vi "DetectorTest_MainV11.vi"() -> ()   [LabVIEW 2012]
uses:
  Detector IV/SMU Settings.ctl
  <vilib>/Utility/file.llb/Write To Spreadsheet File (string).vi
  <vilib>/Utility/file.llb/Read From Spreadsheet File (string).vi
  <vilib>/Utility/file.llb/Read From Spreadsheet File (DBL).vi
  <vilib>/Analysis/NI_AALBase.lvlib
panel:
  in  "make common recipe":bool
  in  "select preset recipe":bool
  in  "Detector Measurement Recipe":T1={"Start Voltage"=0.0, "End Voltage"=0.0, "Number of Points"=0.0, "I compliance ma"=0.0, "Sweep Delay s"=0.0, "Direction"="", "Comments"="testing", "Common Recipe"=0.0, "Test Setup"=0.0, "Measurement Recipe ID"=0.0}
  in  "Current Session":timestamp=timestamp(3388091786.578125 s since 1904-01-01)
  in  "new sesh":bool
  out "RecipeID":string="58"
  in  "Sweep Direction (Keysight)":i32(ring) items=["Up", "Down"]
  in  "Auto Adjust Compliance?":bool
  out "Auto Temp Counter":i32
  out "iteration":i32
  in  "Temp Data":T2={"Ambient Temperature"=20.38176242851337, "Chuck Set Temperature"=35.0} {"Chuck Set Temperature" format="%#.1g"; "Ambient Temperature" format="%#.1g"}
  in  "Wafer Info 3":T3={"Cell Name (Automatic)"="Open_Diode_1000", "Package"="", "Coating"="FOR_AIR", "Comment"="IV test for lot 371", "Flash Setup"="5500_99_03p5", "Hrs under test"=0.0}
  out "TempCounter":i32
  out "WaferCounter":i32
  in  "Profile Z":bool
  in  "Load Wafer":bool
  out "Raw Test Skipped":bool=TRUE
  out "device name w skip":string="Open_Diode_1000(skip)"
  in  "4-wire":bool
  out "Laser Counter":i32
  out "Output Power (mW)":dbl
  out "Counter":i32
  out "NameList":string[](array[string])
  in  "Wafer Info Flash 2":T4={"Cell Name"="5500_130_05", "Package"="", "Coating"="", "LRC?"=enum."J2", "Comment"="", "Hours Under Test"=0.0}
  in  "Parameters Flash 2":T5 {"Voc" format="%#_4g"; "Isc" format="%#_4g"; "FF" format="%#_4g"; "Imax" format="%#_4g"; "Vmax" format="%#_4g"; "Pmax" format="%#_4g"; "Itest" format="%#_4g"}
  in  "Wafer Info Flash":T4={"Cell Name"="Open_Diode_1000", "Package"="", "Coating"="", "LRC?"=enum."J2", "Comment"="", "Hours Under Test"=0.0}
  in  "Parameters Flash":T5={"Voc"=0.0, "Isc"=0.0, "FF"=0.0, "Vtest"=0.0, "Imax"=0.0, "Vmax"=0.0, "Pmax"=0.0, "Itest"=0.0, "Efficiency"=0.0, "Incident Power"=5.674, "Power Density (W/cm^2)"=0.6679328011361159, "Cell Area (cm²)"=849486.6535, "Number of AM1.5D Suns"=0.0, "Input Current (mA)"=40.0, "Equivalent 1 sun Jsc"=0.0} {"Voc" format="%#_4g"; "Isc" format="%#_4g"; "FF" format="%#_4g"; "Imax" format="%#_4g"; "Vmax" format="%#_4g"; "Pmax" format="%#_4g"; "Itest" format="%#_4g"}
  out "RawData file":path=path "C:/Users/Flash/Desktop/Data/Detector test data/SJC_ENG_371_4-GaAs/A-3719-2-A/Raw Data/A-3719-2-A_Open_Diode_1000_20180913075240.csv"
  out "Fine Cell Clusters":T6(array[cluster])=[{"Cell Name"="Open_Diode_1000", "X-coord"=46800.0, "Y-coord"=22950.0, "Area"=849486.6535, "Grid Shadowing"=0.0, "Xdim"=500.0, "Ydim"=500.0, "Mesa Area"=785398.1634}]
  out "Selected Data":cluster{dbl[], dbl[]}={[nan, nan, nan, nan, nan, nan, nan, nan, nan, nan, nan, nan, nan, nan, nan, nan, nan, nan, nan, nan, nan, nan, nan, nan, nan, nan, nan, nan, nan, nan, nan, nan, nan, nan, nan, nan, nan, nan, nan, nan, nan, nan, nan, nan, nan, nan, nan, nan, nan, nan, nan, nan, nan, nan, nan, nan, nan, nan, nan, nan, nan, nan, nan, nan, nan, nan, nan, nan, nan, nan, nan, nan, nan, nan, nan, nan, nan, nan, nan, nan, nan, nan, nan, nan], [nan, nan, nan, nan, nan, nan, nan, nan, nan, nan, nan, nan, nan, nan, nan, nan, nan, nan, nan, nan, nan, nan, nan, nan, nan, nan, nan, nan, nan, nan, nan, nan, nan, nan, nan, nan, nan, nan, nan, nan, nan, nan, nan, nan, nan, nan, nan, nan, nan, nan, nan, nan, nan, nan, nan, nan, nan, nan, nan, nan, nan, nan, nan, nan, nan, nan, nan, nan, nan, nan, nan, nan, nan, nan, nan, nan, nan, nan, nan, nan, nan, nan, nan, nan]}
  in  "Test Results 2":T7
  in  "Session Info 2":T8={"V set"=-1.0, "I compliance"=0.001, "J set"=0.01, "I set"=0.0, "V compliance"=1.0, "Laser Power (mW)"=0.0, "TestID"=0, "Session Time"=timestamp(0 s since 1904-01-01), "Operator"="Radek"} {"V compliance" format="%#_6f"; "I compliance" format="%#_6e"}
  in  "Die Info 2":T9={"Device Name"="", "ActiveArea_um2"=3848.451, "MesaArea_um2"=3848.451, "x"=0.0, "y"=0.0}
  in  "Wafer Info 2":T10
  in  "Test Results":T7={"I meas"=-1.83245e-12, "V meas"=6.01176, "Time"=timestamp(3619695820.3512325 s since 1904-01-01)}
  in  "Session Info":T8={"V set"=-6.0, "I compliance"=0.001, "J set"=0.01, "I set"=1.9634954079999997e-05, "V compliance"=6.0, "Laser Power (mW)"=0.0, "TestID"=1794, "Session Time"=timestamp(3619695160.866512 s since 1904-01-01), "Operator"="sswifter"} {"V compliance" format="%#_6f"; "I compliance" format="%#_6e"}
  in  "Die Info":T9={"Device Name"="Open_Diode_1000", "ActiveArea_um2"=849486.6535, "MesaArea_um2"=785398.1634, "x"=26800.0, "y"=72950.0}
  in  "Wafer Info":T10={"Wafer Name"="A-3719-2-A", "Scribe"="BJ325-089", "Mask"="PH001", "Lot"="SJC_ENG_371_4-GaAs"}
  in  "Name Array":string[](array[string])=["Wafer name", "Scribe", "Mask", "Lot", "Device name", "Active Area", "Mesa Area", "x", "y", "Imeas", "Vmeas", "Time", "Vset", "Icomp", "Jset", "Iset", "Vcomp", "Laser Power", "TestID", "SessionTime", "Operator", "Selected"]
  in  "TestID file":path=path "C:/Users/Flash/Documents/GitHub/labview/Detector IV/rawtest_log.csv"
  in  "update wafer":bool
  in  "Lot":string="SJC_ENG_382_4-GaAs"
  in  "Laser Current (mA)":dbl
  in  "Device Name":string="Open_Diode_3000"
  in  "Scribe":string="BP769-030XT"
  in  "MesaArea_um2":dbl=7068583.471
  out "Status":string="idle"
  out "error out":errorcluster
  in  "error in (no error)":errorcluster
  out "Manaul Plot 1":cluster{"V manual":dbl[], dbl[]}[](array[cluster])=[{"V manual"=[-0.1, -0.089741, -0.07949, -0.06923, -0.05897, -0.04872, -0.03846, -0.02821, -0.017951, -0.00769, 0.00256, 0.012819, 0.02308, 0.03333, 0.043589, 0.05385, 0.0641, 0.074359, 0.084619, 0.09487, 0.10513, 0.115379, 0.125639, 0.135899, 0.14615, 0.156409, 0.16667, 0.176919, 0.187179, 0.19744, 0.207691, 0.217949, 0.22821, 0.23846, 0.248719], [2.22891e-05, 1.84968e-05, 1.52529e-05, 1.24377e-05, 1.00378e-05, 7.9393e-06, 6.043e-06, 4.31347e-06, 2.71019e-06, 1.17492e-06, 3.32763e-07, 1.84722e-06, 3.41691e-06, 5.05009e-06, 6.8287e-06, 8.72018e-06, 1.07805e-05, 1.3036e-05, 1.55303e-05, 1.81749e-05, 2.11963e-05, 2.4467e-05, 2.80104e-05, 3.19022e-05, 3.6041e-05, 4.04887e-05, 4.53187e-05, 5.05479e-05, 5.60681e-05, 6.20483e-05, 6.8299e-05, 7.49314e-05, 8.20298e-05, 8.95166e-05, 9.72544e-05]}, {"V manual"=[-0.1, nan, nan, nan, nan, nan, nan, nan, nan, nan, nan, nan, nan, nan, nan, nan, nan, nan, nan, nan, nan, nan, nan, nan, nan, nan, nan, nan, nan, nan, nan, nan, nan, nan, nan, nan, nan, nan, nan, nan], [2.2117733333333333e-05, nan, nan, nan, nan, nan, nan, nan, nan, nan, nan, nan, nan, nan, nan, nan, nan, nan, nan, nan, nan, nan, nan, nan, nan, nan, nan, nan, nan, nan, nan, nan, nan, nan, nan, nan, nan, nan, nan, nan]}, {"V manual"=[0.23860433333333333, nan, nan, nan, nan, nan, nan, nan, nan, nan, nan, nan, nan, nan, nan, nan, nan, nan, nan, nan, nan, nan, nan, nan, nan, nan, nan, nan, nan, nan, nan, nan, nan, nan, nan, nan, nan, nan, nan, nan], [7.068583470999999e-05, nan, nan, nan, nan, nan, nan, nan, nan, nan, nan, nan, nan, nan, nan, nan, nan, nan, nan, nan, nan, nan, nan, nan, nan, nan, nan, nan, nan, nan, nan, nan, nan, nan, nan, nan, nan, nan, nan, nan]}]
  out "Manual Plot 0":cluster{"V manual":dbl[], "I manual":dbl[]}[](array[cluster])=[{"V manual"=[-0.1, -0.089741, -0.07949, -0.06923, -0.05897, -0.04872, -0.03846, -0.02821, -0.017951, -0.00769, 0.00256, 0.012819, 0.02308, 0.03333, 0.043589, 0.05385, 0.0641, 0.074359, 0.084619, 0.09487, 0.10513, 0.115379, 0.125639, 0.135899, 0.14615, 0.156409, 0.16667, 0.176919, 0.187179, 0.19744, 0.207691, 0.217949, 0.22821, 0.23846, 0.248719], "I manual"=[-2.22891e-05, -1.84968e-05, -1.52529e-05, -1.24377e-05, -1.00378e-05, -7.9393e-06, -6.043e-06, -4.31347e-06, -2.71019e-06, -1.17492e-06, 3.32763e-07, 1.84722e-06, 3.41691e-06, 5.05009e-06, 6.8287e-06, 8.72018e-06, 1.07805e-05, 1.3036e-05, 1.55303e-05, 1.81749e-05, 2.11963e-05, 2.4467e-05, 2.80104e-05, 3.19022e-05, 3.6041e-05, 4.04887e-05, 4.53187e-05, 5.05479e-05, 5.60681e-05, 6.20483e-05, 6.8299e-05, 7.49314e-05, 8.20298e-05, 8.95166e-05, 9.72544e-05]}, {"V manual"=[-0.1, nan, nan, nan, nan, nan, nan, nan, nan, nan, nan, nan, nan, nan, nan, nan, nan, nan, nan, nan, nan, nan, nan, nan, nan, nan, nan, nan, nan, nan, nan, nan, nan, nan, nan, nan, nan, nan, nan, nan], "I manual"=[-2.2117733333333333e-05, nan, nan, nan, nan, nan, nan, nan, nan, nan, nan, nan, nan, nan, nan, nan, nan, nan, nan, nan, nan, nan, nan, nan, nan, nan, nan, nan, nan, nan, nan, nan, nan, nan, nan, nan, nan, nan, nan, nan]}, {"V manual"=[0.23860433333333333, nan, nan, nan, nan, nan, nan, nan, nan, nan, nan, nan, nan, nan, nan, nan, nan, nan, nan, nan, nan, nan, nan, nan, nan, nan, nan, nan, nan, nan, nan, nan, nan, nan, nan, nan, nan, nan, nan, nan], "I manual"=[7.068583470999999e-05, nan, nan, nan, nan, nan, nan, nan, nan, nan, nan, nan, nan, nan, nan, nan, nan, nan, nan, nan, nan, nan, nan, nan, nan, nan, nan, nan, nan, nan, nan, nan, nan, nan, nan, nan, nan, nan, nan, nan]}]
  in  "Reset 1st die":bool
  in  "Sweep Settings":T11={"Channel"=enum."Channel A", "Vstart"=-0.1, "Vend"=0.3, "# of points"=40, "NPLC"=1.0, "I compliance"=0.0001, "Delay ms"=100.0}
  in  "Reset xy":bool
  out "current y":i32
  out "current x":i32=10000
  in  "sweep delay ms":dbl=100.0
  in  "I compliance sweep":dbl=0.0001
  in  "points":u16=80
  in  "V end":dbl=1.0
  in  "V start":dbl=-5.0
  in  "Repeat Vf":u32=3
  out "I set":dbl=7.068583470999999e-05
  in  "V compliance":dbl=0.5 format="%#_6f"
  in  "Vf delay ms":dbl=100.0
  in  "J set A/cm2":dbl=0.001
  in  "Repeat Id":u32=5
  in  "I compliance":dbl=0.001 format="%#_6e"
  in  "Id delay ms":dbl=500.0
  in  "V set":dbl=-0.1
  out "Vmeas Settings":T12={"Channel"=enum."Channel A", "Vset"=7.068583470999999e-05, "NPLC"=1.0, "I compliance"=0.3, "Repeat time"=1, "Delay ms"=100.0, "4-wire"=FALSE}
  out "Imeas Settings":T12={"Channel"=enum."Channel A", "Vset"=-0.1, "NPLC"=1.0, "I compliance"=0.001, "Repeat time"=5, "Delay ms"=500.0, "4-wire"=FALSE}
  out "Array of Cell Data Clusters":T13(array[cluster])=[{"Cell Name"="Open_Diode_3000", "X-coord"=0.0, "Y-coord"=0.0, "Area"=7258335.667, "Grid Shadowing"=0.0, "Ydim"=1500.0, "Xdim"=1500.0, "Meas Area"=7068583.471}, {"Cell Name"="Open_Diode_3000", "X-coord"=10000.0, "Y-coord"=0.0, "Area"=7258335.667, "Grid Shadowing"=0.0, "Ydim"=1500.0, "Xdim"=1500.0, "Meas Area"=7068583.471}, {"Cell Name"="Open_Diode_3000", "X-coord"=20000.0, "Y-coord"=0.0, "Area"=7258335.667, "Grid Shadowing"=0.0, "Ydim"=1500.0, "Xdim"=1500.0, "Meas Area"=7068583.471}, {"Cell Name"="Open_Diode_3000", "X-coord"=30000.0, "Y-coord"=0.0, "Area"=7258335.667, "Grid Shadowing"=0.0, "Ydim"=1500.0, "Xdim"=1500.0, "Meas Area"=7068583.471}, {"Cell Name"="Open_Diode_3000", "X-coord"=-10000.0, "Y-coord"=10000.0, "Area"=7258335.667, "Grid Shadowing"=0.0, "Ydim"=1500.0, "Xdim"=1500.0, "Meas Area"=7068583.471}, {"Cell Name"="Open_Diode_3000", "X-coord"=0.0, "Y-coord"=10000.0, "Area"=7258335.667, "Grid Shadowing"=0.0, "Ydim"=1500.0, "Xdim"=1500.0, "Meas Area"=7068583.471}, {"Cell Name"="Open_Diode_3000", "X-coord"=10000.0, "Y-coord"=10000.0, "Area"=7258335.667, "Grid Shadowing"=0.0, "Ydim"=1500.0, "Xdim"=1500.0, "Meas Area"=7068583.471}, {"Cell Name"="Open_Diode_3000", "X-coord"=40000.0, "Y-coord"=10000.0, "Area"=7258335.667, "Grid Shadowing"=0.0, "Ydim"=1500.0, "Xdim"=1500.0, "Meas Area"=7068583.471}, {"Cell Name"="Open_Diode_3000", "X-coord"=-20000.0, "Y-coord"=20000.0, "Area"=7258335.667, "Grid Shadowing"=0.0, "Ydim"=1500.0, "Xdim"=1500.0, "Meas Area"=7068583.471}, {"Cell Name"="Open_Diode_3000", "X-coord"=-10000.0, "Y-coord"=20000.0, "Area"=7258335.667, "Grid Shadowing"=0.0, "Ydim"=1500.0, "Xdim"=1500.0, "Meas Area"=7068583.471}, {"Cell Name"="Open_Diode_3000", "X-coord"=10000.0, "Y-coord"=20000.0, "Area"=7258335.667, "Grid Shadowing"=0.0, "Ydim"=1500.0, "Xdim"=1500.0, "Meas Area"=7068583.471}, {"Cell Name"="Open_Diode_3000", "X-coord"=20000.0, "Y-coord"=20000.0, "Area"=7258335.667, "Grid Shadowing"=0.0, "Ydim"=1500.0, "Xdim"=1500.0, "Meas Area"=7068583.471}, {"Cell Name"="Open_Diode_3000", "X-coord"=40000.0, "Y-coord"=20000.0, "Area"=7258335.667, "Grid Shadowing"=0.0, "Ydim"=1500.0, "Xdim"=1500.0, "Meas Area"=7068583.471}, {"Cell Name"="Open_Diode_3000", "X-coord"=50000.0, "Y-coord"=20000.0, "Area"=7258335.667, "Grid Shadowing"=0.0, "Ydim"=1500.0, "Xdim"=1500.0, "Meas Area"=7068583.471}, {"Cell Name"="Open_Diode_3000", "X-coord"=-20000.0, "Y-coord"=30000.0, "Area"=7258335.667, "Grid Shadowing"=0.0, "Ydim"=1500.0, "Xdim"=1500.0, "Meas Area"=7068583.471}, {"Cell Name"="Open_Diode_3000", "X-coord"=-10000.0, "Y-coord"=30000.0, "Area"=7258335.667, "Grid Shadowing"=0.0, "Ydim"=1500.0, "Xdim"=1500.0, "Meas Area"=7068583.471}, {"Cell Name"="Open_Diode_3000", "X-coord"=20000.0, "Y-coord"=30000.0, "Area"=7258335.667, "Grid Shadowing"=0.0, "Ydim"=1500.0, "Xdim"=1500.0, "Meas Area"=7068583.471}, {"Cell Name"="Open_Diode_3000", "X-coord"=30000.0, "Y-coord"=30000.0, "Area"=7258335.667, "Grid Shadowing"=0.0, "Ydim"=1500.0, "Xdim"=1500.0, "Meas Area"=7068583.471}, {"Cell Name"="Open_Diode_3000", "X-coord"=40000.0, "Y-coord"=30000.0, "Area"=7258335.667, "Grid Shadowing"=0.0, "Ydim"=1500.0, "Xdim"=1500.0, "Meas Area"=7068583.471}, {"Cell Name"="Open_Diode_3000", "X-coord"=50000.0, "Y-coord"=30000.0, "Area"=7258335.667, "Grid Shadowing"=0.0, "Ydim"=1500.0, "Xdim"=1500.0, "Meas Area"=7068583.471}, {"Cell Name"="Open_Diode_3000", "X-coord"=-20000.0, "Y-coord"=40000.0, "Area"=7258335.667, "Grid Shadowing"=0.0, "Ydim"=1500.0, "Xdim"=1500.0, "Meas Area"=7068583.471}, {"Cell Name"="Open_Diode_3000", "X-coord"=-10000.0, "Y-coord"=40000.0, "Area"=7258335.667, "Grid Shadowing"=0.0, "Ydim"=1500.0, "Xdim"=1500.0, "Meas Area"=7068583.471}, {"Cell Name"="Open_Diode_3000", "X-coord"=0.0, "Y-coord"=40000.0, "Area"=7258335.667, "Grid Shadowing"=0.0, "Ydim"=1500.0, "Xdim"=1500.0, "Meas Area"=7068583.471}, {"Cell Name"="Open_Diode_3000", "X-coord"=10000.0, "Y-coord"=40000.0, "Area"=7258335.667, "Grid Shadowing"=0.0, "Ydim"=1500.0, "Xdim"=1500.0, "Meas Area"=7068583.471}, {"Cell Name"="Open_Diode_3000", "X-coord"=40000.0, "Y-coord"=40000.0, "Area"=7258335.667, "Grid Shadowing"=0.0, "Ydim"=1500.0, "Xdim"=1500.0, "Meas Area"=7068583.471}, {"Cell Name"="Open_Diode_3000", "X-coord"=50000.0, "Y-coord"=40000.0, "Area"=7258335.667, "Grid Shadowing"=0.0, "Ydim"=1500.0, "Xdim"=1500.0, "Meas Area"=7068583.471}, {"Cell Name"="Open_Diode_3000", "X-coord"=-20000.0, "Y-coord"=50000.0, "Area"=7258335.667, "Grid Shadowing"=0.0, "Ydim"=1500.0, "Xdim"=1500.0, "Meas Area"=7068583.471}, {"Cell Name"="Open_Diode_3000", "X-coord"=-10000.0, "Y-coord"=50000.0, "Area"=7258335.667, "Grid Shadowing"=0.0, "Ydim"=1500.0, "Xdim"=1500.0, "Meas Area"=7068583.471}, {"Cell Name"="Open_Diode_3000", "X-coord"=10000.0, "Y-coord"=50000.0, "Area"=7258335.667, "Grid Shadowing"=0.0, "Ydim"=1500.0, "Xdim"=1500.0, "Meas Area"=7068583.471}, {"Cell Name"="Open_Diode_3000", "X-coord"=20000.0, "Y-coord"=50000.0, "Area"=7258335.667, "Grid Shadowing"=0.0, "Ydim"=1500.0, "Xdim"=1500.0, "Meas Area"=7068583.471}, {"Cell Name"="Open_Diode_3000", "X-coord"=40000.0, "Y-coord"=50000.0, "Area"=7258335.667, "Grid Shadowing"=0.0, "Ydim"=1500.0, "Xdim"=1500.0, "Meas Area"=7068583.471}, {"Cell Name"="Open_Diode_3000", "X-coord"=50000.0, "Y-coord"=50000.0, "Area"=7258335.667, "Grid Shadowing"=0.0, "Ydim"=1500.0, "Xdim"=1500.0, "Meas Area"=7068583.471}, {"Cell Name"="Open_Diode_3000", "X-coord"=-10000.0, "Y-coord"=60000.0, "Area"=7258335.667, "Grid Shadowing"=0.0, "Ydim"=1500.0, "Xdim"=1500.0, "Meas Area"=7068583.471}, {"Cell Name"="Open_Diode_3000", "X-coord"=20000.0, "Y-coord"=60000.0, "Area"=7258335.667, "Grid Shadowing"=0.0, "Ydim"=1500.0, "Xdim"=1500.0, "Meas Area"=7068583.471}, {"Cell Name"="Open_Diode_3000", "X-coord"=30000.0, "Y-coord"=60000.0, "Area"=7258335.667, "Grid Shadowing"=0.0, "Ydim"=1500.0, "Xdim"=1500.0, "Meas Area"=7068583.471}, {"Cell Name"="Open_Diode_3000", "X-coord"=40000.0, "Y-coord"=60000.0, "Area"=7258335.667, "Grid Shadowing"=0.0, "Ydim"=1500.0, "Xdim"=1500.0, "Meas Area"=7068583.471}, {"Cell Name"="Open_Diode_3000", "X-coord"=0.0, "Y-coord"=70000.0, "Area"=7258335.667, "Grid Shadowing"=0.0, "Ydim"=1500.0, "Xdim"=1500.0, "Meas Area"=7068583.471}, {"Cell Name"="Open_Diode_3000", "X-coord"=10000.0, "Y-coord"=70000.0, "Area"=7258335.667, "Grid Shadowing"=0.0, "Ydim"=1500.0, "Xdim"=1500.0, "Meas Area"=7068583.471}, {"Cell Name"="Open_Diode_3000", "X-coord"=20000.0, "Y-coord"=70000.0, "Area"=7258335.667, "Grid Shadowing"=0.0, "Ydim"=1500.0, "Xdim"=1500.0, "Meas Area"=7068583.471}, {"Cell Name"="Open_Diode_3000", "X-coord"=30000.0, "Y-coord"=70000.0, "Area"=7258335.667, "Grid Shadowing"=0.0, "Ydim"=1500.0, "Xdim"=1500.0, "Meas Area"=7068583.471}]
  in  "stop":bool
  in  "ActiveArea_um2":dbl=7258335.667
  in  "NPLC":dbl=1.0
  in  "Operator":string(combo)="tbilir"
  in  "Mask":string="PH001"
  in  "Wafer Name":string="A-3820-3-A"
  in  "Tab Control":T14(tab)
  in  "First Wafer Loaded?":bool
  in  "begin lot test":bool
  in  "Desired Wafer Name":string
  in  "Wafer List":i32(listbox)=-1
  in  "Add to wafer list":bool
  in  "Remove from wafer list":bool
  in  "Clear wafer list":bool
  in  "Generate Report":bool
  in  "Only Raw Test":bool
  in  "Clear Laser List":bool
  in  "Remove from Laser List":bool
  in  "Add to Laser":bool
  in  "Desired Current (mA)":dbl=40.0
  in  "Laser List":i32(listbox)=-1
  in  "Start auto":bool
  in  "Clear List":bool
  in  "Refresh Device":bool
  in  "Mask Name":string
  in  "Remove from List":bool
  in  "Add to list":bool
  in  "Available Device Name":string(combo)="Open_Diode_1000"
  in  "Test List":i32(listbox)=-1
  in  "Mask File all":path=path "C:/Users/Flash/Desktop/Mask Files/PH001 Detector GSG/PH001_Detector Aligner mask map file _ full top_open top 10_open top 5 diodes.csv"
  in  "Skip Raw Test?":bool
  in  "Test description":string="IV test for lot 371"
  in  "Clear temp list Auto":bool
  in  "Remove from Temp Auto":bool
  in  "Add to Temp Auto":bool
  in  "Auto Temp Set":dbl=25.0
  in  "Auto Temperature List":i32(listbox)=-1
  in  "Manual_Test":bool
  in  "Manual IV Plot settting":enum32{"Linear plot", "Log plot"}(radio)
  out "Vmeas manual":dbl=0.23860433333333333
  out "Imeas manual":dbl=-2.2117733333333333e-05
  out "Iarray manual":dbl[](array[numeric])=[-2.22891e-05, -1.84968e-05, -1.52529e-05, -1.24377e-05, -1.00378e-05, -7.9393e-06, -6.043e-06, -4.31347e-06, -2.71019e-06, -1.17492e-06, 3.32763e-07, 1.84722e-06, 3.41691e-06, 5.05009e-06, 6.8287e-06, 8.72018e-06, 1.07805e-05, 1.3036e-05, 1.55303e-05, 1.81749e-05, 2.11963e-05, 2.4467e-05, 2.80104e-05, 3.19022e-05, 3.6041e-05, 4.04887e-05, 4.53187e-05, 5.05479e-05, 5.60681e-05, 6.20483e-05, 6.8299e-05, 7.49314e-05, 8.20298e-05, 8.95166e-05, 9.72544e-05]
  out "Varray manual":dbl[](array[numeric])=[-0.1, -0.089741, -0.07949, -0.06923, -0.05897, -0.04872, -0.03846, -0.02821, -0.017951, -0.00769, 0.00256, 0.012819, 0.02308, 0.03333, 0.043589, 0.05385, 0.0641, 0.074359, 0.084619, 0.09487, 0.10513, 0.115379, 0.125639, 0.135899, 0.14615, 0.156409, 0.16667, 0.176919, 0.187179, 0.19744, 0.207691, 0.217949, 0.22821, 0.23846, 0.248719]
  out "y target":i32
  out "x target":i32=10000
  in  "Die Number":u16(ring)=1 items=["0", "1", "2", "3", "4", "5", "6", "7", "8", "9", "10", "11", "12", "13", "14", "15", "16", "17", "18", "19", "20", "21", "22", "23", "24", "25", "26", "27", "28", "29", "30", "31", "32", "33", "34", "35", "36", "37", "38", "39", "40", "41", "42", "43", "44", "45", "46", "47", "48", "49", "50", "51", "52", "53", "54", "55", "56", "57", "58", "59", "60", "61", "62", "63", "64", "65", "66", "67", "68", "69", "70", "71", "72", "73", "74", "75", "76", "77", "78", "79", "80", "81", "82", "83", "84", "85"]
  in  "load file":bool
  in  "Move to":bool
  in  "Mask File Manual":path=path "C:/Users/Flash/Desktop/Mask Files/PH001 Detector GSG/PH001_Detector Aligner mask map file _ full top_open top 10_open top 5 diodes_Open_Diode_3000.csv"
  out "Manual IV":cluster{"V manual":dbl[], "I manual":dbl[]}[](graph)=[{"V manual"=[-0.1, -0.089741, -0.07949, -0.06923, -0.05897, -0.04872, -0.03846, -0.02821, -0.017951, -0.00769, 0.00256, 0.012819, 0.02308, 0.03333, 0.043589, 0.05385, 0.0641, 0.074359, 0.084619, 0.09487, 0.10513, 0.115379, 0.125639, 0.135899, 0.14615, 0.156409, 0.16667, 0.176919, 0.187179, 0.19744, 0.207691, 0.217949, 0.22821, 0.23846, 0.248719], "I manual"=[-2.22891e-05, -1.84968e-05, -1.52529e-05, -1.24377e-05, -1.00378e-05, -7.9393e-06, -6.043e-06, -4.31347e-06, -2.71019e-06, -1.17492e-06, 3.32763e-07, 1.84722e-06, 3.41691e-06, 5.05009e-06, 6.8287e-06, 8.72018e-06, 1.07805e-05, 1.3036e-05, 1.55303e-05, 1.81749e-05, 2.11963e-05, 2.4467e-05, 2.80104e-05, 3.19022e-05, 3.6041e-05, 4.04887e-05, 4.53187e-05, 5.05479e-05, 5.60681e-05, 6.20483e-05, 6.8299e-05, 7.49314e-05, 8.20298e-05, 8.95166e-05, 9.72544e-05]}, {"V manual"=[-0.1, nan, nan, nan, nan, nan, nan, nan, nan, nan, nan, nan, nan, nan, nan, nan, nan, nan, nan, nan, nan, nan, nan, nan, nan, nan, nan, nan, nan, nan, nan, nan, nan, nan, nan, nan, nan, nan, nan, nan], "I manual"=[-2.2117733333333333e-05, nan, nan, nan, nan, nan, nan, nan, nan, nan, nan, nan, nan, nan, nan, nan, nan, nan, nan, nan, nan, nan, nan, nan, nan, nan, nan, nan, nan, nan, nan, nan, nan, nan, nan, nan, nan, nan, nan, nan]}, {"V manual"=[0.23860433333333333, nan, nan, nan, nan, nan, nan, nan, nan, nan, nan, nan, nan, nan, nan, nan, nan, nan, nan, nan, nan, nan, nan, nan, nan, nan, nan, nan, nan, nan, nan, nan, nan, nan, nan, nan, nan, nan, nan, nan], "I manual"=[7.068583470999999e-05, nan, nan, nan, nan, nan, nan, nan, nan, nan, nan, nan, nan, nan, nan, nan, nan, nan, nan, nan, nan, nan, nan, nan, nan, nan, nan, nan, nan, nan, nan, nan, nan, nan, nan, nan, nan, nan, nan, nan]}]
  in  "Measure 2 Point?":bool=TRUE
  in  "Manual Test Comments":string="IV test for lot 371"
  in  "Load raw":bool
  in  "Select":bool
  in  "Number Select":u16=10
  in  "Vmax":dbl=0.285
  in  "Vmin":dbl=0.05
  out "Test FileName":string="A-3719-2-A_Open_Diode_1000_20180913075240.csv"
  out "RawTest ID":u32=2029
  out "Progress":u8(slide)=99 scale=0.0..100.0
  out "Current Device":u32=84
  out "Total Device":u32=84
  out "V meas":dbl[](array[numeric])=[6.01142, 6.01054, 6.01089, 0.000137925, 6.01222, 6.01216, 6.01145, 6.01193, 6.0103, 6.01103, 6.01162, 6.01132, 6.01127, 6.01137, 6.01132, 6.01125, 6.01108, 6.01134, 6.01154, 6.01135, 6.01146, 6.01204, 6.01111, 6.01101, 6.01053, 6.01143, 6.01152, 6.01128, 6.00993, 6.00994, 6.01042, 3.58707, 6.01175, 6.01164, 6.01056, 6.01166, 6.01073, 6.01098, 6.01142, 6.01026, 6.01071, 6.01116, 6.01174, 6.01214, 6.01026, 6.01093, 5.99486, 6.01138, 6.01091, 6.01133, 6.01086, 6.01094, 6.01192, 6.01232, 6.01069, 6.01162, 6.01233, 6.01184, 6.0022, 5.17964, 6.01156, 6.01223, 6.01107, 6.0102, 6.0108, 6.01164, 5.75188, 5.06441, 6.01144, 6.01129, 6.01161, 6.01159, 6.01096, 5.61419, 5.16536, 6.01197, 6.01142, 6.01186, 6.01133, 6.01132, 6.01119, 6.01113, 5.83632, 6.01176]
  out "I meas":dbl[](array[numeric])=[-3.868033999999999e-11, -1.2052780000000002e-09, -6.028065999999999e-11, -0.0009999796, -3.0170019999999996e-11, -4.752688e-11, -4.8625459999999994e-11, -3.7159980000000005e-11, -1.7203160000000002e-07, -2.00883e-08, -7.974548e-11, -3.897576e-11, -3.555112e-11, -2.188194e-08, -5.2771619999999994e-11, -2.9935519999999994e-11, -3.295828e-11, -5.707007999999999e-08, -4.796104e-07, -2.002028e-08, -7.080146e-08, -4.18e-11, -2.108774e-11, -4.09959e-11, -4.424556e-11, -3.3264100000000003e-09, -2.0351338000000002e-10, -6.144901999999999e-09, -4.3002719999999993e-11, -3.898936e-09, -2.0389360000000002e-11, -2.049748e-08, -6.527374000000001e-10, -1.0336196000000001e-10, -2.697004e-11, -3.376518e-08, -6.171924e-11, -2.02069e-10, -1.200538e-09, -2.8179300000000003e-11, -6.537938e-10, -5.153115999999999e-11, -2.8508420000000003e-09, -7.534774e-07, -2.636916e-07, -1.446754e-09, -9.464432000000001e-11, -1.0602588000000001e-10, -4.217728e-11, -7.227086e-08, -3.990094e-11, -2.7389038000000002e-11, -1.90881e-07, -2.2892700000000004e-12, -4.745506e-08, -4.579318e-11, -4.5842860000000003e-11, -5.953868e-11, -3.758154e-11, -4.4363539999999995e-09, -7.143562e-11, -1.397812e-10, -7.11463e-11, -5.56664e-11, -2.6296820000000003e-08, -1.1582659999999999e-07, -2.317642e-11, -5.807276000000001e-11, -2.17813e-12, -5.7970201999999995e-11, -6.71486e-11, -8.667722000000001e-12, 3.2483739999999993e-12, -6.306573999999999e-11, -8.307524e-11, -2.4324079999999998e-12, -2.795726e-12, -2.185576e-12, -2.0225460000000002e-12, -2.122472e-12, -1.6340760000000001e-06, -2.5727129999999997e-06, -3.269066e-11, -1.83245e-12]
  in  "RawData Save Path":path=path "C:/Users/Flash/Desktop/Data/Detector test data"
  in  "StartRaw":bool
  out "Vforward hist":T15(graph)={"X Values"=[0.30074752875, 0.90196673625, 1.5031859437500001, 2.10440515125, 2.70562435875, 3.3068435662500004, 3.90806277375, 4.50928198125, 5.110501188750001, 5.7117203962500005], "Histogram: h(x)"=[1, 0, 0, 0, 0, 1, 0, 0, 3, 79]}
  out "Idark hist":T15(graph)={"X Values"=[-0.0009499806198375813, -0.0008499826595127439, -0.0007499846991879066, -0.0006499867388630691, -0.0005499887785382317, -0.0004499908182133943, -0.0003499928578885569, -0.0002499948975637195, -0.0001499969372388821, -4.99989769140447e-05], "Histogram: h(x)"=[1, 0, 0, 0, 0, 0, 0, 0, 0, 83]}
  in  "Mask File Raw":path=path "C:/Users/Flash/Desktop/Mask Files/PH001 Detector GSG/PH001_Detector Aligner mask map file _ full top_open top 10_open top 5 diodes_Open_Diode_3000.csv"
  out "Spec Plot":cluster{"V meas":dbl[], "I meas":dbl[]}[](graph)=[{"V meas"=[6.01142, 6.01054, 6.01089, 0.000137925, 6.01222, 6.01216, 6.01145, 6.01193, 6.0103, 6.01103, 6.01162, 6.01132, 6.01127, 6.01137, 6.01132, 6.01125, 6.01108, 6.01134, 6.01154, 6.01135, 6.01146, 6.01204, 6.01111, 6.01101, 6.01053, 6.01143, 6.01152, 6.01128, 6.00993, 6.00994, 6.01042, 3.58707, 6.01175, 6.01164, 6.01056, 6.01166, 6.01073, 6.01098, 6.01142, 6.01026, 6.01071, 6.01116, 6.01174, 6.01214, 6.01026, 6.01093, 5.99486, 6.01138, 6.01091, 6.01133, 6.01086, 6.01094, 6.01192, 6.01232, 6.01069, 6.01162, 6.01233, 6.01184, 6.0022, 5.17964, 6.01156, 6.01223, 6.01107, 6.0102, 6.0108, 6.01164, 5.75188, 5.06441, 6.01144, 6.01129, 6.01161, 6.01159, 6.01096, 5.61419, 5.16536, 6.01197, 6.01142, 6.01186, 6.01133, 6.01132, 6.01119, 6.01113, 5.83632, 6.01176], "I meas"=[-3.868033999999999e-11, -1.2052780000000002e-09, -6.028065999999999e-11, -0.0009999796, -3.0170019999999996e-11, -4.752688e-11, -4.8625459999999994e-11, -3.7159980000000005e-11, -1.7203160000000002e-07, -2.00883e-08, -7.974548e-11, -3.897576e-11, -3.555112e-11, -2.188194e-08, -5.2771619999999994e-11, -2.9935519999999994e-11, -3.295828e-11, -5.707007999999999e-08, -4.796104e-07, -2.002028e-08, -7.080146e-08, -4.18e-11, -2.108774e-11, -4.09959e-11, -4.424556e-11, -3.3264100000000003e-09, -2.0351338000000002e-10, -6.144901999999999e-09, -4.3002719999999993e-11, -3.898936e-09, -2.0389360000000002e-11, -2.049748e-08, -6.527374000000001e-10, -1.0336196000000001e-10, -2.697004e-11, -3.376518e-08, -6.171924e-11, -2.02069e-10, -1.200538e-09, -2.8179300000000003e-11, -6.537938e-10, -5.153115999999999e-11, -2.8508420000000003e-09, -7.534774e-07, -2.636916e-07, -1.446754e-09, -9.464432000000001e-11, -1.0602588000000001e-10, -4.217728e-11, -7.227086e-08, -3.990094e-11, -2.7389038000000002e-11, -1.90881e-07, -2.2892700000000004e-12, -4.745506e-08, -4.579318e-11, -4.5842860000000003e-11, -5.953868e-11, -3.758154e-11, -4.4363539999999995e-09, -7.143562e-11, -1.397812e-10, -7.11463e-11, -5.56664e-11, -2.6296820000000003e-08, -1.1582659999999999e-07, -2.317642e-11, -5.807276000000001e-11, -2.17813e-12, -5.7970201999999995e-11, -6.71486e-11, -8.667722000000001e-12, 3.2483739999999993e-12, -6.306573999999999e-11, -8.307524e-11, -2.4324079999999998e-12, -2.795726e-12, -2.185576e-12, -2.0225460000000002e-12, -2.122472e-12, -1.6340760000000001e-06, -2.5727129999999997e-06, -3.269066e-11, -1.83245e-12]}, {"V meas"=[3.58707, nan, nan, nan, nan, nan, nan, nan, nan, nan, nan, nan, nan, nan, nan, nan, nan, nan, nan, nan, nan, nan, nan, nan, nan, nan, nan, nan, nan, nan, nan, nan, nan, nan, nan, nan, nan, nan, nan, nan, nan, nan, nan, nan, nan, nan, nan, nan, nan, nan, nan, nan, nan, nan, nan, nan, nan, nan, nan, nan, nan, nan, nan, nan, nan, nan, nan, nan, nan, nan, nan, nan, nan, nan, nan, nan, nan, nan, nan, nan, nan, nan, nan, nan], "I meas"=[-2.049748e-08, nan, nan, nan, nan, nan, nan, nan, nan, nan, nan, nan, nan, nan, nan, nan, nan, nan, nan, nan, nan, nan, nan, nan, nan, nan, nan, nan, nan, nan, nan, nan, nan, nan, nan, nan, nan, nan, nan, nan, nan, nan, nan, nan, nan, nan, nan, nan, nan, nan, nan, nan, nan, nan, nan, nan, nan, nan, nan, nan, nan, nan, nan, nan, nan, nan, nan, nan, nan, nan, nan, nan, nan, nan, nan, nan, nan, nan, nan, nan, nan, nan, nan, nan]}]
  in  "Explore Data":bool
  out "no file":bool
  in  "Comments":string="IV test for lot 371"
  in  "FineTest save path":path=path "C:/Users/Flash/Desktop/Data/Detector test data"
  out "I fine":dbl[](array[numeric])=[-2.70504e-08, -2.32087e-08, -1.94015e-08, -1.62001e-08, -1.3396e-08, -1.06144e-08, -8.14274e-09, -5.83125e-09, -3.66964e-09, -2.05099e-09, -1.05505e-09, -6.56038e-10, -4.43558e-10, -3.24538e-10, -2.3071e-10, -1.84326e-10, -1.50747e-10, -1.31042e-10, -1.1589e-10, -1.0217e-10, -9.29752e-11, -8.22993e-11, -7.74358e-11, -6.84813e-11, -6.19634e-11, -5.51294e-11, -4.86827e-11, -4.15262e-11, -3.40749e-11, -2.82174e-11, -2.14966e-11, -1.33787e-11, -7.37435e-12, -5.50663e-12, 4.69868e-12, 1.38179e-11, 4.52471e-11, 2.99241e-10, 1.96981e-09, 2.81104e-08]
  out "V fine":dbl[](array[numeric])=[-6.0, -5.82051, -5.64103, -5.46154, -5.28205, -5.10256, -4.92308, -4.74359, -4.5641, -4.38461, -4.20513, -4.02564, -3.84615, -3.66667, -3.48718, -3.30769, -3.1282, -2.94872, -2.76923, -2.58974, -2.41026, -2.23077, -2.05128, -1.87179, -1.69231, -1.51282, -1.33333, -1.15384, -0.974358, -0.79487, -0.615383, -0.435896, -0.256409, -0.0769218, 0.102565, 0.282053, 0.46154, 0.641027, 0.820514, 1.0]
  out "Current Device":u32=1
  out "Total Device":u32=1
  out "IV fine log":cluster{dbl[], dbl[]}[](graph)=[{[-6.0, -5.82051, -5.64103, -5.46154, -5.28205, -5.10256, -4.92308, -4.74359, -4.5641, -4.38461, -4.20513, -4.02564, -3.84615, -3.66667, -3.48718, -3.30769, -3.1282, -2.94872, -2.76923, -2.58974, -2.41026, -2.23077, -2.05128, -1.87179, -1.69231, -1.51282, -1.33333, -1.15384, -0.974358, -0.79487, -0.615383, -0.435896, -0.256409, -0.0769218, 0.102565, 0.282053, 0.46154, 0.641027, 0.820514, 1.0], [2.70504e-08, 2.32087e-08, 1.94015e-08, 1.62001e-08, 1.3396e-08, 1.06144e-08, 8.14274e-09, 5.83125e-09, 3.66964e-09, 2.05099e-09, 1.05505e-09, 6.56038e-10, 4.43558e-10, 3.24538e-10, 2.3071e-10, 1.84326e-10, 1.50747e-10, 1.31042e-10, 1.1589e-10, 1.0217e-10, 9.29752e-11, 8.22993e-11, 7.74358e-11, 6.84813e-11, 6.19634e-11, 5.51294e-11, 4.86827e-11, 4.15262e-11, 3.40749e-11, 2.82174e-11, 2.14966e-11, 1.33787e-11, 7.37435e-12, 5.50663e-12, 4.69868e-12, 1.38179e-11, 4.52471e-11, 2.99241e-10, 1.96981e-09, 2.81104e-08]}]
  out "Progress 2":u8(slide)=100 scale=0.0..100.0
  in  "StartFine":bool
  out "IV fine linear":cluster{dbl[], dbl[]}[](graph)=[{[-6.0, -5.82051, -5.64103, -5.46154, -5.28205, -5.10256, -4.92308, -4.74359, -4.5641, -4.38461, -4.20513, -4.02564, -3.84615, -3.66667, -3.48718, -3.30769, -3.1282, -2.94872, -2.76923, -2.58974, -2.41026, -2.23077, -2.05128, -1.87179, -1.69231, -1.51282, -1.33333, -1.15384, -0.974358, -0.79487, -0.615383, -0.435896, -0.256409, -0.0769218, 0.102565, 0.282053, 0.46154, 0.641027, 0.820514, 1.0], [-2.70504e-08, -2.32087e-08, -1.94015e-08, -1.62001e-08, -1.3396e-08, -1.06144e-08, -8.14274e-09, -5.83125e-09, -3.66964e-09, -2.05099e-09, -1.05505e-09, -6.56038e-10, -4.43558e-10, -3.24538e-10, -2.3071e-10, -1.84326e-10, -1.50747e-10, -1.31042e-10, -1.1589e-10, -1.0217e-10, -9.29752e-11, -8.22993e-11, -7.74358e-11, -6.84813e-11, -6.19634e-11, -5.51294e-11, -4.86827e-11, -4.15262e-11, -3.40749e-11, -2.82174e-11, -2.14966e-11, -1.33787e-11, -7.37435e-12, -5.50663e-12, 4.69868e-12, 1.38179e-11, 4.52471e-11, 2.99241e-10, 1.96981e-09, 2.81104e-08]}]
  in  "Mask File Fine":path=path "C:/Users/Flash/Desktop/Data/Detector test data/SJC_ENG_371_4-GaAs/A-3719-2-A/Raw Data/PH001_Detector Aligner mask map file _ full top_open top 10_open top 5 diodes_Open_Diode_1000_A-3719-2-A_091318_080341.5AM.csv"
  out "Y":dbl
  out "X":dbl
  in  "move prober 2":bool
  in  "load file for temp series":bool
  in  "Mask File Temperature":path=path "C:/Users/Flash/Desktop/Data/Detector test data/PH001 Detector Aligner mask map file _ full top_open top 10_open top 5 diodes_Open_Diode_5_300_A-3605-1-A_052518_113739.0AM.csv"
  out "IV temp linear":cluster{dbl[], dbl[]}[](graph)
  in  "Start temp":bool
  out "IV temp log":cluster{dbl[], dbl[]}[](graph)
  out "V fine temp":dbl[](array[numeric])=[-1.5, -1.45128, -1.40256, -1.35385, -1.30513, -1.25641, -1.20769, -1.15897, -1.11026, -1.06154, -1.01282, -0.964102, -0.915384, -0.866666, -0.817948, -0.76923, -0.720512, -0.671794, -0.623076, -0.574358, -0.52564, -0.476923, -0.428205, -0.379487, -0.330769, -0.282051, -0.233333, -0.184615, -0.135897, -0.087179, -0.038461, 0.0102569, 0.0589749, 0.107693, 0.156411, 0.205129, 0.253847, 0.302565, 0.351283, 0.400001]
  out "I fine temp":dbl[](array[numeric])=[-1.28772e-07, -1.20805e-07, -1.15592e-07, -1.10987e-07, -1.06412e-07, -1.02022e-07, -4.62038e-08, -9.34188e-08, -8.97462e-08, -8.60003e-08, -8.23237e-08, -7.87101e-08, -7.52945e-08, -7.18306e-08, -6.85145e-08, -6.5287e-08, -6.2088e-08, -5.90038e-08, -5.59938e-08, -5.29941e-08, -5.00661e-08, -4.71812e-08, -4.43421e-08, -4.15389e-08, -3.87298e-08, -3.5945e-08, -3.31511e-08, -3.027e-08, -2.71168e-08, -2.30654e-08, -1.54139e-08, 7.82768e-09, 2.30625e-07, 5.07951e-07, 2.21662e-06, 9.15235e-06, 3.37902e-05, 9.47719e-05, 0.000202989, 0.000357986]
  in  "Temperature Series save path":path=path "C:/Users/Flash/Desktop/Data/Detector test data"
  in  "Comments Temp":string
  in  "Single Device Temperature List":i32(listbox)=-1
  in  "Desired Temperature":dbl=25.0
  in  "Add to Temp":bool
  in  "Remove from Temp":bool
  in  "Clear temp list":bool
  in  "Desired Device":u16(ring)=50 items=["0", "1", "2", "3", "4", "5", "6", "7", "8", "9"]
  in  "Channel Keysight":dbl
  in  "Keysight SMU":refnum<visa-resource-name>="GPIB0::23::INSTR"
  in  "update temp":bool
  out "Current Temp":string="0\r"
  in  "Temp Setpoint":string="25"
  in  "Temptronics VISA":refnum<visa-resource-name>="GPIB0::9::INSTR"
  in  "Prober GPIB":string="0:1"
  in  "Keithley SMU":refnum<visa-resource-name>="GPIB0::26::INSTR"
  in  "Channel":enum32{"Channel A", "Channel B"}(ring)
  out "Calibration":cluster{"Y":dbl[], "Y":dbl[]}[](graph)=[{"Y"=[0.1, 0.2, 0.3, 0.4, 0.5, 0.6, 0.7, 0.8, 0.9, 1.0, 1.1, 1.2, 1.3, 1.4, 1.5, 1.6, 1.7, 1.8, 1.9, 2.0, 2.1, 2.2, 2.3, 2.4, 2.5, 2.6, 2.7, 2.8, 2.9, 3.0, 3.1, 3.2, 3.3, 3.4, 3.5, 3.6, 3.7, 3.8, 3.9, 4.0, 4.1, 4.2, 4.3, 4.4, 4.5, 4.6, 4.7, 4.8, 4.9, 5.0, 5.1, 5.2, 5.3, 5.4, 5.5, 5.6, 5.7, 5.8, 5.9, 6.0, 6.1, 6.2, 6.3, 6.4, 6.5, 6.6, 6.7, 6.8, 6.9, 7.0, 7.1, 7.2, 7.3, 7.4, 7.5, 7.6, 7.7, 7.8, 7.9, 8.0, 8.1, 8.2, 8.3, 8.4, 8.5, 8.6, 8.7, 8.8, 8.9, 9.0, 9.1, 9.2, 9.3, 9.4, 9.5, 9.6, 9.7, 9.8, 9.9, 10.0, 10.1, 10.2, 10.3, 10.4, 10.5, 10.6, 10.7, 10.8, 10.9, 11.0, 11.1, 11.2, 11.3, 11.4, 11.5, 11.6, 11.7, 11.8, 11.9, 12.0, 12.1, 12.2, 12.3, 12.4, 12.5, 12.6, 12.7, 12.8, 12.9, 13.0, 13.1, 13.2, 13.3, 13.4, 13.5, 13.6, 13.7, 13.8, 13.9, 14.0, 14.1, 14.2, 14.3, 14.4, 14.5, 14.6, 14.7, 14.8, 14.9, 15.0, 15.1, 15.2, 15.3, 15.4, 15.5, 15.6, 15.7, 15.8, 15.9, 16.0, 16.1, 16.2, 16.3, 16.4, 16.5, 16.6, 16.7, 16.8, 16.9, 17.0, 17.1, 17.2, 17.3, 17.4, 17.5, 17.6, 17.7, 17.8, 17.9, 18.0, 18.1, 18.2, 18.3, 18.4, 18.5, 18.6, 18.7, 18.8, 18.9, 19.0, 19.1, 19.2, 19.3, 19.4, 19.5, 19.6, 19.7, 19.8, 19.9, 20.0, 20.1, 20.2, 20.3, 20.4, 20.5, 20.6, 20.7, 20.8, 20.9, 21.0, 21.1, 21.2, 21.3, 21.4, 21.5, 21.6, 21.7, 21.8, 21.9, 22.0, 22.1, 22.2, 22.3, 22.4, 22.5, 22.6, 22.7, 22.8, 22.9, 23.0, 23.1, 23.2, 23.3, 23.4, 23.5, 23.6, 23.7, 23.8, 23.9, 24.0, 24.1, 24.2, 24.3, 24.4, 24.5, 24.6, 24.7, 24.8, 24.9, 25.0, 25.1, 25.2, 25.3, 25.4, 25.5, 25.6, 25.7, 25.8, 25.9, 26.0, 26.1, 26.2, 26.3, 26.4, 26.5, 26.6, 26.7, 26.8, 26.9, 27.0, 27.1, 27.2, 27.3, 27.4, 27.5, 27.6, 27.7, 27.8, 27.9, 28.0, 28.1, 28.2, 28.3, 28.4, 28.5, 28.6, 28.7, 28.8, 28.9, 29.0, 29.1, 29.2, 29.3, 29.4, 29.5, 29.6, 29.7, 29.8, 29.9, 30.0, 30.1, 30.2, 30.3, 30.4, 30.5, 30.6, 30.7, 30.8, 30.9, 31.0, 31.1, 31.2, 31.3, 31.4, 31.5, 31.6, 31.7, 31.8, 31.9, 32.0, 32.1, 32.2, 32.3, 32.4, 32.5, 32.6, 32.7, 32.8, 32.9, 33.0, 33.1, 33.2, 33.3, 33.4, 33.5, 33.6, 33.7, 33.8, 33.9, 34.0, 34.1, 34.2, 34.3, 34.4, 34.5, 34.6, 34.7, 34.8, 34.9, 35.0, 35.1, 35.2, 35.3, 35.4, 35.5, 35.6, 35.7, 35.8, 35.9, 36.0, 36.1, 36.2, 36.3, 36.4, 36.5, 36.6, 36.7, 36.8, 36.9, 37.0, 37.1, 37.2, 37.3, 37.4, 37.5, 37.6, 37.7, 37.8, 37.9, 38.0, 38.1, 38.2, 38.3, 38.4, 38.5, 38.6, 38.7, 38.8, 38.9, 39.0, 39.1, 39.2, 39.3, 39.4, 39.5, 39.6, 39.7, 39.8, 39.9, 40.0], "Y"=[0.0, 0.0, 0.0, 0.0, 0.0, 0.0, 0.0, 0.0, 0.0, 0.0, 0.0, 0.0, 0.0, 0.0, 0.0, 0.0, 0.0, 0.001, 0.001, 0.001, 0.001, 0.001, 0.001, 0.001, 0.001, 0.001, 0.001, 0.001, 0.001, 0.001, 0.001, 0.001, 0.001, 0.002, 0.002, 0.002, 0.002, 0.002, 0.002, 0.002, 0.002, 0.002, 0.002, 0.003, 0.003, 0.003, 0.003, 0.003, 0.003, 0.004, 0.004, 0.004, 0.004, 0.004, 0.005, 0.005, 0.005, 0.005, 0.006, 0.006, 0.006, 0.007, 0.007, 0.007, 0.008, 0.008, 0.008, 0.009, 0.009, 0.01, 0.01, 0.011, 0.011, 0.012, 0.012, 0.013, 0.013, 0.014, 0.015, 0.016, 0.017, 0.019, 0.023, 0.037, 0.058, 0.075, 0.091, 0.109, 0.127, 0.149, 0.168, 0.185, 0.202, 0.22, 0.243, 0.261, 0.279, 0.297, 0.314, 0.332, 0.354, 0.372, 0.391, 0.409, 0.427, 0.449, 0.466, 0.485, 0.503, 0.522, 0.544, 0.561, 0.579, 0.597, 0.615, 0.633, 0.658, 0.674, 0.692, 0.71, 0.728, 0.751, 0.768, 0.787, 0.807, 0.824, 0.845, 0.862, 0.88, 0.899, 0.918, 0.933, 0.957, 0.976, 0.993, 1.012, 1.029, 1.051, 1.07, 1.089, 1.103, 1.124, 1.145, 1.165, 1.183, 1.202, 1.217, 1.239, 1.256, 1.276, 1.294, 1.315, 1.333, 1.356, 1.376, 1.389, 1.405, 1.43, 1.45, 1.467, 1.485, 1.508, 1.524, 1.546, 1.56, 1.579, 1.598, 1.614, 1.631, 1.656, 1.679, 1.695, 1.715, 1.731, 1.75, 1.769, 1.791, 1.801, 1.824, 1.84, 1.865, 1.881, 1.897, 1.912, 1.93, 1.953, 1.974, 1.993, 2.006, 2.028, 2.052, 2.073, 2.087, 2.105, 2.125, 2.146, 2.164, 2.186, 2.203, 2.213, 2.243, 2.258, 2.276, 2.296, 2.311, 2.328, 2.35, 2.366, 2.389, 2.412, 2.426, 2.45, 2.459, 2.476, 2.502, 2.522, 2.53, 2.561, 2.571, 2.593, 2.609, 2.626, 2.652, 2.666, 2.691, 2.704, 2.729, 2.74, 2.764, 2.782, 2.807, 2.817, 2.837, 2.854, 2.869, 2.886, 2.908, 2.937, 2.947, 2.979, 2.988, 3.002, 3.033, 3.043, 3.064, 3.075, 3.1, 3.111, 3.145, 3.156, 3.181, 3.196, 3.212, 3.232, 3.246, 3.273, 3.289, 3.299, 3.327, 3.35, 3.371, 3.374, 3.4, 3.418, 3.45, 3.462, 3.483, 3.499, 3.516, 3.531, 3.55, 3.564, 3.592, 3.608, 3.629, 3.662, 3.674, 3.693, 3.717, 3.727, 3.752, 3.772, 3.78, 3.804, 3.82, 3.838, 3.87, 3.871, 3.889, 3.91, 3.938, 3.945, 3.97, 3.981, 4.008, 4.023, 4.048, 4.058, 4.076, 4.113, 4.131, 4.144, 4.172, 4.183, 4.199, 4.227, 4.24, 4.258, 4.285, 4.301, 4.32, 4.316, 4.347, 4.38, 4.395, 4.4, 4.426, 4.449, 4.458, 4.471, 4.488, 4.507, 4.529, 4.555, 4.571, 4.584, 4.624, 4.629, 4.654, 4.684, 4.686, 4.715, 4.731, 4.733, 4.756, 4.781, 4.791, 4.815, 4.82, 4.847, 4.864, 4.89, 4.907, 4.923, 4.935, 4.976, 4.983, 5.002, 5.022, 5.05, 5.065, 5.074, 5.082, 5.1, 5.123, 5.154, 5.154, 5.187, 5.22, 5.239, 5.253, 5.261, 5.278, 5.285, 5.316, 5.333, 5.363, 5.375, 5.388, 5.405, 5.426, 5.432, 5.455, 5.493, 5.508, 5.516, 5.539, 5.54, 5.569, 5.584, 5.594, 5.623, 5.639, 5.678, 5.667, 5.689, 5.724, 5.742, 5.738, 5.771, 5.806, 5.814, 5.826, 5.847, 5.852, 5.877, 5.906, 5.912, 5.934, 5.958]}]
  out "Laser Error":errorcluster caption="error out" {"code" format="%.0x"}
  in  "Load Calibration File":path=path "C:/Users/Flash/Desktop/Laser Calibration Files/Calib7_23_18.csv"
  in  "TL4000 In":refnum<visa-resource-name>="USB0::0x1313::0x804F::M00445403::INSTR" caption="resource name"
  in  "Enable Laser":bool=TRUE
  out "Raw Test Filename":path=path "C:/Users/Flash/Desktop/Data/Detector test data/SJC_ENG_371_4-GaAs/A-3719-2-A/Raw Data/A-3719-2-A_Open_Diode_1000_20180913075240.csv"
  out "new raw data save path":path=path "C:/Users/Flash/Desktop/Data/Detector test data/SJC_ENG_371_4-GaAs/A-3719-2-A/Raw Data"
  out "Error Out":errorcluster
  in  "Wait after load":u32
  in  "Keysight":bool
  out "Temp Controller Found":bool
  out "Keithley SMU Found":bool
  out "Keysight SMU Found":bool=TRUE
  out "Thorlabs Laser Found":bool=TRUE
  out "EG Prober Found":bool=TRUE
  out "Test Type":string="Auto Test"
  in  "Update viewer":bool
  in  "Logview":i32(listbox)=-1
  in  "Add Comments":string
  in  "Save Comment":bool
  out "Last Measurement":T16={"result string"="9_13_2018", "time string"="11:39 AM", "Wafer Name"="A-3719-2-A", "Operator"="sswifter", "Test description"="IV test for lot 371", "Test Type"="Auto Test"}
  in  "Measurement Log Path":path=path "C:/Users/Flash/Desktop/Data/Detector test data/MeasurementLog.csv"
  # "0 is for dark IV!"
  # "Sweep Settings"
  # "Forward Voltage"
  # "Dark/Light Current"
  # "Check settings before click start!"
  # "Make sure current x and y are same as prober before click Start!"
  # "TEC Control"
  # "TL4000 Settings"
  # "Keithley"
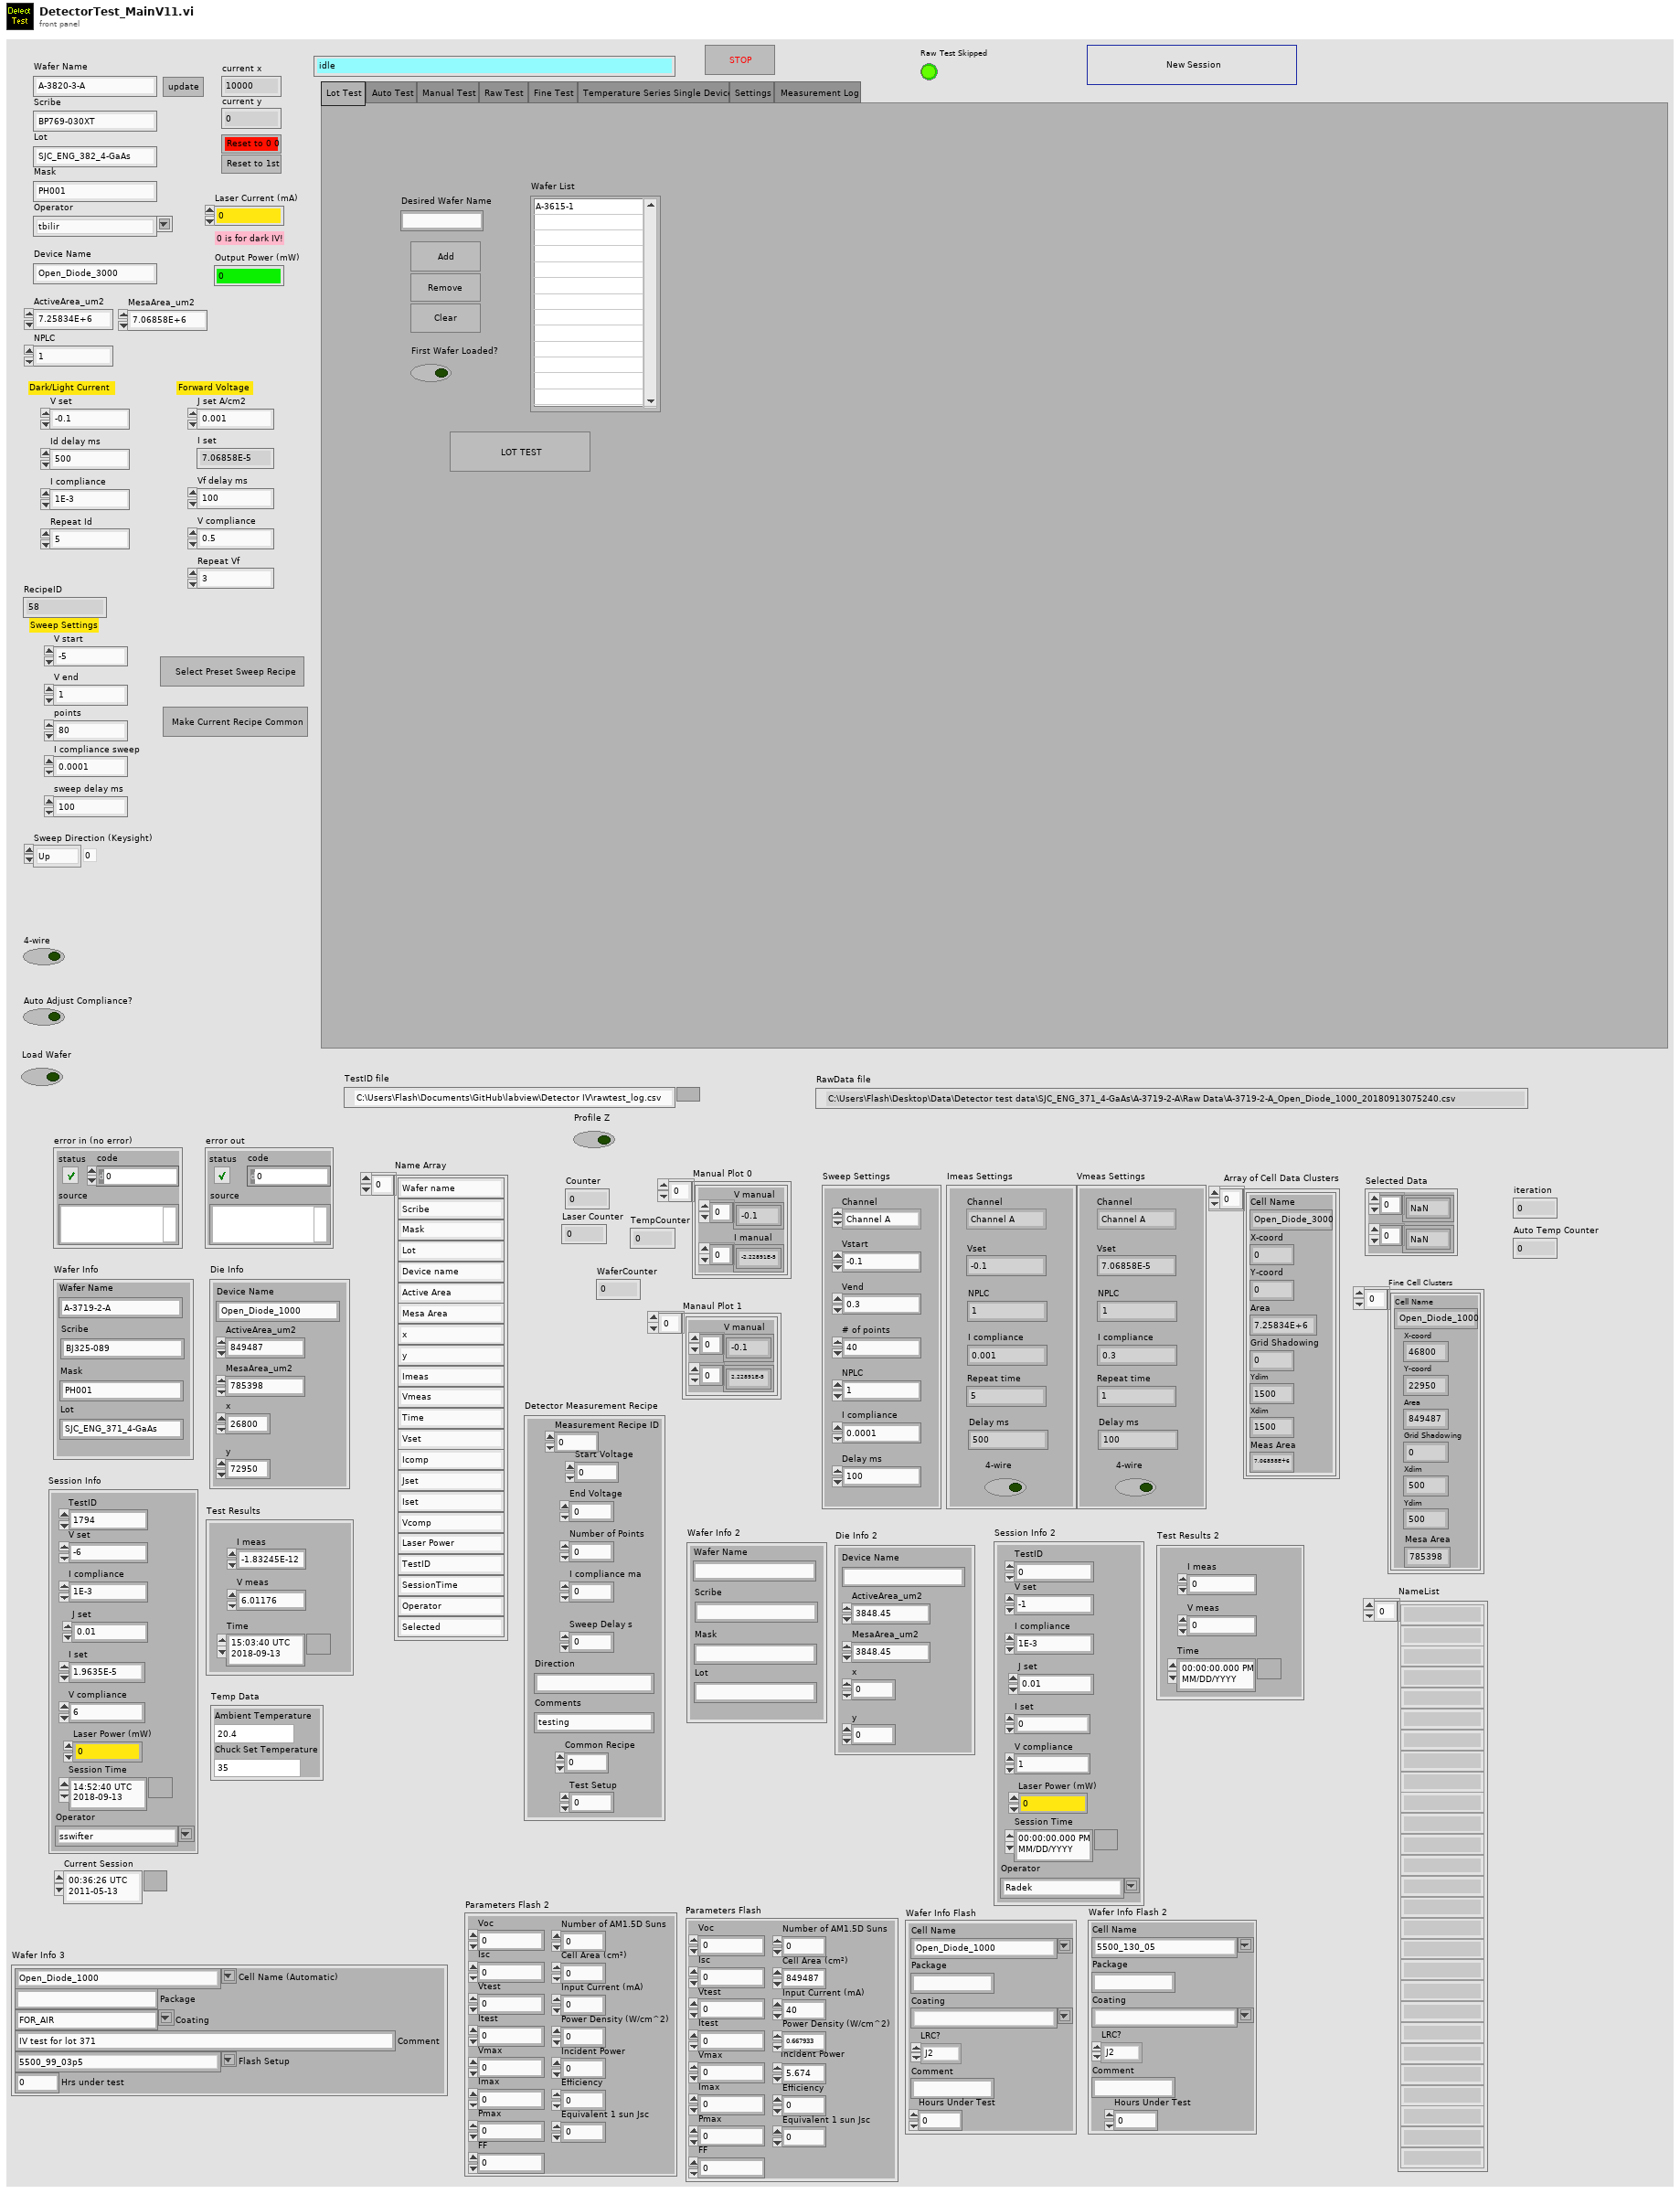
[diagram p1: front panel]
types:
  T1 = cluster{"Start Voltage":dbl, "End Voltage":dbl, "Number of Points":dbl, "I compliance ma":dbl, "Sweep Delay s":dbl, "Direction":string, "Comments":string, "Common Recipe":dbl, "Test Setup":dbl, "Measurement Recipe ID":dbl}
  T2 = cluster{"Ambient Temperature":dbl, "Chuck Set Temperature":dbl}
  T3 = cluster{"Cell Name (Automatic)":string, "Package":string, "Coating":string, "Comment":string, "Flash Setup":string, "Hrs under test":dbl}
  T4 = cluster{"Cell Name":string, "Package":string, "Coating":string, "LRC?":enum16{"J1", "J2", "LRC"}, "Comment":string, "Hours Under Test":dbl}
  T5 = cluster{"Voc":dbl, "Isc":dbl, "FF":dbl, "Vtest":dbl, "Imax":dbl, "Vmax":dbl, "Pmax":dbl, "Itest":dbl, "Efficiency":dbl, "Incident Power":dbl, "Power Density (W/cm^2)":dbl, "Cell Area (cm²)":dbl, "Number of AM1.5D Suns":dbl, "Input Current (mA)":dbl, "Equivalent 1 sun Jsc":dbl}
  T6 = cluster{"Cell Name":string, "X-coord":dbl, "Y-coord":dbl, "Area":dbl, "Grid Shadowing":dbl, "Xdim":dbl, "Ydim":dbl, "Mesa Area":dbl}[]
  T7 = cluster{"I meas":dbl, "V meas":dbl, "Time":timestamp}
  T8 = cluster{"V set":dbl, "I compliance":dbl, "J set":dbl, "I set":dbl, "V compliance":dbl, "Laser Power (mW)":dbl, "TestID":u32, "Session Time":timestamp, "Operator":string}
  T9 = cluster{"Device Name":string, "ActiveArea_um2":dbl, "MesaArea_um2":dbl, "x":dbl, "y":dbl}
  T10 = cluster{"Wafer Name":string, "Scribe":string, "Mask":string, "Lot":string}
  T11 = cluster{"Channel":enum32{"Channel A", "Channel B"}, "Vstart":dbl, "Vend":dbl, "# of points":u16, "NPLC":dbl, "I compliance":dbl, "Delay ms":dbl}
  T12 = typedef "SMU Settings.ctl" = cluster{"Channel":enum32{"Channel A", "Channel B"}, "Vset":dbl, "NPLC":dbl, "I compliance":dbl, "Repeat time":u16, "Delay ms":dbl, "4-wire":bool}
  T13 = cluster{"Cell Name":string, "X-coord":dbl, "Y-coord":dbl, "Area":dbl, "Grid Shadowing":dbl, "Ydim":dbl, "Xdim":dbl, "Meas Area":dbl}[]
  T14 = enum32{"Lot Test", "Auto Test", "Manual Test", "Raw Test", "Fine Test", "Temperature Series Single Device", "Settings", "Measurement Log"}
  T15 = cluster{"X Values":dbl[], "Histogram: h(x)":i32[]}
  T16 = cluster{"result string":string, "time string":string, "Wafer Name":string, "Operator":string, "Test description":string, "Test Type":string}
  T17 = enum32{"Lot Test", "Auto Test", "Manual Test", "Raw Test", "Fine Test", "Temperature Series Single Device", "Settings"}
  T18 = cluster{"Cell Name":string, "X-coord":dbl, "Y-coord":dbl, "Area":dbl, "Grid Shadowing":dbl, "Ydim":dbl, "Xdim":dbl, "Meas Area":dbl}
  T19 = cluster{"Varray manual":dbl[], "Iarray manual":dbl[]}[]
  T20 = cluster{"Start Voltage":dbl, "End Voltage":dbl, "# Data Points":dbl, "I compliance":dbl, "Sweep Delay":dbl, "Direction":string, "Comments":string, "Recipe ID":dbl, "Common Recipe":dbl, "Setup ID":dbl}
  T21 = cluster{"Start Voltage":dbl, "End Voltage":dbl, "Number of Points":dbl, "I compliance ma":dbl, "Sweep Delay s":dbl, "Direction":string}
  T22 = cluster{"Start Voltage":dbl, "End Voltage":dbl, "Number of Points":dbl, "I compliance ma":dbl, "Sweep Delay s":dbl, "Direction":string, "Comments":string, "Common Recipe":dbl, "Test Setup":dbl}
  T23 = cluster{"WaferName":string, "Scribe":string, "Structure":string, "Lot":string, "Mask":string}
  T24 = cluster{"V set":dbl, "I compliance":dbl, "J set":dbl, "I set":dbl, "V compliance":dbl, "Laser Power (mW)":dbl, "TestID":u32, "Operator":string}
  T25 = cluster{"Device Name":string, "ActiveArea_um2":dbl, "MesaArea_um2":dbl}
  T26 = cluster{"Cell Name":string, "X-coord":dbl, "Y-coord":dbl, "Area":dbl, "Grid Shadowing":dbl, "Xdim":dbl, "Ydim":dbl, "Mesa Area":dbl}
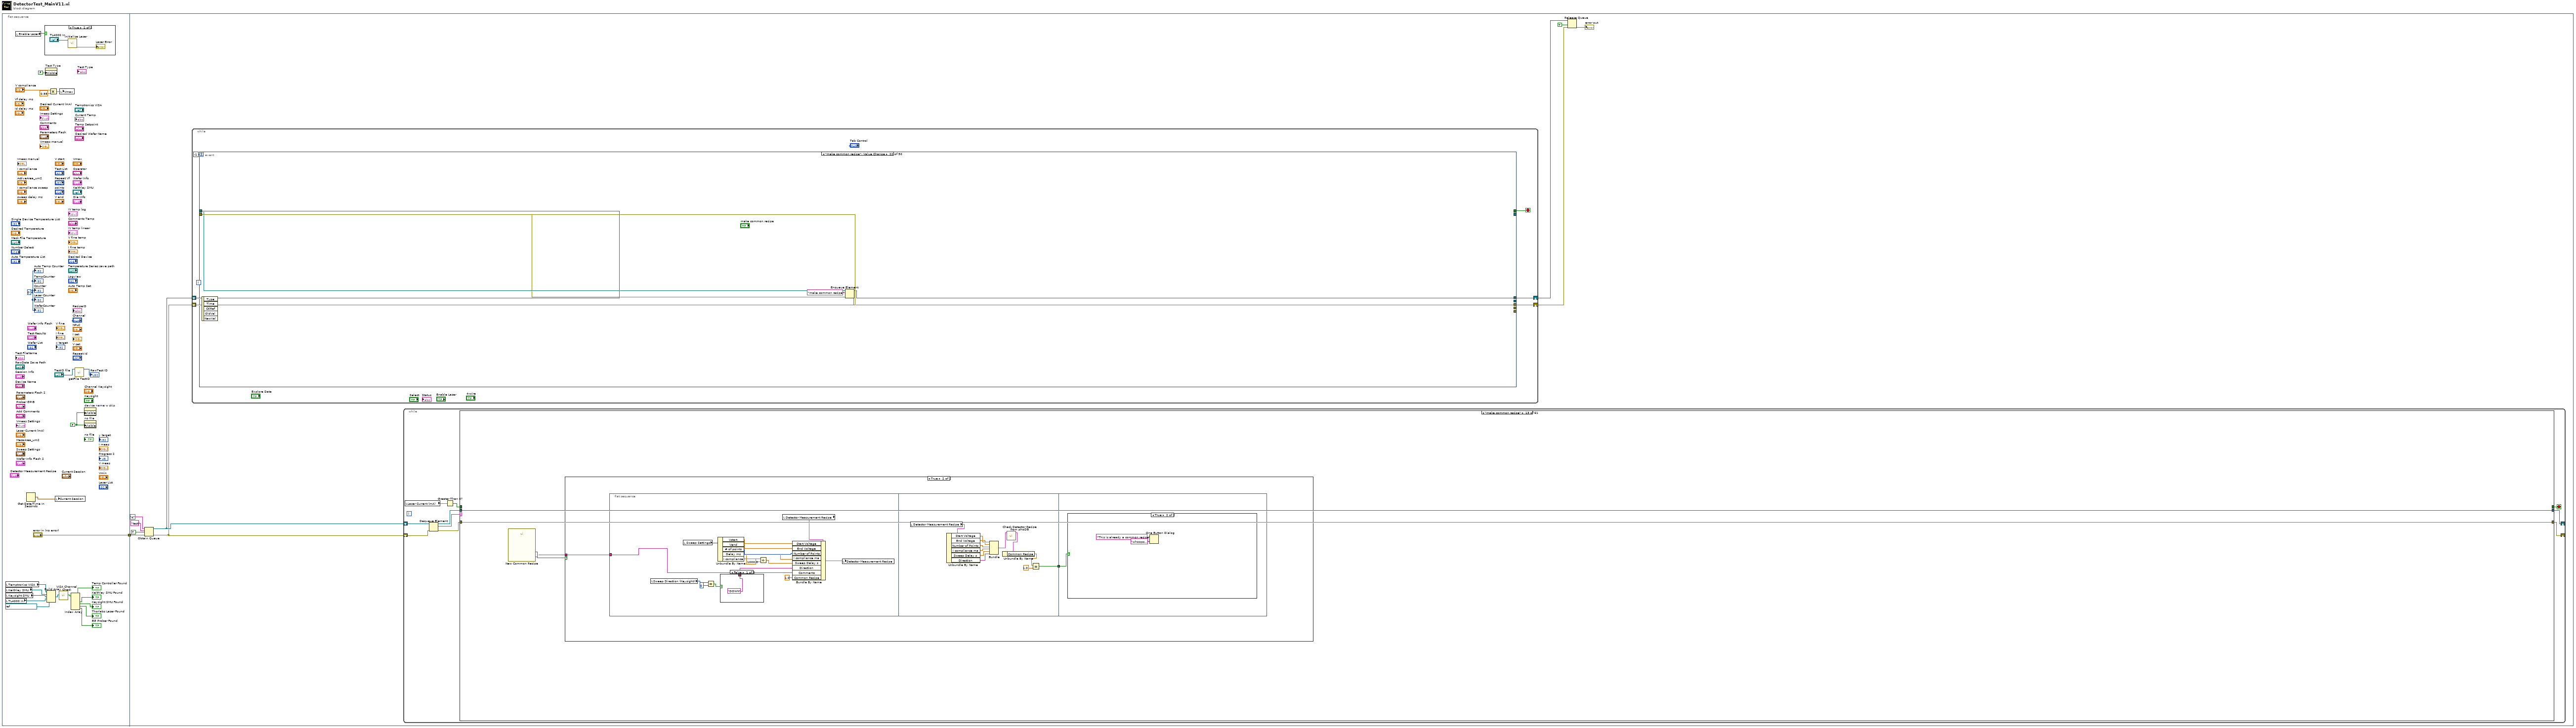
[diagram p0: block diagram]
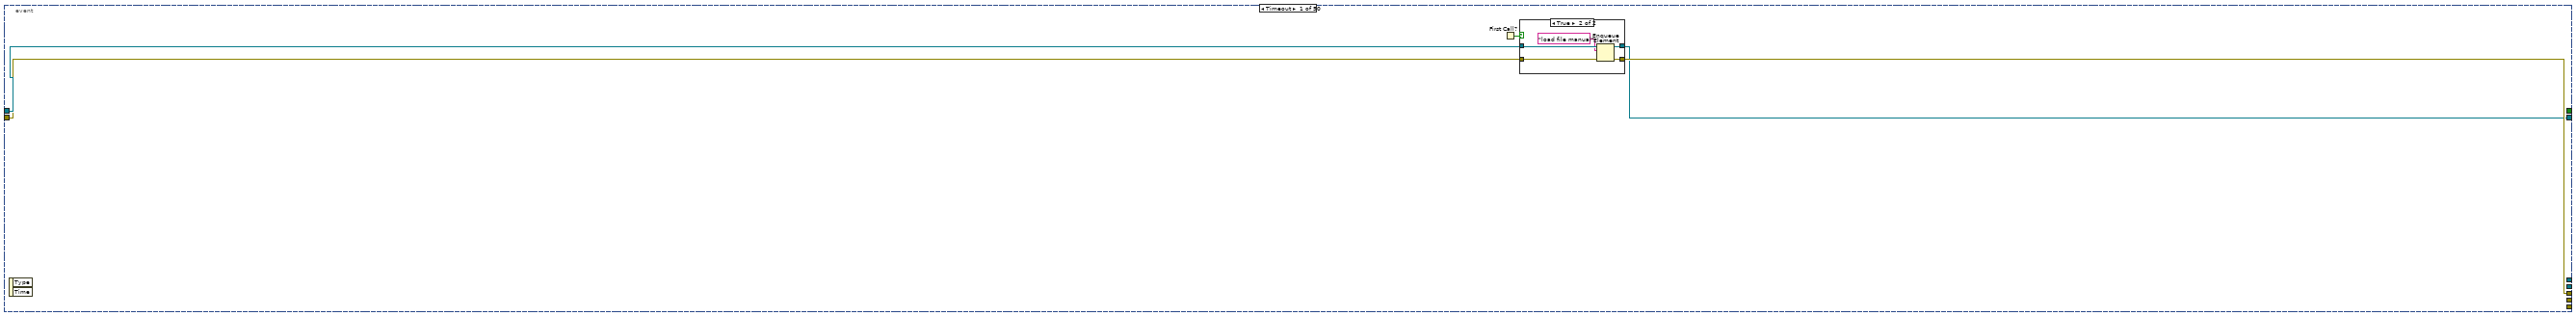
[diagram p3: hidden frame]
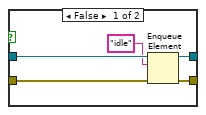
[diagram p4: hidden frame]
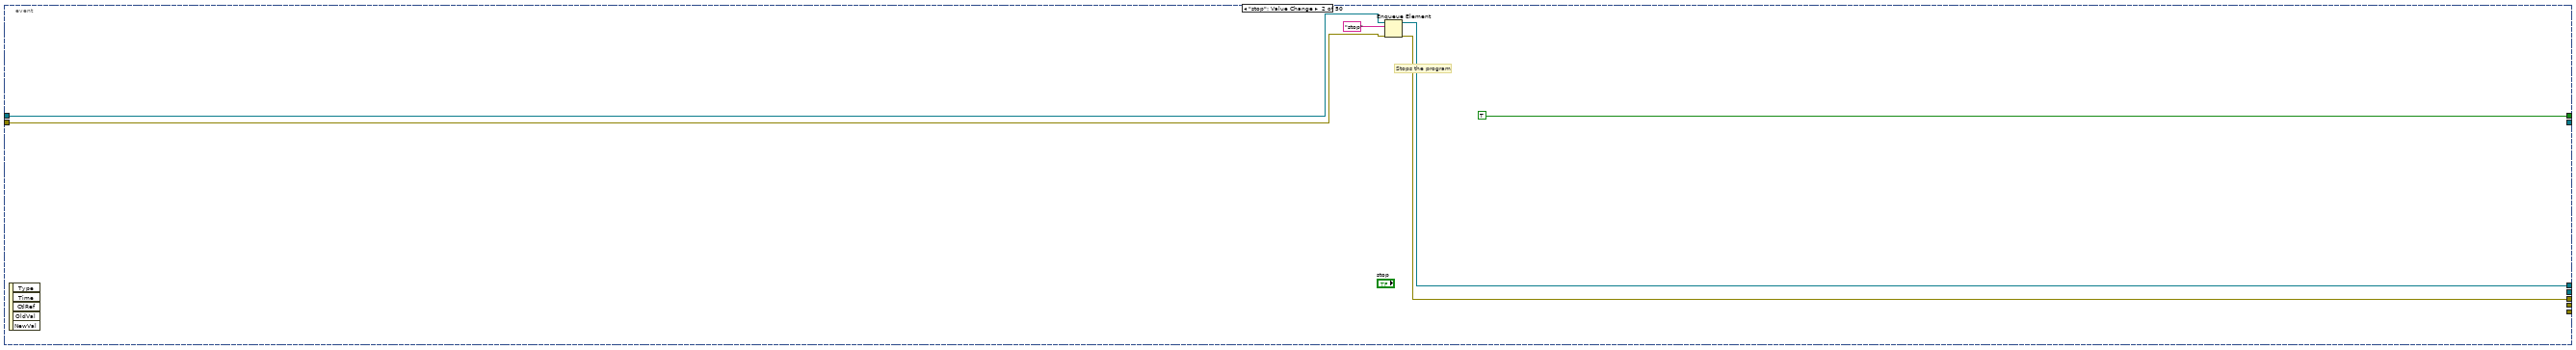
[diagram p5: hidden frame]
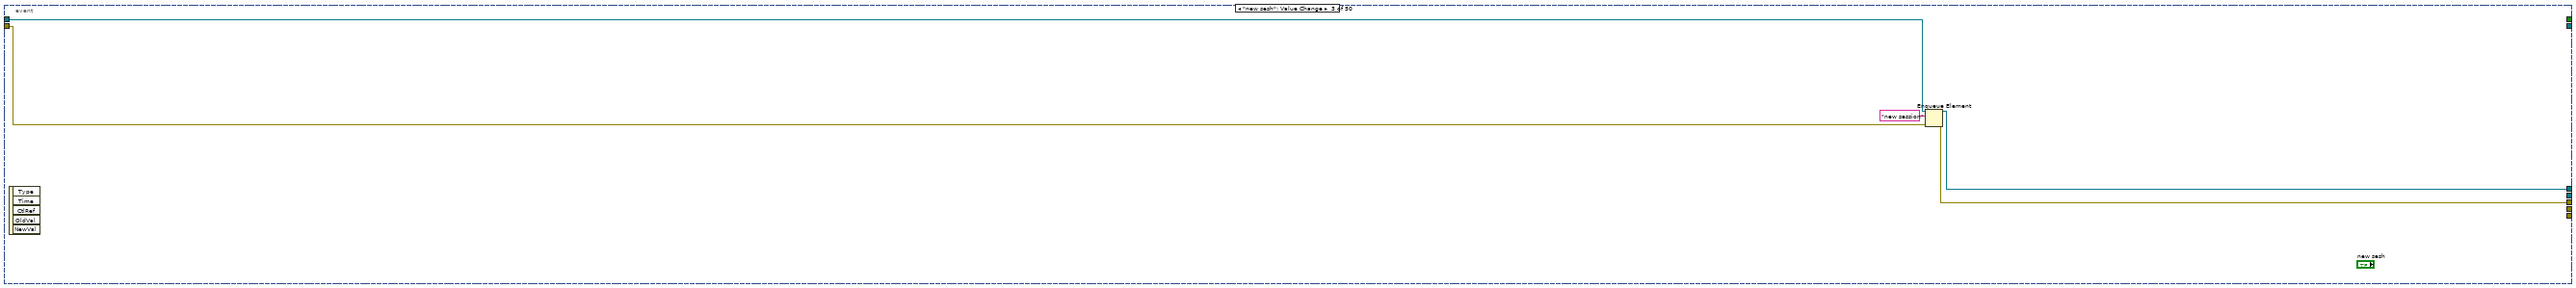
[diagram p6: hidden frame]
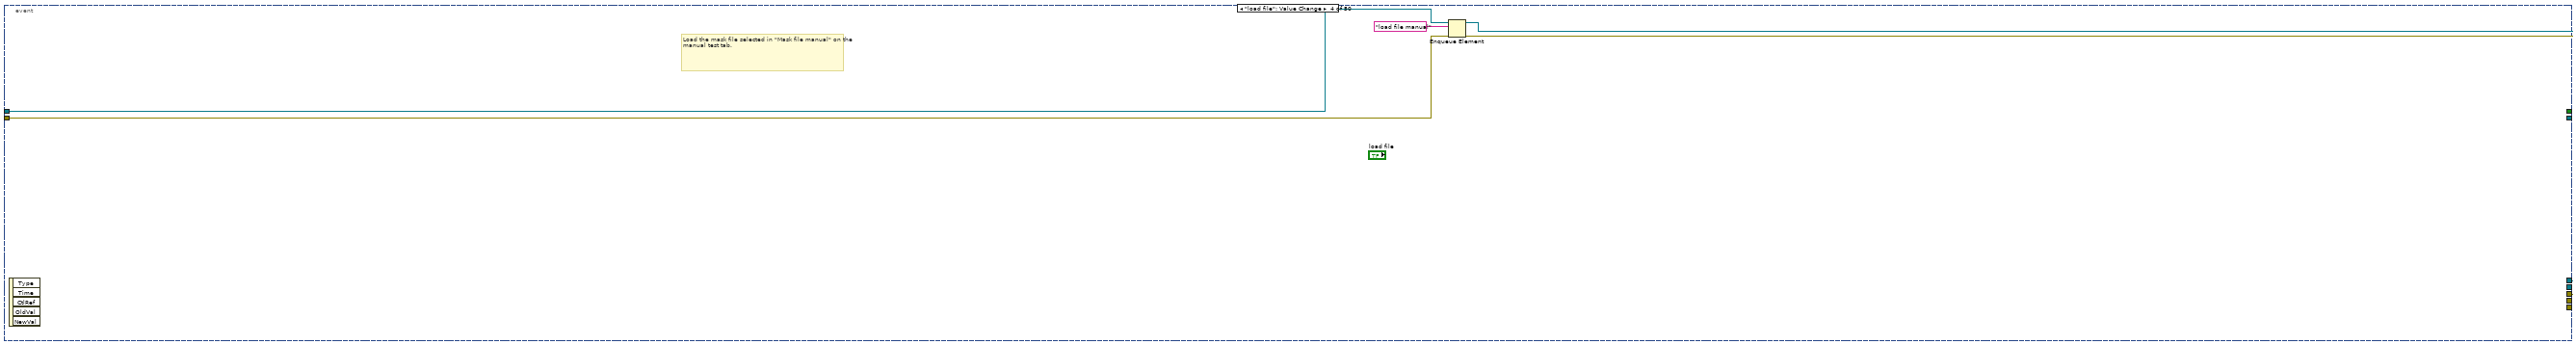
[diagram p7: hidden frame]
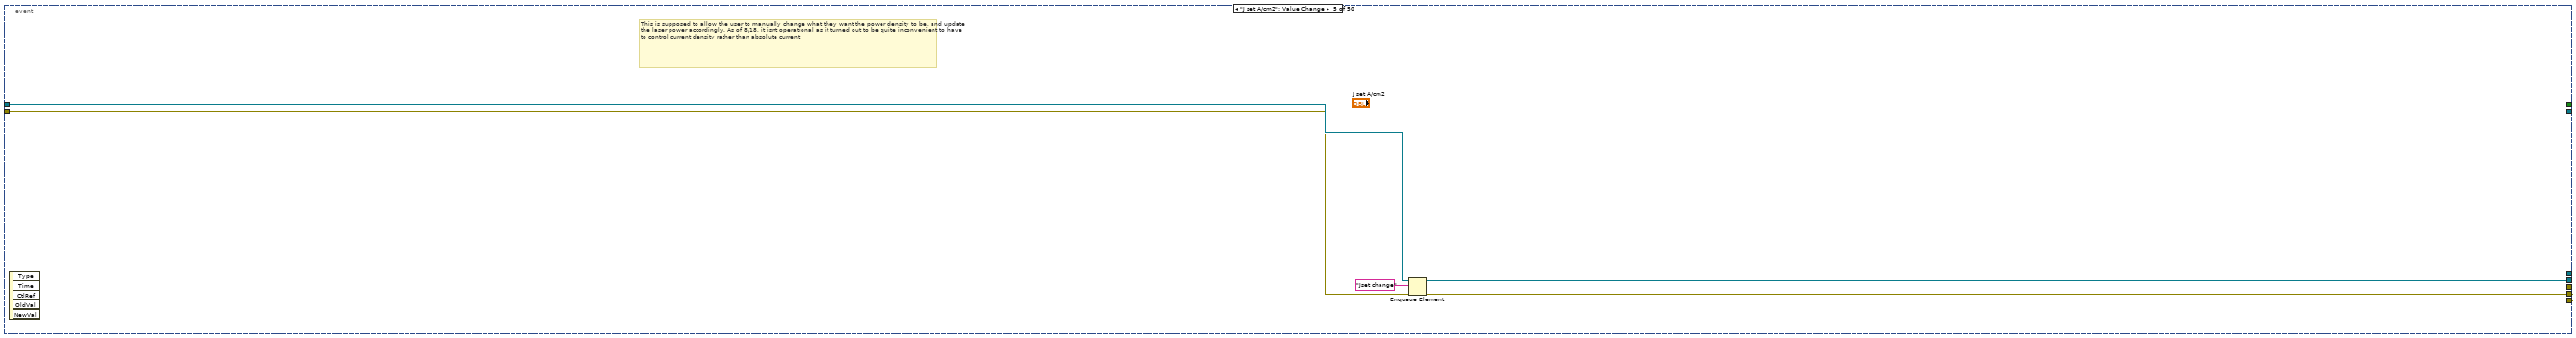
[diagram p8: hidden frame]
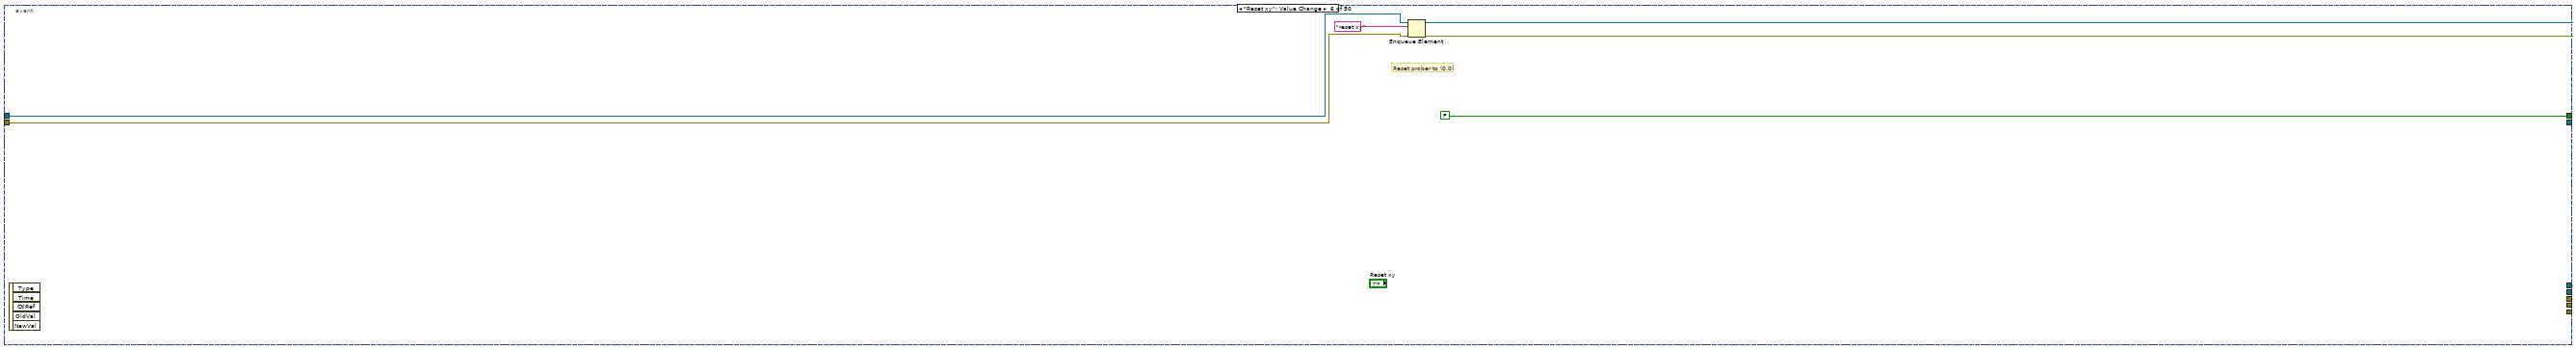
[diagram p9: hidden frame]
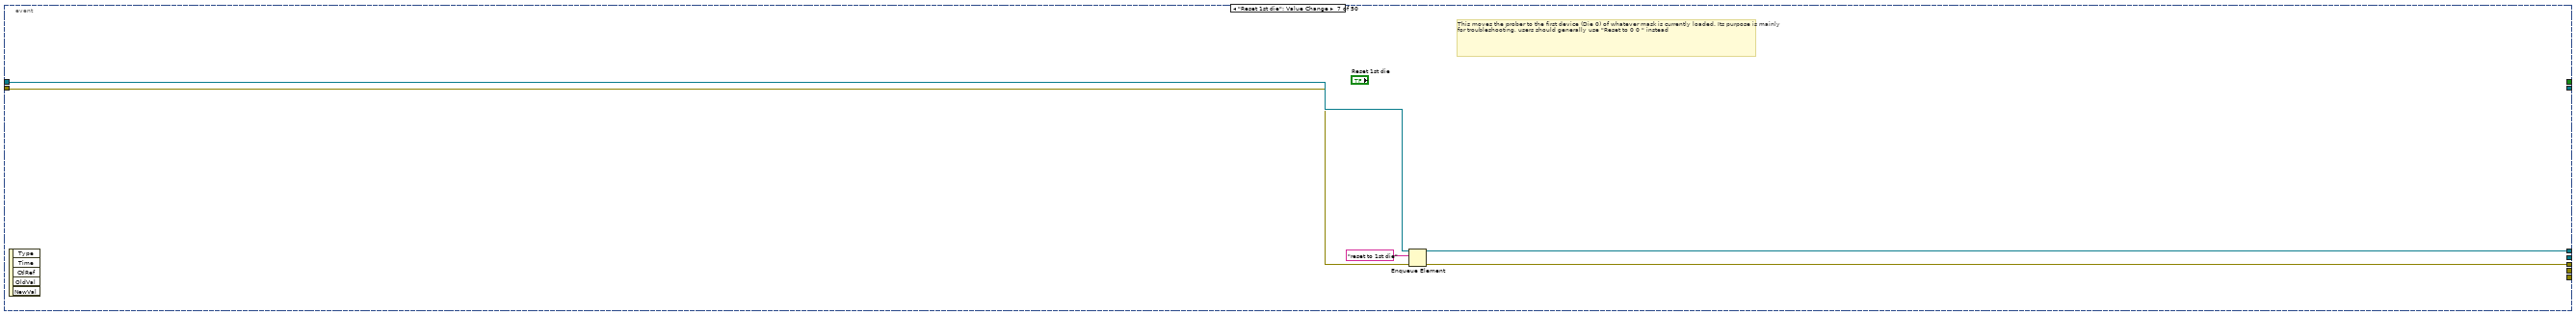
[diagram p10: hidden frame]
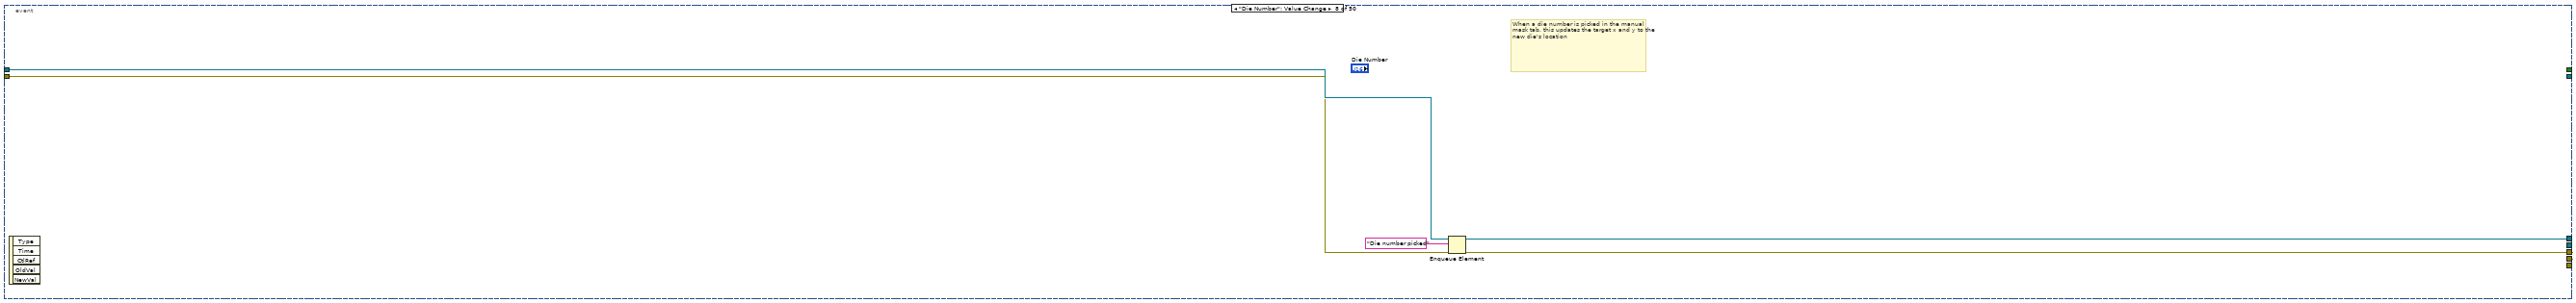
[diagram p11: hidden frame]
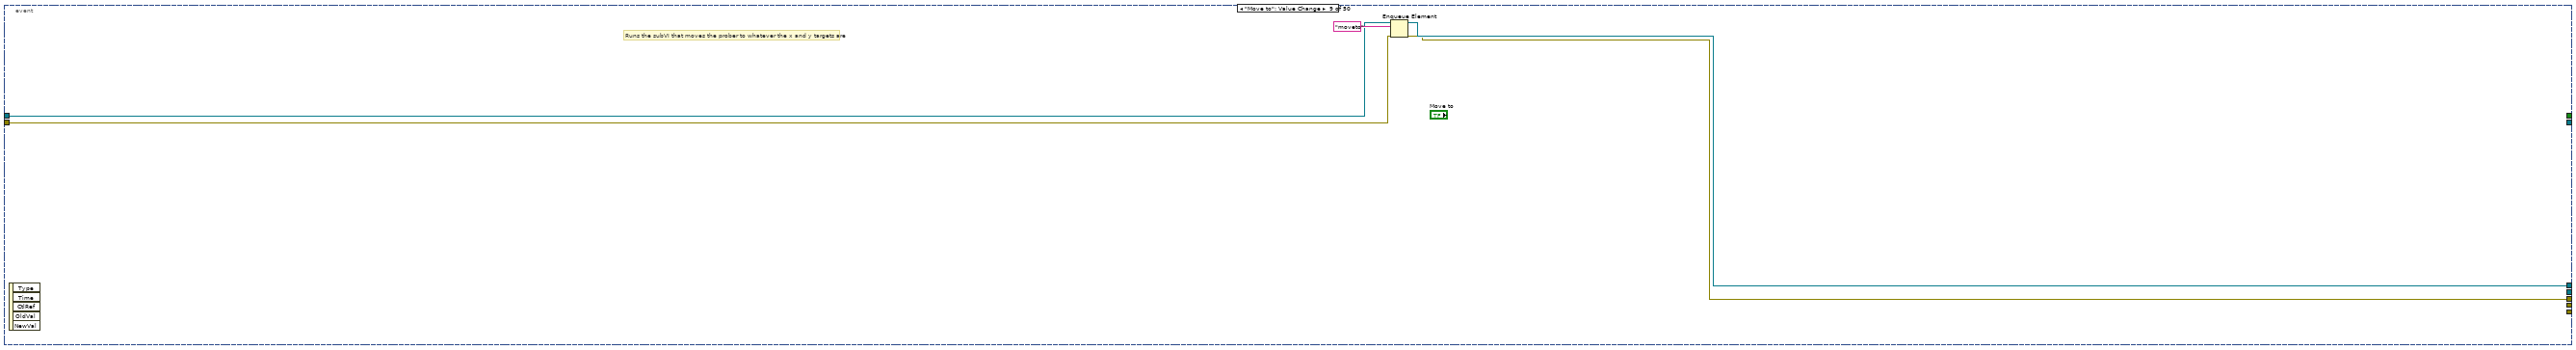
[diagram p12: hidden frame]
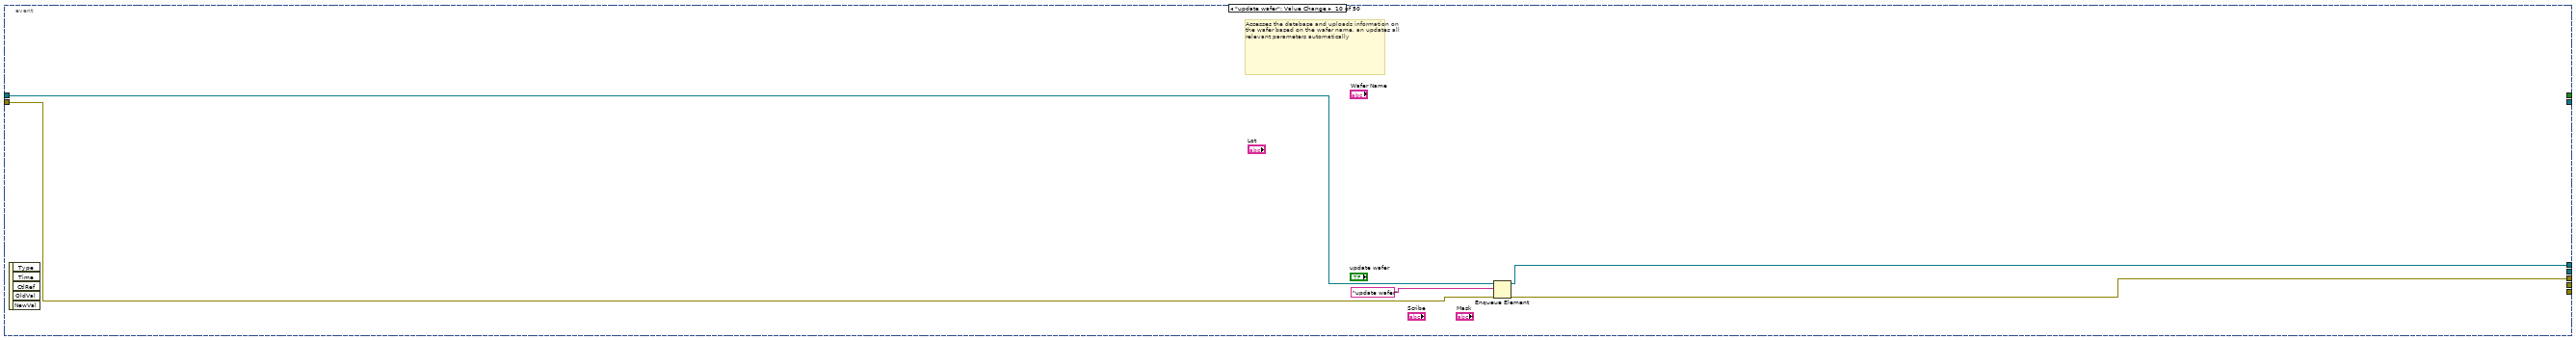
[diagram p13: hidden frame]
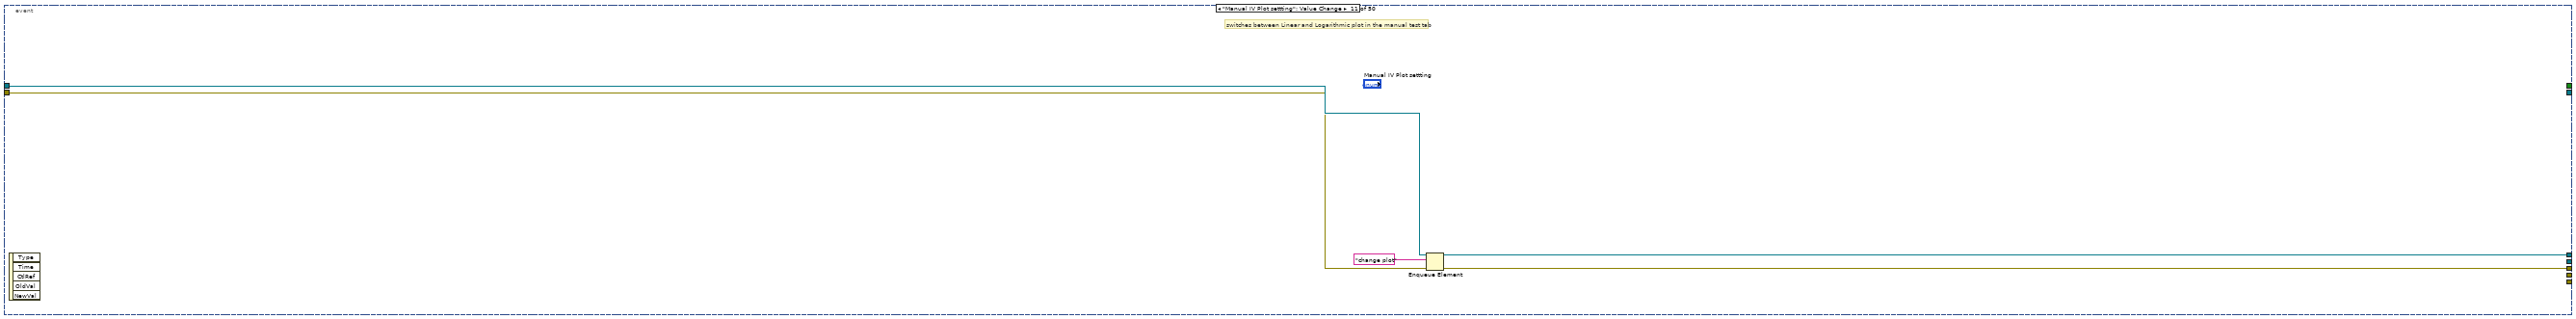
[diagram p14: hidden frame]
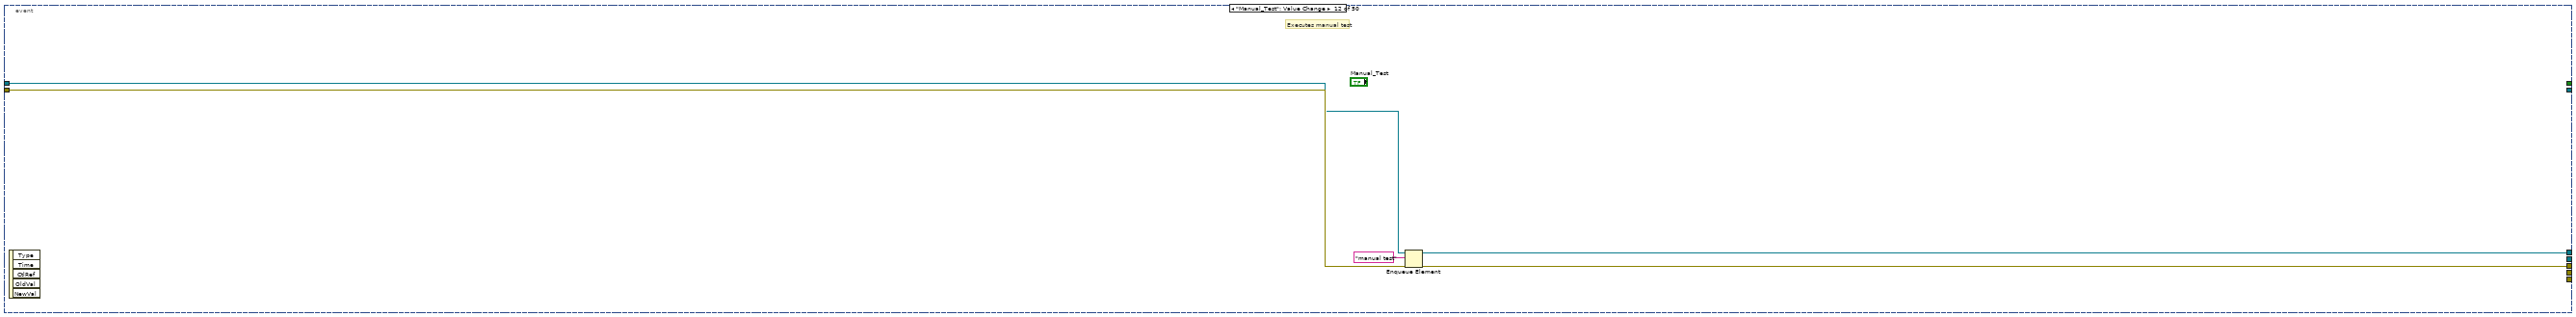
[diagram p15: hidden frame]
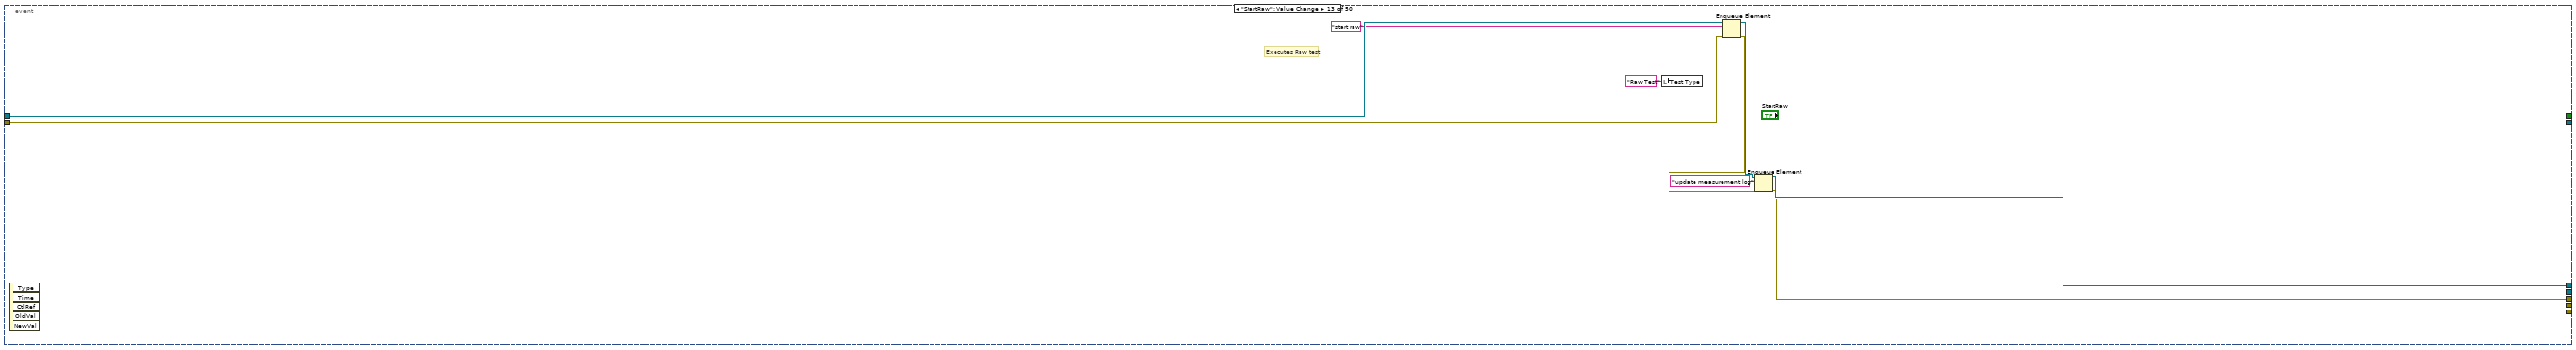
[diagram p16: hidden frame]
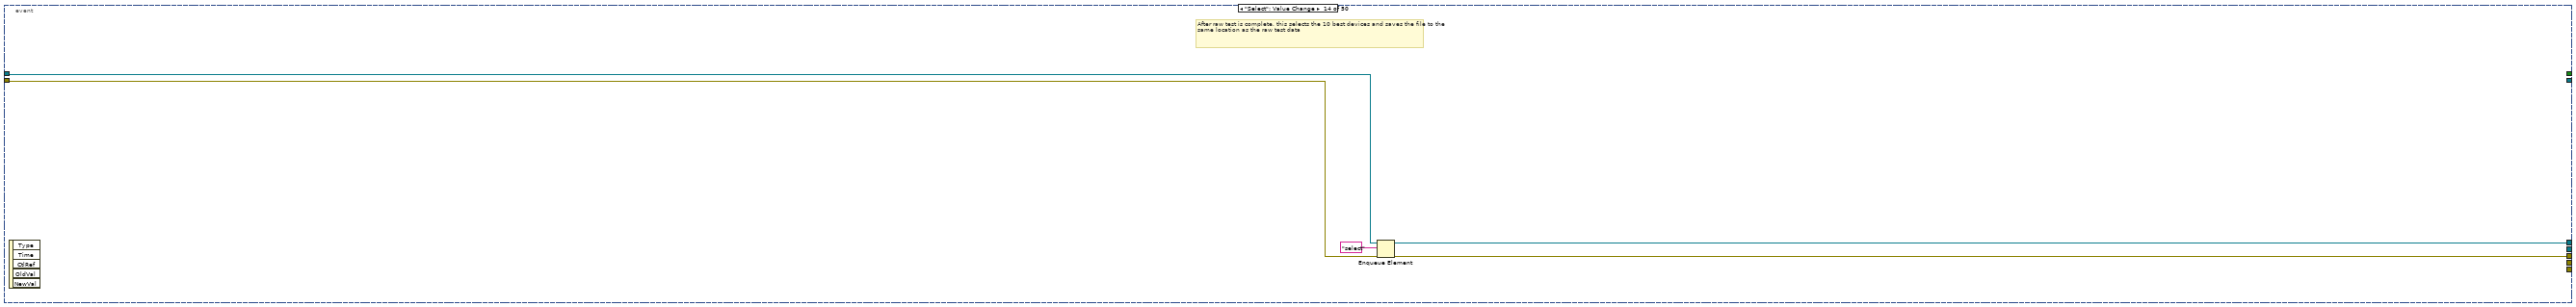
[diagram p17: hidden frame]
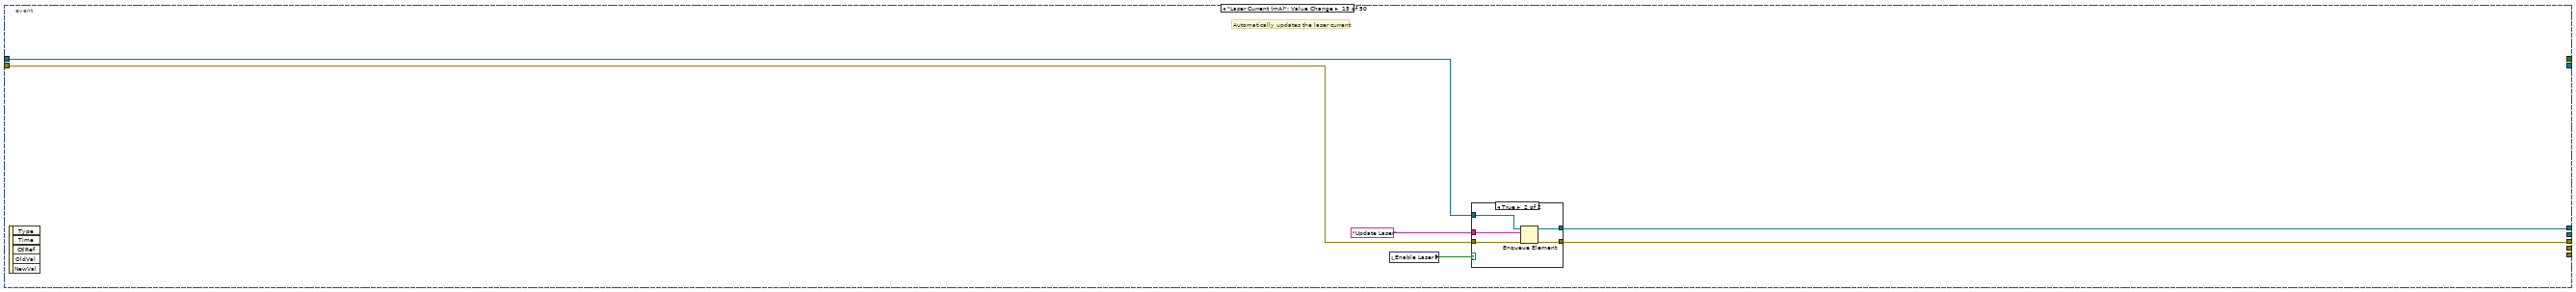
[diagram p18: hidden frame]
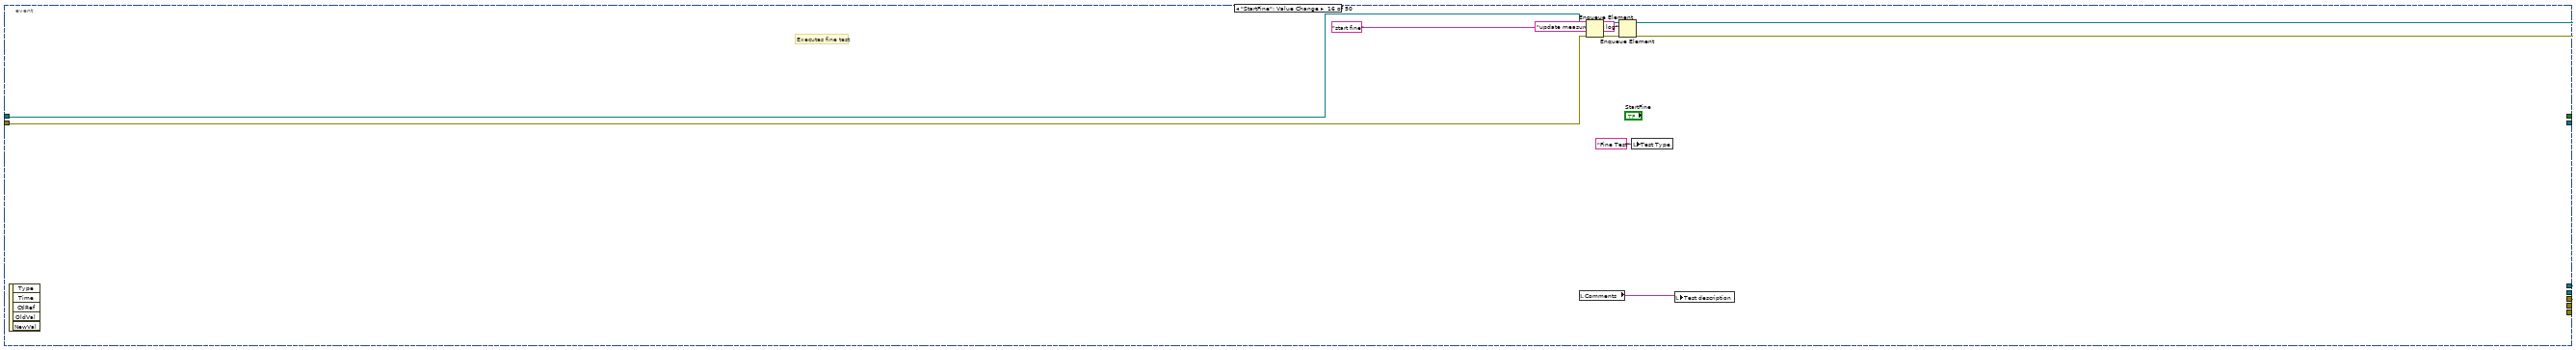
[diagram p20: hidden frame]
diagram:
  n1 = flat-sequence {
    tunnel: ["error in (no error)"] -> w1
    tunnel: w1 -> [w33]
    frame #0 {
      w18 = FALSE ("Visible")
      w16 = u32 0 ("Counter")
      n2 = local read "Temptronics VISA"() -> (w14:refnum<visa-resource-name>)
      n3 = local read "Keithley SMU"() -> (w13:refnum<visa-resource-name>)
      n4 = local read "Keysight SMU"() -> (w12:refnum<visa-resource-name>)
      n5 = local read "TL4000 In"() -> (w11:refnum<visa-resource-name>)
      n6 = local read "Enable Laser"() -> (w17:bool)
      n7 = Get Date/Time In Seconds() -> (seconds since 1Jan1904=w2:timestamp)
      n8 = case shown="True" w17 {
        frame False {
        }
        frame True {
          n9 = call "Initialize Laser.vi"("VISA Refnum in"="TL4000 In") -> ("error out"=→"Laser Error":errorcluster)  [unwired: 10 in]
        }
      }
      n10 = property on="Test Type" class="Str"("Visible"=FALSE) -> ()  [unwired: 2 in, 2 out]
      n11 = Build Array(w14, w13, w12, w11, refnum<visa-resource-name> "GPIB0::1::INSTR" ("Temptronics VISA")) -> (w9:refnum<visa-resource-name>[])
      n12 = Multiply(x="V compliance", y=0.95) -> (x*y=w20:dbl)
      n13 = local write "Current Session"(w2) -> ()
      n14 = call "VISA Channel Check.vi"("VISA Channel Array"=w9) -> ("Array"=w8:bool[])  [unwired: 10 in]
      n15 = local write "Vmax"(w20) -> ()
      n16 = Index Array(array=w8) -> (element #1=→"Temp Controller Found":bool, element #2=→"Keithley SMU Found":bool, element #3=→"Keysight SMU Found":bool, element #4=→"Thorlabs Laser Found":bool, element #5=→"EG Prober Found":bool)  [unwired: 5 in]
      n17 = call "getFile TestID.vi"("Path"="TestID file") -> ("TestID"=→"RawTest ID":u32)  [unwired: 9 in, 1 out]
      n18 = property on="device name w skip" class="Str"("Visible"=w18) -> ()  [unwired: 2 in, 2 out]
      n19 = property on="no file" class="Bool (strict)"("Visible"=w18) -> ()  [unwired: 2 in, 2 out]
      "Counter" <- w16
      "Laser Counter" <- w16
      "WaferCounter" <- w16
      "TempCounter" <- w16
      "Auto Temp Counter" <- w16
    }
    frame #1 {
      n20 = Obtain Queue(name (unnamed)="q", element data type="test" ("name (unnamed)"), create if not found? (T)=TRUE, error in (no error)=w33) -> (queue out=w35:refnum<queue>, error out=w34:errorcluster)  [unwired: 1 in, 1 out]
      n21 = while {
        shift-right: [w40] -> w36
        shift-left: w35 -> [w41]
        shift-right: [w38] -> w27
        shift-left: w34 -> [w39]
        stop <- w42 stop-if-true
        n22 = event shown="[21] \"make common recipe\": Value Change" {
          selector: _ -> [_ _ _ _ _ _ _ _ _ _ _ _ _ _ _ _ _ _ _ _ _ _ _ _ _ _ _ _ _ _ _ _ _ _ _ _ _ _ _ _ _ _ _ _ _ _ _ _ _ _]
          dyn-events: _ -> [_ _ _ _ _ _ _ _ _ _ _ _ _ _ _ _ _ _ _ _ _ _ _ _ _ _ _ _ _ _ _ _ _ _ _ _ _ _ _ _ _ _ _ _ _ _ _ _ _ _]
          timeout: -1 -> [_ _ _ _ _ _ _ _ _ _ _ _ _ _ _ _ _ _ _ _ _ _ _ _ _ _ _ _ _ _ _ _ _ _ _ _ _ _ _ _ _ _ _ _ _ _ _ _ _ _]
          tunnel: [_ TRUE _ _ _ FALSE _ _ _ _ _ _ _ _ _ _ _ _ _ _ _ _ _ _ _ _ _ _ _ _ _ _ _ _ _ _ _ _ _ _ _ _ _ _ _ _ _ _ _ _] -> w42
          tunnel: w41 -> [w46 w58 w67 w73 w78 w84 w89 w94 w98 w104 w109 w112 w123 w128 w133 w151 w156 w161 w166 w179 w301 w309 w312 w318 w323 w329 w332 w486 w491 w496 w501 w505 w510 w516 w525 w531 w536 w541 w546 w560 w565 w569 w574 w579 w585 w589 w594 w600 w608 w612]
          tunnel: [_ w62 w65 w72 _ w83 w88 w93 w96 w102 w108 w111 w118 w126 w132 w145 w154 w159 w164 w177 w304 w306 w311 w316 w321 w327 w335 w484 w489 w494 w499 w503 w508 w514 w520 w529 w534 w540 w544 w555 w564 w566 w571 w578 w582 w587 w592 w598 w604 w610] -> w40
          tunnel: w39 -> [w45 w61 w66 w71 w77 w81 w87 w92 w97 w103 w107 w113 w122 w127 w131 w150 w155 w160 w165 w178 w300 w308 w314 w317 w322 w328 w331 w485 w490 w495 w500 w504 w511 w515 w524 w530 w535 w539 w545 w559 w563 w568 w573 w577 w584 w588 w593 w599 w607 w611]
          tunnel: [w44 w60 w64 w70 _ w82 w86 _ w95 w101 w106 w110 w117 w125 w130 w144 w153 w158 w163 w176 w303 w305 w313 w315 w320 w326 w334 w483 w488 w493 w498 w502 w509 w513 w519 w528 w533 w538 w543 w553 w562 w567 w572 w576 w581 w586 w591 w597 w602 w609] -> w38
          tunnel: [_ _ _ _ w76 _ _ _ _ _ _ _ _ _ _ _ _ _ _ _ _ _ _ _ _ _ _ _ _ _ _ _ _ _ _ _ _ _ _ _ _ _ _ _ _ _ _ _ _ _] -> _
          tunnel: [_ _ _ _ w75 _ _ _ _ _ _ _ _ _ _ _ _ _ _ _ _ _ _ _ _ _ _ _ _ _ _ _ _ _ _ _ _ _ _ _ _ _ _ _ _ _ _ _ _ _] -> _
          tunnel: [w43 _ _ _ _ _ _ _ _ _ _ _ _ _ _ _ _ _ _ _ _ _ _ _ _ _ _ _ _ _ _ _ _ _ _ _ _ _ _ _ _ _ _ _ _ _ _ _ _ _] -> _
          tunnel: [_ _ _ _ _ _ _ w91 _ _ _ _ _ _ _ _ _ _ _ _ _ _ _ _ _ _ _ _ _ _ _ _ _ _ _ _ _ _ _ _ _ _ _ _ _ _ _ _ _ _] -> _
          event Timeout {
            n23 = event-data() -> ()  [unwired: 1 in, 2 out]
            n24 = First Call?() -> (First Call?: T/F=w47:bool)
            n25 = case shown="True" w47 {
              tunnel: w45 -> [w50 w56]
              tunnel: w46 -> [w52 w57]
              tunnel: [w49 w55] -> w44
              tunnel: [w51 w54] -> w43
              frame False {
                n26 = Enqueue Element(queue=w52, element="idle", error in (no error)=w50) -> (queue out=w51:refnum<queue>, error out=w49:errorcluster)  [unwired: 1 in, 1 out]
              }
              frame True {
                n27 = Enqueue Element(queue=w57, element="load file manual", error in (no error)=w56) -> (queue out=w54:refnum<queue>, error out=w55:errorcluster)  [unwired: 1 in, 1 out]
              }
            }
          }
          event "stop": Value Change {
            # "Stops the program"
            n28 = event-data() -> ()  [unwired: 1 in, 5 out]
            n29 = Enqueue Element(queue=w58, element="stop", error in (no error)=w61) -> (queue out=w62:refnum<queue>, error out=w60:errorcluster)  [unwired: 1 in, 1 out]
          }
          event "new sesh": Value Change {
            n30 = event-data() -> ()  [unwired: 1 in, 5 out]
            n31 = Enqueue Element(queue=w67, element="new session", error in (no error)=w66) -> (queue out=w65:refnum<queue>, error out=w64:errorcluster)  [unwired: 1 in, 1 out]
          }
          event "load file": Value Change {
            # "Load the mask file selected in \"Mask file manual\" on the manual test tab."
            n32 = event-data() -> ()  [unwired: 1 in, 5 out]
            n33 = Enqueue Element(queue=w73, element="load file manual", error in (no error)=w71) -> (queue out=w72:refnum<queue>, error out=w70:errorcluster)  [unwired: 1 in, 1 out]
          }
          event "J set A/cm2": Value Change {
            # "This is supposed to allow the user to manually change what they want the power density to be, and update the laser power accordingly. As of 8/18, it isnt operational as it turned out to be quite inconvenient to have to control current density rather than absolute current"
            n34 = event-data() -> ()  [unwired: 1 in, 5 out]
            n35 = Enqueue Element(queue=w78, element="Jset change", error in (no error)=w77) -> (queue out=w76:refnum<queue>, error out=w75:errorcluster)  [unwired: 1 in, 1 out]
          }
          event "Reset xy": Value Change {
            # "Reset prober to (0,0)"
            n36 = event-data() -> ()  [unwired: 1 in, 5 out]
            n37 = Enqueue Element(queue=w84, element="reset xy", error in (no error)=w81) -> (queue out=w83:refnum<queue>, error out=w82:errorcluster)  [unwired: 1 in, 1 out]
          }
          event "Reset 1st die": Value Change {
            # "This moves the prober to the first device (Die 0) of whatever mask is currently loaded. Its purpose is mainly for troubleshooting, users should generally use \"Reset to 0 0 \" instead"
            n38 = event-data() -> ()  [unwired: 1 in, 5 out]
            n39 = Enqueue Element(queue=w89, element="reset to 1st die", error in (no error)=w87) -> (queue out=w88:refnum<queue>, error out=w86:errorcluster)  [unwired: 1 in, 1 out]
          }
          event "Die Number": Value Change {
            # "When a die number is picked in the manual mask tab, this updates the target x and y to the new die's location"
            n40 = event-data() -> ()  [unwired: 1 in, 5 out]
            n41 = Enqueue Element(queue=w94, element="Die number picked", error in (no error)=w92) -> (queue out=w93:refnum<queue>, error out=w91:errorcluster)  [unwired: 1 in, 1 out]
          }
          event "Move to": Value Change {
            # "Runs the subVI that moves the prober to whatever the x and y targets are"
            n42 = event-data() -> ()  [unwired: 1 in, 5 out]
            n43 = Enqueue Element(queue=w98, element="moveto", error in (no error)=w97) -> (queue out=w96:refnum<queue>, error out=w95:errorcluster)  [unwired: 1 in, 1 out]
          }
          event "update wafer": Value Change {
            # "Accesses the database and uploads information on the wafer based on the wafer name, an updates all relevant parameters automatically"
            n44 = event-data() -> ()  [unwired: 1 in, 5 out]
            n45 = Enqueue Element(queue=w104, element="update wafer", error in (no error)=w103) -> (queue out=w102:refnum<queue>, error out=w101:errorcluster)  [unwired: 1 in, 1 out]
          }
          event "Manual IV Plot settting": Value Change {
            # "switches between Linear and Logarithmic plot in the manual test tab"
            n46 = event-data() -> ()  [unwired: 1 in, 5 out]
            n47 = Enqueue Element(queue=w109, element="change plot", error in (no error)=w107) -> (queue out=w108:refnum<queue>, error out=w106:errorcluster)  [unwired: 1 in, 1 out]
          }
          event "Manual_Test": Value Change {
            # "Executes manual test"
            n48 = event-data() -> ()  [unwired: 1 in, 5 out]
            n49 = Enqueue Element(queue=w112, element="manual test", error in (no error)=w113) -> (queue out=w111:refnum<queue>, error out=w110:errorcluster)  [unwired: 1 in, 1 out]
          }
          event "StartRaw": Value Change {
            # "Executes Raw test"
            n50 = event-data() -> ()  [unwired: 1 in, 5 out]
            n51 = local write "Test Type"("Raw Test" ("Test Type")) -> ()
            n52 = Enqueue Element(queue=w123, element="start raw", error in (no error)=w122) -> (queue out=w119:refnum<queue>, error out=w116:errorcluster)  [unwired: 1 in, 1 out]
            n53 = Enqueue Element(queue=w119, element="update measurement log", error in (no error)=w116) -> (queue out=w118:refnum<queue>, error out=w117:errorcluster)  [unwired: 1 in, 1 out]
          }
          event "Select": Value Change {
            # "After raw test is complete, this selects the 10 best devices and saves the file to the same location as the raw test data"
            n54 = event-data() -> ()  [unwired: 1 in, 5 out]
            n55 = Enqueue Element(queue=w128, element="select", error in (no error)=w127) -> (queue out=w126:refnum<queue>, error out=w125:errorcluster)  [unwired: 1 in, 1 out]
          }
          event "Laser Current (mA)": Value Change {
            # "Automatically updates the laser current"
            n56 = event-data() -> ()  [unwired: 1 in, 5 out]
            n57 = local read "Enable Laser"() -> (w129:bool)
            n58 = case shown="True" w129 {
              tunnel: "Update Laser" ("element") -> [_ w141]
              tunnel: w133 -> [w136 w140]
              tunnel: [w136 w139] -> w132
              tunnel: w131 -> [w135 w138]
              tunnel: [w135 w137] -> w130
              frame False {
              }
              frame True {
                n59 = Enqueue Element(queue=w140, element=w141, error in (no error)=w138) -> (queue out=w139:refnum<queue>, error out=w137:errorcluster)  [unwired: 1 in, 1 out]
              }
            }
          }
          event "StartFine": Value Change {
            # "Executes fine test"
            n60 = event-data() -> ()  [unwired: 1 in, 5 out]
            n61 = local read "Comments"() -> (w142:string)
            n62 = Enqueue Element(queue=w151, element="start fine", error in (no error)=w150) -> (queue out=w147:refnum<queue>, error out=w146:errorcluster)  [unwired: 1 in, 1 out]
            n63 = Enqueue Element(queue=w147, element="update measurement log", error in (no error)=w146) -> (queue out=w145:refnum<queue>, error out=w144:errorcluster)  [unwired: 1 in, 1 out]
            n64 = local write "Test Type"("Fine Test" ("Test Type")) -> ()
            n65 = local write "Test description"(w142) -> ()
          }
          event "Mask File Raw": Value Change {
            # "When raw mask is updated, it asks if you want to update the manual test mask as well"
            n66 = event-data() -> ()  [unwired: 1 in, 5 out]
            n67 = Enqueue Element(queue=w156, element="raw mask updated", error in (no error)=w155) -> (queue out=w154:refnum<queue>, error out=w153:errorcluster)  [unwired: 1 in, 1 out]
          }
          event "Mask File Manual": Value Change {
            # "When manual mask is updated, it asks if the user would want to update the raw test as well"
            n68 = event-data() -> ()  [unwired: 1 in, 5 out]
            n69 = Enqueue Element(queue=w161, element="mask manual update", error in (no error)=w160) -> (queue out=w159:refnum<queue>, error out=w158:errorcluster)  [unwired: 1 in, 1 out]
          }
          event "Load raw": Value Change {
            # "Gives the user the option to pick a raw data file, and then displays that on the graphical display on the raw test tab"
            n70 = event-data() -> ()  [unwired: 1 in, 5 out]
            n71 = Enqueue Element(queue=w166, element="load raw data", error in (no error)=w165) -> (queue out=w164:refnum<queue>, error out=w163:errorcluster)  [unwired: 1 in, 1 out]
          }
          event "Start auto": Value Change {
            # "Exectues Auto Test:\n1) For loop - repeats as many times as there are test names.\n2) Skip raw? - check to see if the user would like to skip raw test (see guide). If raw test is skipped, the variable \"Raw test skipped\" is set to TRUE\n3) Case Structure - If the laser is enabled, the program sets the laser current to zero prior to the raw test.; if the user has elected to disable the laser, then this step is skipped\n4) Start Raw - The raw test is executed. If the raw test is skipped, this element is still queued up, and the entire test is skipped within the event structure. This is because the timing didn't work when I tried to skip the raw test here.\n5)Select - This selects the best ten devices. Again, if raw test is skipped, this still is added to the queue, and is skipped in the event structure\n6) Double Case Structure - There are 4 options\n         a) Laser Disabled & Only Raw test TRUE -  The entire fine test portion is skipped\n         b)  Laser Disabled & Only Raw Test FALSE - The fine test is run ONLY dark. Find best devices mask still queues up, but only runs if the raw test has been skipped\n         c) Laser Enabled - Only Raw Test TRUE - the entire fine test is still skipped\n         d) Laser Enabled - Only Raw Test FALSE - fine test is run through a for loop that repeats the test for every laser power in the Laser List. Find best devices mask only runs if the raw test is skipped.\n7) Reset skip - replaces the (skip) on the device name if the raw test was skipped, as for the duration of the test it had to be removed. This is in case multiple tests are to be run - so the user doesn't have to keep specifying that they want to skip the raw test every time they run the auto test\n8) Zero/Update Laser - Turns the laser to zero after the test is complete\n9) Update Measurement log - automatically updates the measurement lof with the details of the test"
            n72 = event-data() -> ()  [unwired: 1 in, 1 out]
            n73 = local read "Test description"() -> (w174:string)
            n74 = property on="Auto Temperature List" class="LstBox (strict)"() -> ("Item Names"=w172:string[])  [unwired: 2 in, 2 out]
            n75 = local write "Test Type"("Auto Test" ("Test Type")) -> ()
            n76 = local write "Comments"(w174) -> ()
            n77 = for {
              tunnel: w179 -> [w194]
              tunnel: w178 -> [w193]
              tunnel: [w197] -> w171
              tunnel: [w196] -> w169
              tunnel: w172 -> [_] mode=indexing
              n78 = local read "Temp Controller Found"() -> (w190:bool)
              n79 = case shown="False" w190 {
                tunnel: w194 -> [w205 w216]
                tunnel: w193 -> [w204 w215]
                tunnel: [w205 w214] -> w192
                tunnel: [w204 w213] -> w191
                frame False {
                }
                frame True {
                  n80 = Enqueue Element(queue=w216, element="select temperature", error in (no error)=w215) -> (queue out=w210:refnum<queue>, error out=w208:errorcluster)  [unwired: 1 in, 1 out]
                  n81 = Enqueue Element(queue=w210, element="update temperature", error in (no error)=w208) -> (queue out=w209:refnum<queue>, error out=w207:errorcluster)  [unwired: 1 in, 1 out]
                  n82 = Enqueue Element(queue=w209, element="wait for temperature", error in (no error)=w207) -> (queue out=w214:refnum<queue>, error out=w213:errorcluster)  [unwired: 1 in, 1 out]
                }
              }
              n83 = property on="Test List" class="LstBox (strict)"() -> ("Item Names"=w203:string[])  [unwired: 2 in, 2 out]
              n84 = for {
                shift-right: [w217] -> w200
                shift-left: w191 -> [w225]
                shift-right: [w220] -> w201
                shift-left: w192 -> [w226]
                tunnel: w203 -> [_] mode=indexing
                n85 = Enqueue Element(queue=w226, element="skip raw?", error in (no error)=w225) -> (queue out=w224:refnum<queue>, error out=w223:errorcluster)  [unwired: 1 in, 1 out]
                n86 = Enqueue Element(queue=w224, element="pick device", error in (no error)=w223) -> (queue out=w232:refnum<queue>, error out=w231:errorcluster)  [unwired: 1 in, 1 out]
                n87 = case shown="False" FALSE {
                  tunnel: w232 -> [w285 w298]
                  tunnel: w231 -> [w284 w299]
                  tunnel: [w282 w298] -> w230
                  tunnel: [w281 w299] -> w229
                  frame False {
                    n88 = local read "Enable Laser"() -> (w283:bool)
                    n89 = case shown="True" w283 {
                      tunnel: [w289 w297] -> w287
                      tunnel: [w288 w296] -> w286
                      tunnel: w285 -> [w289 w294]
                      tunnel: w284 -> [w288 w292]
                      frame False {
                      }
                      frame True {
                        n90 = Enqueue Element(queue=w294, element="Zero Laser", error in (no error)=w292) -> (queue out=w293:refnum<queue>, error out=w291:errorcluster)  [unwired: 1 in, 1 out]
                        n91 = Enqueue Element(queue=w293, element="Update Laser", error in (no error)=w291) -> (queue out=w297:refnum<queue>, error out=w296:errorcluster)  [unwired: 1 in, 1 out]
                      }
                    }
                    n92 = Enqueue Element(queue=w287, element="start raw", error in (no error)=w286) -> (queue out=w278:refnum<queue>, error out=w277:errorcluster)  [unwired: 1 in, 1 out]
                    n93 = Enqueue Element(queue=w278, element="select", error in (no error)=w277) -> (queue out=w282:refnum<queue>, error out=w281:errorcluster)  [unwired: 1 in, 1 out]
                  }
                  frame True {
                  }
                }
                n94 = local read "Enable Laser"() -> (w227:bool)
                n95 = case shown="True" w227 {
                  tunnel: [w239 w255] -> w221
                  tunnel: [w238 w254] -> w218
                  tunnel: w230 -> [w237 w253]
                  tunnel: w229 -> [w236 w252]
                  frame False {
                    n96 = local read "Only Raw Test"() -> (w234:bool)
                    n97 = Not(x=w234) -> (.not. x?=w235:bool)
                    n98 = case shown="False" w235 {
                      tunnel: [w241 w249] -> w239
                      tunnel: [w240 w248] -> w238
                      tunnel: w237 -> [w241 w247]
                      tunnel: w236 -> [w240 w245]
                      frame False {
                      }
                      frame True {
                        n99 = Enqueue Element(queue=w247, element="find best devices mask", error in (no error)=w245) -> (queue out=w246:refnum<queue>, error out=w244:errorcluster)  [unwired: 1 in, 1 out]
                        n100 = Enqueue Element(queue=w246, element="start fine", error in (no error)=w244) -> (queue out=w249:refnum<queue>, error out=w248:errorcluster)  [unwired: 1 in, 1 out]
                      }
                    }
                  }
                  frame True {
                    n101 = Not(x="Only Raw Test") -> (.not. x?=w250:bool)
                    n102 = case shown="True" w250 {
                      tunnel: [w257 w262] -> w255
                      tunnel: [w256 w261] -> w254
                      tunnel: w253 -> [w257 w260]
                      tunnel: w252 -> [w256 w259]
                      frame False {
                      }
                      frame True {
                        n103 = property on="Laser List" class="LstBox (strict)"() -> ("Item Names"=w258:string[])  [unwired: 2 in, 2 out]
                        n104 = for {
                          tunnel: [w276] -> w262
                          tunnel: [w275] -> w261
                          tunnel: w260 -> [w271]
                          tunnel: w259 -> [w274]
                          tunnel: w258 -> [_] mode=indexing
                          n105 = Enqueue Element(queue=w271, element="pick laser", error in (no error)=w274) -> (queue out=w270:refnum<queue>, error out=w272:errorcluster)  [unwired: 1 in, 1 out]
                          n106 = Enqueue Element(queue=w270, element="Update Laser", error in (no error)=w272) -> (queue out=w265:refnum<queue>, error out=w268:errorcluster)  [unwired: 1 in, 1 out]
                          n107 = Enqueue Element(queue=w265, element="find best devices mask", error in (no error)=w268) -> (queue out=w266:refnum<queue>, error out=w267:errorcluster)  [unwired: 1 in, 1 out]
                          n108 = Enqueue Element(queue=w266, element="start fine", error in (no error)=w267) -> (queue out=w276:refnum<queue>, error out=w275:errorcluster)  [unwired: 1 in, 1 out]
                        }
                      }
                    }
                  }
                }
                n109 = Enqueue Element(queue=w221, element="reset skip", error in (no error)=w218) -> (queue out=w220:refnum<queue>, error out=w217:errorcluster)  [unwired: 1 in, 1 out]
              }
              n110 = Enqueue Element(queue=w201, element="Zero Laser", error in (no error)=w200) -> (queue out=w199:refnum<queue>, error out=w198:errorcluster)  [unwired: 1 in, 1 out]
              n111 = Enqueue Element(queue=w199, element="update laser", error in (no error)=w198) -> (queue out=w197:refnum<queue>, error out=w196:errorcluster)  [unwired: 1 in, 1 out]
            }
            n112 = local read "Temp Controller Found"() -> (w167:bool)
            n113 = case shown="False" w167 {
              tunnel: w171 -> [w181 w189]
              tunnel: [w181 w187] -> w170
              tunnel: w169 -> [w180 w186]
              tunnel: [w180 w184] -> w168
              frame False {
              }
              frame True {
                n114 = Enqueue Element(queue=w189, element="temp to 25", error in (no error)=w186) -> (queue out=w188:refnum<queue>, error out=w185:errorcluster)  [unwired: 1 in, 1 out]
                n115 = Enqueue Element(queue=w188, element="update temperature", error in (no error)=w185) -> (queue out=w187:refnum<queue>, error out=w184:errorcluster)  [unwired: 1 in, 1 out]
              }
            }
            n116 = Enqueue Element(queue=w170, element="update measurement log", error in (no error)=w168) -> (queue out=w177:refnum<queue>, error out=w176:errorcluster)  [unwired: 1 in, 1 out]
          }
          event "select preset recipe": Value Change {
            n117 = event-data() -> ()  [unwired: 1 in, 5 out]
            n118 = Enqueue Element(queue=w301, element="select preset sweep recipe", error in (no error)=w300) -> (queue out=w304:refnum<queue>, error out=w303:errorcluster)  [unwired: 1 in, 1 out]
          }
          event "make common recipe": Value Change {
            n119 = event-data() -> ()  [unwired: 1 in, 5 out]
            n120 = Enqueue Element(queue=w309, element="make common recipe", error in (no error)=w308) -> (queue out=w306:refnum<queue>, error out=w305:errorcluster)  [unwired: 1 in, 1 out]
          }
          event "Generate Report": Value Change {
            n121 = event-data() -> ()  [unwired: 1 in, 5 out]
            n122 = Enqueue Element(queue=w312, element="generate prelim report", error in (no error)=w314) -> (queue out=w311:refnum<queue>, error out=w313:errorcluster)  [unwired: 1 in, 1 out]
          }
          event "Add to Temp Auto": Value Change {
            n123 = event-data() -> ()  [unwired: 1 in, 5 out]
            n124 = Enqueue Element(queue=w318, element="add temp auto", error in (no error)=w317) -> (queue out=w316:refnum<queue>, error out=w315:errorcluster)  [unwired: 1 in, 1 out]
          }
          event "Remove from Temp Auto": Value Change {
            n125 = event-data() -> ()  [unwired: 1 in, 5 out]
            n126 = Enqueue Element(queue=w323, element="remove temp auto", error in (no error)=w322) -> (queue out=w321:refnum<queue>, error out=w320:errorcluster)  [unwired: 1 in, 1 out]
          }
          event "Clear temp list Auto": Value Change {
            n127 = event-data() -> ()  [unwired: 1 in, 5 out]
            n128 = Enqueue Element(queue=w329, element="clear temp auto", error in (no error)=w328) -> (queue out=w327:refnum<queue>, error out=w326:errorcluster)  [unwired: 1 in, 1 out]
          }
          event "begin lot test": Value Change {
            n129 = event-data() -> ()  [unwired: 1 in, 5 out]
            n130 = local write "Test Type"("Lot Test" ("Test Type")) -> ()
            n131 = property on="Wafer List" class="LstBox (strict)"() -> ("Item Names"=w333:string[])  [unwired: 2 in, 2 out]
            n132 = for {
              tunnel: w333 -> [_] mode=indexing
              shift-right: [w343] -> w335
              shift-left: w332 -> [w362]
              shift-right: [w342] -> w334
              shift-left: w331 -> [w361]
              i -> [w360]
              n133 = Equal?(x=w360, y=0) -> (x = y?=w358:bool)
              n134 = And(x="First Wafer Loaded?", y=w358) -> (x .and. y?=w356:bool)
              n135 = case shown="False" w356 {
                tunnel: w362 -> [w469 w481]
                tunnel: w361 -> [w468 w480]
                tunnel: [w467 w481] -> w355
                tunnel: [w466 w480] -> w350
                frame False {
                  n136 = Enqueue Element(queue=w469, element="load wafer", error in (no error)=w468) -> (queue out=w474:refnum<queue>, error out=w473:errorcluster)  [unwired: 1 in, 1 out]
                  n137 = Enqueue Element(queue=w474, element="wait", error in (no error)=w473) -> (queue out=w472:refnum<queue>, error out=w471:errorcluster)  [unwired: 1 in, 1 out]
                  n138 = Enqueue Element(queue=w472, element="profile z", error in (no error)=w471) -> (queue out=w477:refnum<queue>, error out=w476:errorcluster)  [unwired: 1 in, 1 out]
                  n139 = Enqueue Element(queue=w477, element="auto align", error in (no error)=w476) -> (queue out=w467:refnum<queue>, error out=w466:errorcluster)  [unwired: 1 in, 1 out]
                }
                frame True {
                }
              }
              n140 = Enqueue Element(queue=w355, element="desired wafer to current wafer", error in (no error)=w350) -> (queue out=w354:refnum<queue>, error out=w351:errorcluster)  [unwired: 1 in, 1 out]
              n141 = Enqueue Element(queue=w354, element="update wafer", error in (no error)=w351) -> (queue out=w353:refnum<queue>, error out=w352:errorcluster)  [unwired: 1 in, 1 out]
              n142 = property on="Auto Temperature List" class="LstBox (strict)"() -> ("Item Names"=w336:string[])  [unwired: 2 in, 2 out]
              n143 = for {
                tunnel: [w375] -> w346
                tunnel: [w374] -> w339
                tunnel: w353 -> [w373]
                tunnel: w352 -> [w372]
                tunnel: w336 -> [_] mode=indexing
                n144 = Enqueue Element(queue=w373, element="select temperature", error in (no error)=w372) -> (queue out=w371:refnum<queue>, error out=w370:errorcluster)  [unwired: 1 in, 1 out]
                n145 = Enqueue Element(queue=w371, element="update temperature", error in (no error)=w370) -> (queue out=w369:refnum<queue>, error out=w368:errorcluster)  [unwired: 1 in, 1 out]
                n146 = property on="Test List" class="LstBox (strict)"() -> ("Item Names"=w381:string[])  [unwired: 2 in, 2 out]
                n147 = Enqueue Element(queue=w369, element="wait for temperature", error in (no error)=w368) -> (queue out=w367:refnum<queue>, error out=w366:errorcluster)  [unwired: 1 in, 1 out]
                n148 = for {
                  shift-right: [w386] -> w376
                  shift-left: w366 -> [w391]
                  shift-right: [w387] -> w377
                  shift-left: w367 -> [w392]
                  tunnel: w381 -> [_] mode=indexing
                  # "Executes Lot Test\n1) First Wafer Loaded? - If the first wafer in the lot is already on the chuck, the user selects this and the loading wafer steps are skipped for the first iteration of the the for loop.\n2) Load wafer - loads the wafer from the cassette to the chuck\n3)wait - waits ten seconds  - if the profile command comes while the cwafer is still being loaded the probe station gives an error\n4) Profile z and autoalign - completes the rest of the loading procedure\n5) desired wafer to current wafer - changes wafer name to the next on on the \"Wafer List\"\n6) update wafer - update wafer info\n7) Runs auto test (see auto test tab)"
                  n149 = Enqueue Element(queue=w392, element="skip raw?", error in (no error)=w391) -> (queue out=w390:refnum<queue>, error out=w389:errorcluster)  [unwired: 1 in, 1 out]
                  n150 = Enqueue Element(queue=w390, element="pick device", error in (no error)=w389) -> (queue out=w398:refnum<queue>, error out=w397:errorcluster)  [unwired: 1 in, 1 out]
                  n151 = case shown="False" FALSE {
                    tunnel: w398 -> [w451 w464]
                    tunnel: w397 -> [w450 w465]
                    tunnel: [w448 w464] -> w396
                    tunnel: [w447 w465] -> w395
                    frame False {
                      n152 = local read "Enable Laser"() -> (w449:bool)
                      n153 = case shown="True" w449 {
                        tunnel: [w455 w463] -> w453
                        tunnel: [w454 w462] -> w452
                        tunnel: w451 -> [w455 w460]
                        tunnel: w450 -> [w454 w458]
                        frame False {
                        }
                        frame True {
                          n154 = Enqueue Element(queue=w460, element="Zero Laser", error in (no error)=w458) -> (queue out=w459:refnum<queue>, error out=w457:errorcluster)  [unwired: 1 in, 1 out]
                          n155 = Enqueue Element(queue=w459, element="Update Laser", error in (no error)=w457) -> (queue out=w463:refnum<queue>, error out=w462:errorcluster)  [unwired: 1 in, 1 out]
                        }
                      }
                      n156 = Enqueue Element(queue=w453, element="start raw", error in (no error)=w452) -> (queue out=w444:refnum<queue>, error out=w443:errorcluster)  [unwired: 1 in, 1 out]
                      n157 = Enqueue Element(queue=w444, element="select", error in (no error)=w443) -> (queue out=w448:refnum<queue>, error out=w447:errorcluster)  [unwired: 1 in, 1 out]
                    }
                    frame True {
                    }
                  }
                  n158 = local read "Enable Laser"() -> (w393:bool)
                  n159 = case shown="True" w393 {
                    tunnel: [w405 w421] -> w384
                    tunnel: [w404 w420] -> w385
                    tunnel: w396 -> [w403 w419]
                    tunnel: w395 -> [w402 w418]
                    frame False {
                      n160 = local read "Only Raw Test"() -> (w400:bool)
                      n161 = Not(x=w400) -> (.not. x?=w401:bool)
                      n162 = case shown="False" w401 {
                        tunnel: [w407 w415] -> w405
                        tunnel: [w406 w414] -> w404
                        tunnel: w403 -> [w407 w413]
                        tunnel: w402 -> [w406 w411]
                        frame False {
                        }
                        frame True {
                          n163 = Enqueue Element(queue=w413, element="find best devices mask", error in (no error)=w411) -> (queue out=w412:refnum<queue>, error out=w410:errorcluster)  [unwired: 1 in, 1 out]
                          n164 = Enqueue Element(queue=w412, element="start fine", error in (no error)=w410) -> (queue out=w415:refnum<queue>, error out=w414:errorcluster)  [unwired: 1 in, 1 out]
                        }
                      }
                    }
                    frame True {
                      n165 = local read "Only Raw Test"() -> (w416:bool)
                      n166 = Not(x=w416) -> (.not. x?=w417:bool)
                      n167 = case shown="True" w417 {
                        tunnel: [w423 w428] -> w421
                        tunnel: [w422 w427] -> w420
                        tunnel: w419 -> [w423 w426]
                        tunnel: w418 -> [w422 w425]
                        frame False {
                        }
                        frame True {
                          n168 = property on="Laser List" class="LstBox (strict)"() -> ("Item Names"=w424:string[])  [unwired: 2 in, 2 out]
                          n169 = for {
                            tunnel: [w442] -> w428
                            tunnel: [w441] -> w427
                            tunnel: w426 -> [w437]
                            tunnel: w425 -> [w440]
                            tunnel: w424 -> [_] mode=indexing
                            n170 = Enqueue Element(queue=w437, element="pick laser", error in (no error)=w440) -> (queue out=w436:refnum<queue>, error out=w438:errorcluster)  [unwired: 1 in, 1 out]
                            n171 = Enqueue Element(queue=w436, element="Update Laser", error in (no error)=w438) -> (queue out=w431:refnum<queue>, error out=w434:errorcluster)  [unwired: 1 in, 1 out]
                            n172 = Enqueue Element(queue=w431, element="find best devices mask", error in (no error)=w434) -> (queue out=w432:refnum<queue>, error out=w433:errorcluster)  [unwired: 1 in, 1 out]
                            n173 = Enqueue Element(queue=w432, element="start fine", error in (no error)=w433) -> (queue out=w442:refnum<queue>, error out=w441:errorcluster)  [unwired: 1 in, 1 out]
                          }
                        }
                      }
                    }
                  }
                  n174 = Enqueue Element(queue=w384, element="reset skip", error in (no error)=w385) -> (queue out=w387:refnum<queue>, error out=w386:errorcluster)  [unwired: 1 in, 1 out]
                }
                n175 = Enqueue Element(queue=w377, element="Zero Laser", error in (no error)=w376) -> (queue out=w380:refnum<queue>, error out=w379:errorcluster)  [unwired: 1 in, 1 out]
                n176 = Enqueue Element(queue=w380, element="update laser", error in (no error)=w379) -> (queue out=w375:refnum<queue>, error out=w374:errorcluster)  [unwired: 1 in, 1 out]
              }
              n177 = Enqueue Element(queue=w346, element="temp to 25", error in (no error)=w339) -> (queue out=w345:refnum<queue>, error out=w340:errorcluster)  [unwired: 1 in, 1 out]
              n178 = Enqueue Element(queue=w345, element="update temperature", error in (no error)=w340) -> (queue out=w344:refnum<queue>, error out=w341:errorcluster)  [unwired: 1 in, 1 out]
              n179 = Enqueue Element(queue=w344, element="update measurement log", error in (no error)=w341) -> (queue out=w343:refnum<queue>, error out=w342:errorcluster)  [unwired: 1 in, 1 out]
            }
          }
          event "update temp": Value Change {
            # "Gives the VISA commands to update chuck temperature"
            n180 = event-data() -> ()  [unwired: 1 in, 5 out]
            n181 = Enqueue Element(queue=w486, element="update temperature", error in (no error)=w485) -> (queue out=w484:refnum<queue>, error out=w483:errorcluster)  [unwired: 1 in, 1 out]
          }
          event "Add to Temp": Value Change {
            # "adds value from desired temperature to temperature list"
            n182 = event-data() -> ()  [unwired: 1 in, 5 out]
            n183 = Enqueue Element(queue=w491, element="add to temp list", error in (no error)=w490) -> (queue out=w489:refnum<queue>, error out=w488:errorcluster)  [unwired: 1 in, 1 out]
          }
          event "Remove from Temp": Value Change {
            # "removes highlighted value from temperature list"
            n184 = event-data() -> ()  [unwired: 1 in, 5 out]
            n185 = Enqueue Element(queue=w496, element="remove from temp list", error in (no error)=w495) -> (queue out=w494:refnum<queue>, error out=w493:errorcluster)  [unwired: 1 in, 1 out]
          }
          event "Clear temp list": Value Change {
            # "removes all values from temperature list"
            n186 = event-data() -> ()  [unwired: 1 in, 5 out]
            n187 = Enqueue Element(queue=w501, element="clear temp list", error in (no error)=w500) -> (queue out=w499:refnum<queue>, error out=w498:errorcluster)  [unwired: 1 in, 1 out]
          }
          event "load file for temp series": Value Change {
            # "works the same as loading manual mask file, but this is just in the temperature series tab"
            n188 = event-data() -> ()  [unwired: 1 in, 5 out]
            n189 = Enqueue Element(queue=w505, element="load file for temp", error in (no error)=w504) -> (queue out=w503:refnum<queue>, error out=w502:errorcluster)  [unwired: 1 in, 1 out]
          }
          event "move prober 2": Value Change {
            # "does the same as \"moveto\" from a different button"
            n190 = event-data() -> ()  [unwired: 1 in, 5 out]
            n191 = Enqueue Element(queue=w510, element="moveto", error in (no error)=w511) -> (queue out=w508:refnum<queue>, error out=w509:errorcluster)  [unwired: 1 in, 1 out]
          }
          event "Desired Device": Value Change {
            # "Does the same as \"Die number changed\" but from the temperature series tab"
            n192 = event-data() -> ()  [unwired: 1 in, 5 out]
            n193 = Enqueue Element(queue=w516, element="desired device change", error in (no error)=w515) -> (queue out=w514:refnum<queue>, error out=w513:errorcluster)  [unwired: 1 in, 1 out]
          }
          event "Start temp": Value Change {
            # "Begins Temperature Series\n1) Selects Temperature - updates current temprature from temp list\n2) Update temperature - writes current temperature to Temptronic TEC\n3) Wait fr temperature - waits until the temperature has settled on the correct value\n4) begin temperature series - runs a few fine tests with different tempreatures (in progress)"
            n194 = event-data() -> ()  [unwired: 1 in, 5 out]
            n195 = local read "Comments Temp"() -> (w517:string)
            n196 = local write "Test Type"("Temperature Test" ("Test Type")) -> ()
            n197 = local write "Comments"(w517) -> ()
            n198 = Enqueue Element(queue=w525, element="begin temperature series", error in (no error)=w524) -> (queue out=w522:refnum<queue>, error out=w521:errorcluster)  [unwired: 1 in, 1 out]
            n199 = Enqueue Element(queue=w522, element="update measurement log", error in (no error)=w521) -> (queue out=w520:refnum<queue>, error out=w519:errorcluster)  [unwired: 1 in, 1 out]
          }
          event "Refresh Device": Value Change {
            # "This is supposed to populate the device mane list from the given mask file. As of 8/5/18 it isn't working properly"
            n200 = event-data() -> ()  [unwired: 1 in, 5 out]
            n201 = Enqueue Element(queue=w531, element="refresh device names", error in (no error)=w530) -> (queue out=w529:refnum<queue>, error out=w528:errorcluster)  [unwired: 1 in, 1 out]
          }
          event "Add to list": Value Change {
            # "Adds device name value to test list"
            n202 = event-data() -> ()  [unwired: 1 in, 5 out]
            n203 = Enqueue Element(queue=w536, element="add to list", error in (no error)=w535) -> (queue out=w534:refnum<queue>, error out=w533:errorcluster)  [unwired: 1 in, 1 out]
          }
          event "Remove from List": Value Change {
            # "removes highlighted walue from test list"
            n204 = event-data() -> ()  [unwired: 1 in, 5 out]
            n205 = Enqueue Element(queue=w541, element="remove from list", error in (no error)=w539) -> (queue out=w540:refnum<queue>, error out=w538:errorcluster)  [unwired: 1 in, 1 out]
          }
          event "Clear List": Value Change {
            # "removes all entries from test list"
            n206 = event-data() -> ()  [unwired: 1 in, 5 out]
            n207 = Enqueue Element(queue=w546, element="clear list", error in (no error)=w545) -> (queue out=w544:refnum<queue>, error out=w543:errorcluster)  [unwired: 1 in, 1 out]
          }
          event "Load Wafer": Value Change {
            # "Loads wafer and performs profilng and auto alignment procedures"
            n208 = event-data() -> ()  [unwired: 1 in, 5 out]
            n209 = Enqueue Element(queue=w560, element="load wafer", error in (no error)=w559) -> (queue out=w551:refnum<queue>, error out=w550:errorcluster)  [unwired: 1 in, 1 out]
            n210 = Enqueue Element(queue=w551, element="wait", error in (no error)=w550) -> (queue out=w549:refnum<queue>, error out=w548:errorcluster)  [unwired: 1 in, 1 out]
            n211 = Enqueue Element(queue=w549, element="profile z", error in (no error)=w548) -> (queue out=w556:refnum<queue>, error out=w554:errorcluster)  [unwired: 1 in, 1 out]
            n212 = Enqueue Element(queue=w556, element="auto align", error in (no error)=w554) -> (queue out=w555:refnum<queue>, error out=w553:errorcluster)  [unwired: 1 in, 1 out]
          }
          event "Profile Z": Value Change {
            # "Performs just the z profile"
            n213 = event-data() -> ()  [unwired: 1 in, 5 out]
            n214 = Enqueue Element(queue=w565, element="profile z", error in (no error)=w563) -> (queue out=w564:refnum<queue>, error out=w562:errorcluster)  [unwired: 1 in, 1 out]
          }
          event "Add to Laser": Value Change {
            # "adds desired laser value to laser list"
            n215 = event-data() -> ()  [unwired: 1 in, 5 out]
            n216 = Enqueue Element(queue=w569, element="add to laser list", error in (no error)=w568) -> (queue out=w566:refnum<queue>, error out=w567:errorcluster)  [unwired: 1 in, 1 out]
          }
          event "Remove from Laser List": Value Change {
            # "removes highlighted value from laser list"
            n217 = event-data() -> ()  [unwired: 1 in, 5 out]
            n218 = Enqueue Element(queue=w574, element="remove from laser list", error in (no error)=w573) -> (queue out=w571:refnum<queue>, error out=w572:errorcluster)  [unwired: 1 in, 1 out]
          }
          event "Clear Laser List": Value Change {
            # "removes all entries from laser list"
            n219 = event-data() -> ()  [unwired: 1 in, 5 out]
            n220 = Enqueue Element(queue=w579, element="clear laser list", error in (no error)=w577) -> (queue out=w578:refnum<queue>, error out=w576:errorcluster)  [unwired: 1 in, 1 out]
          }
          event "Add to wafer list": Value Change {
            # "Adds desired value to wafer list"
            n221 = event-data() -> ()  [unwired: 1 in, 5 out]
            n222 = Enqueue Element(queue=w585, element="add to wafer list", error in (no error)=w584) -> (queue out=w582:refnum<queue>, error out=w581:errorcluster)  [unwired: 1 in, 1 out]
          }
          event "Remove from wafer list": Value Change {
            # "removes highlighted value from wafer list"
            n223 = event-data() -> ()  [unwired: 1 in, 5 out]
            n224 = Enqueue Element(queue=w589, element="remove from wafer list", error in (no error)=w588) -> (queue out=w587:refnum<queue>, error out=w586:errorcluster)  [unwired: 1 in, 1 out]
          }
          event "Clear wafer list": Value Change {
            # "removes all values from wafer list"
            n225 = event-data() -> ()  [unwired: 1 in, 5 out]
            n226 = Enqueue Element(queue=w594, element="clear wafer list", error in (no error)=w593) -> (queue out=w592:refnum<queue>, error out=w591:errorcluster)  [unwired: 1 in, 1 out]
          }
          event "Update viewer": Value Change {
            # "Updates the measurement log viewer from the csv file in case of manual changes to the log"
            n227 = event-data() -> ()  [unwired: 1 in, 5 out]
            n228 = Enqueue Element(queue=w600, element="update viewer", error in (no error)=w599) -> (queue out=w598:refnum<queue>, error out=w597:errorcluster)  [unwired: 1 in, 1 out]
          }
          event "Save Comment": Value Change {
            # "Saves the comment to the highlighted entry in the measurement log, and updates the viewer to match the csv file. I still havent gotten the measurement log to close automatically however"
            n229 = event-data() -> ()  [unwired: 1 in, 5 out]
            n230 = Enqueue Element(queue=w608, element="save comment", error in (no error)=w607) -> (queue out=w605:refnum<queue>, error out=w603:errorcluster)  [unwired: 1 in, 1 out]
            n231 = Enqueue Element(queue=w605, element="update viewer", error in (no error)=w603) -> (queue out=w604:refnum<queue>, error out=w602:errorcluster)  [unwired: 1 in, 1 out]
          }
          event "Explore Data": Value Change {
            n232 = event-data() -> ()  [unwired: 1 in, 5 out]
            n233 = Enqueue Element(queue=w612, element="explore data", error in (no error)=w611) -> (queue out=w610:refnum<queue>, error out=w609:errorcluster)  [unwired: 1 in, 1 out]
          }
        }
      }
      n234 = while {
        shift-right: [w621] -> _
        shift-left: w35 -> [w618]
        shift-right: [w620] -> _
        shift-left: w34 -> [w617]
        stop <- w623 stop-if-true
        n235 = local read "Laser Current (mA)"() -> (w615:dbl)
        n236 = Dequeue Element(queue=w618, error in (no error)=w617) -> (queue out=w616:refnum<queue>, element=w622:string, error out=w619:errorcluster)  [unwired: 1 in, 1 out]
        n237 = Greater Than 0?(x=w615) -> (x > 0?=w614:bool)
        n238 = case shown="\"make common recipe\"" w622 {
          tunnel: [_ TRUE _ _ _ _ _ _ _ _ _ _ _ _ _ _ _ _ _ _ _ _ _ _ _ _ _ _ _ _ _ _ _ _ _ _ _ _ _ _ _ _ _ _ _ _ _ _ _ _ _ _ _ _ _ _ _ _ _ _ _] -> w623
          tunnel: w619 -> [w625 w627 w631 w827 w871 w881 w891 w921 w944 w954 w985 w1200 w1206 w1258 w1264 w1273 w1285 w1291 w1303 w1339 w1382 w1419 w1651 w1653 w1688 w1696 w1706 w1711 w1762 w1774 w1785 w1807 w1829 w1831 w1836 w1842 w1848 w1858 w1863 w1866 w1870 w1885 w1903 w1918 w1928 w1930 w1938 w1943 w1948 w1951 w1954 w1973 w1987 w2011 w2015 w2046 w2322 w2327 w2330 w2332 w2337]
          tunnel: [w625 w627 w632 w827 w872 w878 w888 w924 w945 w957 w984 w1200 w1206 w1258 w1268 w1273 w1285 w1290 w1305 w1339 w1384 w1421 w1651 w1653 w1688 w1698 w1708 w1711 w1762 w1771 w1788 w1807 w1829 w1831 w1836 w1844 w1851 w1858 w1863 w1866 w1869 w1885 w1903 w1918 w1928 w1930 w1938 w1943 w1948 w1951 w1954 w1973 w1987 w2011 w2014 w2046 w2322 w2327 w2330 w2332 w2337] -> w620
          tunnel: w616 -> [w624 w626 w634 w828 w874 w880 w890 w922 w947 w959 w982 w1201 w1207 w1259 w1270 w1274 w1286 w1289 w1304 w1340 w1383 w1418 w1652 w1654 w1689 w1697 w1707 w1712 w1763 w1775 w1787 w1808 w1830 w1832 w1837 w1843 w1850 w1859 w1864 w1867 w1872 w1886 w1904 w1919 w1929 w1931 w1939 w1944 w1949 w1952 w1955 w1974 w1988 w2012 w2017 w2047 w2323 w2328 w2331 w2333 w2338]
          tunnel: [w624 w626 w633 w828 w873 w879 w889 w923 w946 w958 w983 w1201 w1207 w1259 w1269 w1274 w1286 w1288 w1306 w1340 w1385 w1420 w1652 w1654 w1689 w1699 w1709 w1712 w1763 w1776 w1789 w1808 w1830 w1832 w1837 w1845 w1852 w1859 w1864 w1867 w1871 w1886 w1904 w1919 w1929 w1931 w1939 w1944 w1949 w1952 w1955 w1974 w1988 w2012 w2016 w2047 w2323 w2328 w2331 w2333 w2338] -> w621
          tunnel: w614 -> [_ _ _ _ _ _ _ _ _ _ _ _ _ _ _ _ _ _ _ _ _ w1422 _ _ _ _ _ _ _ _ _ _ _ _ _ _ _ _ _ _ _ _ _ _ _ _ _ _ _ _ _ _ _ _ _ _ _ _ _ _ _]
          frame "False", Default {
          }
          frame "stop" {
            # "Ends the for loop that contains the event structure, effectively ending the program"
          }
          frame "start raw" {
            # "Raw Test:\n(If Raw Test Skipped is TRUE, the entire raw test is not run. This only happens as part of the auto or lot tests)\n1) Loads mask file and updates info\n2) Finds/Creates directory for new Raw test file and creates file\n3) Runs raw test and updates graph after every measurement is taken\n4) Resets the prober to 0 0"
            n239 = local read "Raw Test Skipped"() -> (w630:bool)
            n240 = Not(x=w630) -> (.not. x?=w629:bool)
            n241 = case shown="True" w629 {
              frame False {
              }
              frame True {
                n242 = flat-sequence {
                  tunnel: [w648] -> w638
                  tunnel: w638 -> [w684]
                  tunnel: [w684] -> w637
                  tunnel: [w677] -> w636
                  tunnel: w637 -> [w686]
                  tunnel: w636 -> [w685]
                  frame #0 {
                    n243 = local read "Wafer Name"() -> (w646:string)
                    n244 = local read "RawTest ID"() -> (w651:u32)
                    n245 = local read "Scribe"() -> (w645:string)
                    n246 = local read "Mask"() -> (w644:string)
                    n247 = local read "Lot"() -> (w643:string)
                    n248 = local write "Status"("Prepare raw test" ("Status")) -> ()
                    n249 = Bundle By Name(cluster="Wafer Info 2", "Wafer Name"=w646, "Scribe"=w645, "Mask"=w644, "Lot"=w643) -> (w647:T10)
                    n250 = local write "Tab Control"(T17."Raw Test" ("Tab Control")) -> ()
                    n251 = Increment(x=w651) -> (x+1=w650:u32)
                    n252 = call "Device Files v1.vi"("Rows"=1200, "Mask file path"="Mask File Raw") -> ("size(s)"=w648:i32, "Array of Cell Clusters"=→"Array of Cell Data Clusters":T6)  [unwired: 6 in, 2 out]
                    "Total Device" <- w648
                    n253 = local write "Wafer Info"(w647) -> ()
                    n254 = local write "RawTest ID"(w650) -> ()
                    n255 = Initialize Array(nan ("element"), w648) -> (w641:dbl[])
                    n256 = local write "V meas"(w641) -> ()
                    n257 = local write "I meas"(w641) -> ()
                    n258 = Bundle(w641, w641) -> (→"Selected Data":cluster{dbl[], dbl[]})  [unwired: 1 in]
                    "Progress" <- u8 0 ("Progress")
                  }
                  frame #1 {
                    n259 = local read "Array of Cell Data Clusters"() -> (w683:T13)
                    n260 = local read "RawData Save Path"() -> (w659:path)
                    n261 = local read "Lot"() -> (w665:string)
                    n262 = Build Path(base path=w659, name or relative path=w665) -> (appended path=w664:path)
                    n263 = Index Array(array=w683, index=0) -> (element=w681:T18)
                    n264 = call "CreateDirectory.vi"("Path to be created"=w664) -> ()  [unwired: 10 in, 1 out]
                    n265 = local read "Wafer Name"() -> (w663:string)
                    n266 = Unbundle By Name(w681) -> ("Cell Name"=w680:string)
                    n267 = Build Path(base path=w664, name or relative path=w663) -> (appended path=w662:path)
                    n268 = call "get RawTest filename.vi"("Device Name"=w680, "Wafer Name"=w663) -> ("current time"=w674:timestamp, "FileName"=w679:string)  [unwired: 8 in]
                    n269 = call "CreateDirectory.vi"("Path to be created"=w662) -> ()  [unwired: 10 in, 1 out]
                    n270 = local write "Test FileName"(w679) -> ()
                    n271 = local read "Laser Current (mA)"() -> (w668:dbl)
                    n272 = local read "V compliance"() -> (w669:dbl)
                    n273 = local read "I compliance"() -> (w672:dbl)
                    n274 = local read "J set A/cm2"() -> (w671:dbl)
                    n275 = local read "RawTest ID"() -> (w667:u32)
                    n276 = local read "Operator"() -> (w666:string)
                    n277 = local read "V set"() -> (w673:dbl)
                    n278 = local read "I set"() -> (w670:dbl)
                    n279 = Bundle By Name(cluster="Session Info 2", "V set"=w673, "I compliance"=w672, "J set"=w671, "I set"=w670, "V compliance"=w669, "Laser Power (mW)"=w668, "TestID"=w667, "Session Time"=w674, "Operator"=w666) -> (w675:T8)
                    n280 = Build Path(base path=w662, name or relative path="Raw Data") -> (appended path=w660:path)
                    "new raw data save path" <- w660
                    n281 = local write "Session Info"(w675) -> ()
                    n282 = call "CreateDirectory.vi"("Path to be created"=w660) -> ("Output"=w657:path)  [unwired: 10 in]
                    n283 = Build Path(base path=w657, name or relative path=w679) -> (appended path=w658:path)
                    "Raw Test Filename" <- w658
                    n284 = call "writeFile RawTestHead.vi"("Name Array"="Name Array", "Path"=w658) -> ("Path out"=w677:path)  [unwired: 9 in]
                    "RawData file" <- w677
                  }
                  frame #2 {
                    n285 = for {
                      N: w686 -> [w699]
                      tunnel: w685 -> [w687]
                      i -> [w688]
                      n286 = Divide(x=w688, y=w699) -> (x/y=w697:dbl)
                      n287 = flat-sequence {
                        tunnel: [w733] -> w708
                        tunnel: [w732] -> w707
                        tunnel: w688 -> [w726]
                        tunnel: [w728] -> w703
                        tunnel: [w727] -> w702
                        tunnel: [w710] -> w701
                        tunnel: [w709] -> w700
                        tunnel: w708 -> [w734]
                        tunnel: w707 -> [w742]
                        tunnel: [w741] -> w706
                        tunnel: [w740] -> w705
                        tunnel: w703 -> [w738]
                        tunnel: w702 -> [w737]
                        tunnel: w701 -> [w736]
                        tunnel: w700 -> [w735]
                        tunnel: w706 -> [w745]
                        tunnel: w705 -> [w744]
                        tunnel: [w747] -> w704
                        tunnel: w704 -> [w771]
                        tunnel: [w771] -> w690
                        tunnel: [w772] -> w689
                        tunnel: w690 -> [w804]
                        tunnel: w689 -> [w803]
                        tunnel: w688 -> [w810]
                        tunnel: w687 -> [w801]
                        frame #0 {
                          n288 = Increment(x=w726) -> (x+1=→"Current Device":i32)
                          n289 = local read "Array of Cell Data Clusters"() -> (w730:T13)
                          n290 = local read "Laser Current (mA)"() -> (w722:dbl)
                          n291 = Index Array(array=w730, index=w726) -> (element=w723:T18)
                          n292 = local read "Device Name"() -> (w713:string)
                          n293 = Unbundle By Name(w723) -> ("X-coord"=w710:dbl, "Y-coord"=w709:dbl, "Area"=w711:dbl, "Meas Area"=w712:dbl, "Cell Name"=w716:string)
                          n294 = call "get Area.vi"("Laser"=w722, "Cell Data Cluster"=w723) -> ("Area"=w720:dbl)  [unwired: 9 in]
                          n295 = local read "J set A/cm2"() -> (w718:dbl)
                          n296 = local write "ActiveArea_um2"(w711) -> ()
                          n297 = local write "MesaArea_um2"(w712) -> ()
                          n298 = local write "Device Name"(w716) -> ()
                          n299 = Divide(x=w720, y=100000000.0) -> (x/y=w719:dbl)
                          n300 = Bundle By Name(cluster="Die Info 2", "Device Name"=w713, "ActiveArea_um2"=w711, "MesaArea_um2"=w712, "x"=w710, "y"=w709) -> (w714:T9)
                          n301 = Multiply(x=w718, y=w719) -> (x*y=w717:dbl)
                          n302 = local read "Prober GPIB"() -> (w724:string)
                          n303 = local read "current y"() -> (w729:i32)
                          n304 = local read "current x"() -> (w731:i32)
                          n305 = local write "Die Info"(w714) -> ()
                          n306 = local write "I set"(w717) -> ()
                          n307 = Subtract(x=w709, y=w729) -> (x-y=w727:dbl)
                          n308 = Subtract(x=w710, y=w731) -> (x-y=w728:dbl)
                          n309 = call "EG2001 Move Z Down.vi"("GPIB Address"=w724) -> ("Error Out"=w732:errorcluster, "GPIB Address Out"=w733:string)  [unwired: 9 in]
                        }
                        frame #1 {
                          n310 = local write "current x"(w736) -> ()
                          n311 = local write "current y"(w735) -> ()
                          n312 = call "EG2001 Move Machine Step X-Y.vi"("Flip X Coordinates?"=FALSE, "Y"=w737, "Steps/Microns"=enum32{"Steps", "Microns"}."Microns", "X"=w738, "error in (no error)"=w742, "GPIB Address"=w734) -> ("Error Out"=w740:errorcluster, "GPIB Address Out"=w741:string)  [unwired: 4 in]
                        }
                        frame #2 {
                          n313 = call "EG2001 Move Z Up.vi"("error in (no error)"=w744, "GPIB Address"=w745) -> ()  [unwired: 10 out]
                        }
                        frame #3 {
                          n314 = local read "Keysight"() -> (w746:bool)
                          n315 = case shown="False" w746 {
                            tunnel: [w748 w769] -> w747
                            frame False {
                              n316 = local read "Channel Keysight"() -> (w758:dbl)
                              n317 = local read "Imeas Settings"() -> (w752:T12)
                              n318 = local read "I compliance"() -> (w756:dbl)
                              n319 = local read "Id delay ms"() -> (w754:dbl)
                              n320 = local read "Repeat Id"() -> (w755:u32)
                              n321 = local read "4-wire"() -> (w751:bool)
                              n322 = local read "NPLC"() -> (w757:dbl)
                              n323 = local read "V set"() -> (w753:dbl)
                              n324 = local read "Keysight SMU"() -> (w749:refnum<visa-resource-name>)
                              n325 = Bundle By Name(cluster=w752, "Channel"=w758, "Vset"=w753, "NPLC"=w757, "I compliance"=w756, "Repeat time"=w755, "Delay ms"=w754, "4-wire"=w751) -> (w750:T12)
                              n326 = call "Agilent B2900 Measure I at Vset.vi"("Imeas Settings"=w750, "VISA resource name"=w749) -> ("Avg I"=w748:dbl)  [unwired: 9 in]
                              n327 = local write "Imeas Settings"(w750) -> ()
                            }
                            frame True {
                              n328 = local read "Imeas Settings"() -> (w761:T12)
                              n329 = local read "I compliance"() -> (w765:dbl)
                              n330 = local read "Id delay ms"() -> (w763:dbl)
                              n331 = local read "Repeat Id"() -> (w764:u32)
                              n332 = local read "Channel"() -> (w767:enum32{"Channel A", "Channel B"})
                              n333 = local read "4-wire"() -> (w760:bool)
                              n334 = local read "NPLC"() -> (w766:dbl)
                              n335 = local read "V set"() -> (w762:dbl)
                              n336 = local read "Keithley SMU"() -> (w768:refnum<visa-resource-name>)
                              n337 = Bundle By Name(cluster=w761, "Channel"=w767, "Vset"=w762, "NPLC"=w766, "I compliance"=w765, "Repeat time"=w764, "Delay ms"=w763, "4-wire"=w760) -> (w759:T12)
                              n338 = local write "Imeas Settings"(w759) -> ()
                              n339 = call "K2602 setVmeasI.vi"("Settings"=w759, "SMU"=w768) -> ("Iavg"=w769:dbl)  [unwired: 6 in, 3 out]
                            }
                          }
                        }
                        frame #4 {
                          n340 = local read "Keysight"() -> (w770:bool)
                          n341 = case shown="False" w770 {
                            tunnel: [w773 w788] -> w772
                            frame False {
                              n342 = local read "Vmeas Settings"() -> (w783:T12)
                              n343 = local read "V compliance"() -> (w781:dbl)
                              n344 = local read "Vf delay ms"() -> (w779:dbl)
                              n345 = local read "Repeat Vf"() -> (w780:u32)
                              n346 = local read "Channel"() -> (w782:enum32{"Channel A", "Channel B"})
                              n347 = local read "4-wire"() -> (w776:bool)
                              n348 = local read "NPLC"() -> (w778:dbl)
                              n349 = local read "I set"() -> (w777:dbl)
                              n350 = local read "Keysight SMU"() -> (w774:refnum<visa-resource-name>)
                              n351 = Bundle By Name(cluster=w783, "Channel"=w782, "Vset"=w777, "NPLC"=w778, "I compliance"=w781, "Repeat time"=w780, "Delay ms"=w779, "4-wire"=w776) -> (w775:T12)
                              n352 = call "Agilent B2900 Measure V at Iset.vi"("Imeas Settings"=w775, "VISA resource name"=w774) -> ("Avg V"=w773:dbl)  [unwired: 9 in]
                              n353 = local write "Vmeas Settings"(w775) -> ()
                            }
                            frame True {
                              n354 = local read "Channel Keysight"() -> (w792:dbl)
                              n355 = local read "Vmeas Settings"() -> (w793:T12)
                              n356 = local read "V compliance"() -> (w791:dbl)
                              n357 = local read "Vf delay ms"() -> (w789:dbl)
                              n358 = local read "Repeat Vf"() -> (w790:u32)
                              n359 = local read "4-wire"() -> (w785:bool)
                              n360 = local read "NPLC"() -> (w787:dbl)
                              n361 = local read "I set"() -> (w786:dbl)
                              n362 = Bundle By Name(cluster=w793, "Channel"=w792, "Vset"=w786, "NPLC"=w787, "I compliance"=w791, "Repeat time"=w790, "Delay ms"=w789, "4-wire"=w785) -> (w784:T12)
                              n363 = local write "Vmeas Settings"(w784) -> ()
                              n364 = call "K2602 setImeasV.vi"("Settings"=w784) -> ("Vavg"=w788:dbl)  [unwired: 7 in, 3 out]
                            }
                          }
                        }
                        frame #5 {
                          n365 = local read "I meas"() -> (w812:dbl[])
                          n366 = local read "V meas"() -> (w811:dbl[])
                          n367 = Replace Array Subset(array=w812, new element=w804, index=w810) -> (w807:dbl[])
                          n368 = Get Date/Time In Seconds() -> (seconds since 1Jan1904=w802:timestamp)
                          n369 = local read "Session Info"() -> (w797:T8)
                          n370 = local read "Wafer Info"() -> (w799:T10)
                          n371 = local read "Die Info"() -> (w798:T9)
                          n372 = local write "I meas"(w807) -> ()
                          n373 = Bundle By Name(cluster="Test Results 2", "I meas"=w804, "V meas"=w803, "Time"=w802) -> (w800:T7)
                          n374 = Replace Array Subset(array=w811, new element=w803, index=w810) -> (w806:dbl[])
                          n375 = local read "Selected Data"() -> (w795:cluster{dbl[], dbl[]})
                          n376 = local write "V meas"(w806) -> ()
                          n377 = call <vilib>:"Histogram.vi"("X"=w806) -> ("Histogram Graph"=→"Vforward hist":T15)  [unwired: 7 in, 3 out]
                          n378 = Bundle("V meas"=w806, "I meas"=w807) -> (w796:cluster{"V meas":dbl[], "I meas":dbl[]})  [unwired: 1 in]
                          n379 = call "writeFile RawTestData.vi"("Test Results"=w800, "Session Info"=w797, "Die Info"=w798, "Wafer Info"=w799, "Path"=w801) -> ()  [unwired: 6 in, 1 out]
                          n380 = local write "Test Results"(w800) -> ()
                          n381 = call <vilib>:"Histogram.vi"("X"=w807) -> ("Histogram Graph"=→"Idark hist":T15)  [unwired: 7 in, 3 out]
                          n382 = Build Array(w796, w795) -> (→"Spec Plot":cluster{"V meas":dbl[], "I meas":dbl[]}[])
                        }
                      }
                      n383 = Increment(x=w688) -> (x+1=w691:i32)
                      n384 = Multiply(x=w697, y=100.0) -> (x*y=w695:dbl)
                      n385 = To Unsigned Byte Integer(number=w695) -> (unsigned 8bit integer=w698:u8)
                      n386 = Number To Decimal String(number=w691) -> (decimal integer string=w693:string)  [unwired: 1 in]
                      n387 = local write "Progress"(w698) -> ()
                      n388 = Concatenate Strings("Raw Test for die number:" ("string"), w693) -> (w694:string)
                      n389 = local write "Status"(w694) -> ()
                    }
                  }
                  frame #3 {
                    w817 = -1
                    n390 = local read "Prober GPIB"() -> (w824:string)
                    n391 = local read "RawTest ID"() -> (w814:u32)
                    n392 = local read "TestID file"() -> (w813:path)
                    n393 = local read "current y"() -> (w818:i32)
                    n394 = local read "current x"() -> (w819:i32)
                    n395 = Multiply(x=w817, y=w818) -> (x*y=w815:i32)
                    n396 = Multiply(x=w817, y=w819) -> (x*y=w816:i32)
                    n397 = call "writeFile TestID.vi"("TestID"=w814, "Path"=w813) -> ()  [unwired: 10 in]
                    n398 = call "EG2001 Move Z Down.vi"("GPIB Address"=w824) -> ("Error Out"=w823:errorcluster, "GPIB Address Out"=w822:string)  [unwired: 9 in]
                    n399 = call "EG2001 Move Machine Step X-Y.vi"("Flip X Coordinates?"=FALSE, "Y"=w815, "Steps/Microns"=enum32{"Steps", "Microns"}."Microns", "X"=w816, "error in (no error)"=w823, "GPIB Address"=w822) -> ()  [unwired: 4 in, 2 out]
                  }
                  frame #4 {
                    w825 = 0
                    n400 = local write "current y"(w825) -> ()
                    n401 = local write "current x"(w825) -> ()
                  }
                }
              }
            }
            n402 = Enqueue Element At Opposite End(queue=w634, element="idle", error in (no error)=w631) -> (queue out=w633:refnum<queue>, error out=w632:errorcluster)  [unwired: 1 in, 1 out]
          }
          frame "find best devices mask" {
            # "If raw test is skipped - this searches through the saving structure (see guide) by lot, wafer name, and device name to find previous raw test measurements. When the file is found, it updates the fine mask file. If no file is found, a dialogue box alets the user of that"
            n403 = local read "Raw Test Skipped"() -> (w826:bool)
            n404 = case shown="True" w826 {
              frame False {
              }
              frame True {
                w842 = path "C:/Users/Flash/Desktop/Data/Detector test data" ("path")
                n405 = List Folder(path=w842) -> (folder names=w841:string[])  [unwired: 3 in, 3 out]
                n406 = for {
                  tunnel: w841 -> [w851] mode=indexing
                  tunnel: [w850] -> w843
                  tunnel: [w849] -> w833
                  stop <- w849 stop-if-true
                  n407 = local read "Lot"() -> (w850:string)
                  n408 = Equal?(x=w851, y=w850) -> (x = y?=w849:bool)
                }
                n409 = Build Path(base path=w842, name or relative path=w843) -> (appended path=w838:path)
                n410 = List Folder(path=w838) -> (folder names=w840:string[])  [unwired: 3 in, 3 out]
                n411 = for {
                  tunnel: w840 -> [w848] mode=indexing
                  tunnel: [w847] -> w839
                  tunnel: [w846] -> w835
                  stop <- w846 stop-if-true
                  n412 = local read "Wafer Name"() -> (w847:string)
                  n413 = Equal?(x=w848, y=w847) -> (x = y?=w846:bool)
                }
                n414 = Build Path(base path=w838, name or relative path=w839) -> (appended path=w831:path)
                n415 = Build Path(base path=w831, name or relative path="Raw Data") -> (appended path=w830:path)
                n416 = List Folder(path=w830) -> (filenames=w837:string[])  [unwired: 3 in, 3 out]
                n417 = for {
                  tunnel: w837 -> [w862] mode=indexing
                  tunnel: [w862] -> w844
                  tunnel: [w855] -> w836
                  stop <- w855 stop-if-true
                  w861 = "" ("y")
                  n418 = local read "Device Name"() -> (w854:string)
                  n419 = local read "Wafer Name"() -> (w865:string)
                  n420 = Concatenate Strings(w854, "_" ("string")) -> (w852:string)
                  n421 = Match Pattern(string=w862, regular expression="mask") -> (after substring=w860:string)  [unwired: 1 in, 3 out]
                  n422 = Match Pattern(string=w862, regular expression=w852) -> (after substring=w866:string)  [unwired: 1 in, 3 out]
                  n423 = Match Pattern(string=w862, regular expression=w865) -> (after substring=w864:string)  [unwired: 1 in, 3 out]
                  n424 = Not Equal?(x=w866, y=w861) -> (x != y?=w867:bool)
                  n425 = Not Equal?(x=w861, y=w864) -> (x != y?=w858:bool)
                  n426 = Not Equal?(x=w861, y=w860) -> (x != y?=w859:bool)
                  n427 = And(x=w867, y=w858) -> (x .and. y?=w856:bool)
                  n428 = And(x=w858, y=w859) -> (x .and. y?=w857:bool)
                  n429 = And(x=w856, y=w857) -> (x .and. y?=w855:bool)
                }
                n430 = Or(x=w836, y=w835) -> (x .or. y?=w834:bool)
                n431 = Build Path(base path=w830, name or relative path=w844) -> (appended path=w845:path)
                n432 = Or(x=w834, y=w833) -> (x .or. y?=w832:bool)
                n433 = local write "Mask File Fine"(w845) -> ()
                n434 = case shown="False" w832 {
                  frame False {
                    n435 = local write "no file"(TRUE ("no file")) -> ()
                    n436 = One Button Dialog(message="There is no file from which to run the fine test") -> ()  [unwired: 1 in, 1 out]
                  }
                  frame True {
                  }
                }
              }
            }
          }
          frame "reset xy" {
            # "Pretty Obvious"
            n437 = local read "Prober GPIB"() -> (w870:string)
            n438 = Enqueue Element At Opposite End(queue=w874, element="idle", error in (no error)=w871) -> (queue out=w873:refnum<queue>, error out=w872:errorcluster)  [unwired: 1 in, 1 out]
            n439 = call "EG2001 Move First.vi"("GPIB Address"=w870) -> ()  [unwired: 9 in, 2 out]
            "current x" <- u32 0 ("current x")
            "current y" <- u32 0 ("current y")
          }
          frame "reset to 1st die" {
            # "Moves prober to first die"
            n440 = Enqueue Element At Opposite End(queue=w880, element="idle", error in (no error)=w881) -> (queue out=w879:refnum<queue>, error out=w878:errorcluster)  [unwired: 1 in, 1 out]
            n441 = local read "Array of Cell Data Clusters"() -> (w887:T13)
            n442 = Index Array(array=w887, index=0) -> (element=w885:T18)
            n443 = Unbundle By Name(w885) -> ("X-coord"=w884:dbl, "Y-coord"=w883:dbl)
            n444 = local write "current x"(w884) -> ()
            n445 = local write "current y"(w883) -> ()
          }
          frame "load file manual" {
            # "Update informaiton from mask file to relevant variables"
            n446 = Enqueue Element At Opposite End(queue=w890, element="idle", error in (no error)=w891) -> (queue out=w889:refnum<queue>, error out=w888:errorcluster)  [unwired: 1 in, 1 out]
            n447 = flat-sequence {
              tunnel: [w897] -> w893
              tunnel: w893 -> [w901]
              frame #0 {
                n448 = local write "Status"("Loading mask file" ("Status")) -> ()
                n449 = call "Device Files v1.vi"("Rows"=1200, "Mask file path"="Mask File Manual") -> ("Mask Name"=w898:string, "size(s)"=w897:i32, "Array of Cell Clusters"=w894:T6)  [unwired: 6 in, 1 out]
                n450 = local write "Mask"(w898) -> ()
                n451 = local write "Array of Cell Data Clusters"(w894) -> ()
              }
              frame #1 {
                n452 = for {
                  N: w901 -> [_]
                  tunnel: [w902] -> w900 mode=indexing
                  i -> [w903]
                  n453 = Number To Decimal String(number=w903) -> (decimal integer string=w902:string)  [unwired: 1 in]
                }
                n454 = property on="Die Number" class="Ring (strict)"("Strings []"=w900) -> ()  [unwired: 2 in, 2 out]
              }
              frame #2 {
                n455 = local read "Die Number"() -> (w910:u16)
                n456 = local read "Array of Cell Data Clusters"() -> (w911:T13)
                n457 = Index Array(array=w911, index=w910) -> (element=w909:T18)
                n458 = Unbundle By Name(w909) -> ("Cell Name"=w904:string, "X-coord"=w907:dbl, "Y-coord"=w908:dbl, "Area"=w906:dbl, "Meas Area"=w905:dbl)
                n459 = local write "Device Name"(w904) -> ()
                n460 = local write "x target"(w907) -> ()
                n461 = local write "y target"(w908) -> ()
                n462 = local write "ActiveArea_um2"(w906) -> ()
                n463 = local write "MesaArea_um2"(w905) -> ()
              }
              frame #3 {
                n464 = local read "J set A/cm2"() -> (w917:dbl)
                n465 = local read "Laser Current (mA)"() -> (w914:dbl)
                n466 = Equal To 0?(x=w914) -> (x = 0?=w913:bool)
                n467 = case shown="False" w913 {
                  tunnel: [w919 w920] -> w912
                  frame False {
                    n468 = local read "ActiveArea_um2"() -> (w919:dbl)
                  }
                  frame True {
                    n469 = local read "MesaArea_um2"() -> (w920:dbl)
                  }
                }
                n470 = Divide(x=w912, y=100000000.0) -> (x/y=w916:dbl)
                n471 = Multiply(x=w916, y=w917) -> (x*y=w918:dbl)
                n472 = local write "I set"(w918) -> ()
              }
            }
          }
          frame "Die number picked" {
            # "Update target x and y when a new die is picked in the manual test tab"
            n473 = Enqueue Element At Opposite End(queue=w922, element="idle", error in (no error)=w921) -> (queue out=w923:refnum<queue>, error out=w924:errorcluster)  [unwired: 1 in, 1 out]
            n474 = local write "Status"("Changing Die" ("Status")) -> ()
            n475 = flat-sequence {
              frame #0 {
                n476 = local read "Die Number"() -> (w933:u16)
                n477 = local read "Array of Cell Data Clusters"() -> (w934:T13)
                n478 = Index Array(array=w934, index=w933) -> (element=w932:T18)
                n479 = Unbundle By Name(w932) -> ("Cell Name"=w929:string, "X-coord"=w931:dbl, "Y-coord"=w930:dbl, "Area"=w928:dbl, "Meas Area"=w927:dbl)
                n480 = local write "Device Name"(w929) -> ()
                n481 = local write "x target"(w931) -> ()
                n482 = local write "y target"(w930) -> ()
                n483 = local write "ActiveArea_um2"(w928) -> ()
                n484 = local write "MesaArea_um2"(w927) -> ()
              }
              frame #1 {
                n485 = local read "J set A/cm2"() -> (w940:dbl)
                n486 = local read "Laser Current (mA)"() -> (w937:dbl)
                n487 = Equal To 0?(x=w937) -> (x = 0?=w936:bool)
                n488 = case shown="True" w936 {
                  tunnel: [w942 w943] -> w935
                  frame False {
                    n489 = local read "ActiveArea_um2"() -> (w942:dbl)
                  }
                  frame True {
                    n490 = local read "MesaArea_um2"() -> (w943:dbl)
                  }
                }
                n491 = Divide(x=w935, y=100000000.0) -> (x/y=w939:dbl)
                n492 = Multiply(x=w939, y=w940) -> (x*y=w941:dbl)
                n493 = local write "I set"(w941) -> ()
              }
            }
          }
          frame "Jset change" {
            # "Updates Current setpoint for a desired current density"
            n494 = local read "J set A/cm2"() -> (w950:dbl)
            n495 = Enqueue Element At Opposite End(queue=w947, element="idle", error in (no error)=w944) -> (queue out=w946:refnum<queue>, error out=w945:errorcluster)  [unwired: 1 in, 1 out]
            n496 = local read "ActiveArea_um2"() -> (w953:dbl)
            n497 = Divide(x=w953, y=100000000.0) -> (x/y=w951:dbl)
            n498 = Multiply(x=w951, y=w950) -> (x*y=w949:dbl)
            n499 = local write "I set"(w949) -> ()
          }
          frame "moveto" {
            # "Moves from current xy to target xy, and then changes current xy to match lcation"
            n500 = Enqueue Element At Opposite End(queue=w959, element="idle", error in (no error)=w954) -> (queue out=w958:refnum<queue>, error out=w957:errorcluster)  [unwired: 1 in, 1 out]
            n501 = flat-sequence {
              tunnel: [w964] -> w956
              tunnel: [w963] -> w955
              tunnel: w956 -> [w969]
              tunnel: w955 -> [w968]
              frame #0 {
                n502 = local read "Prober GPIB"() -> (w962:string)
                n503 = local write "Status"("Probe up" ("Status")) -> ()
                n504 = call "EG2001 Move Z Down.vi"("GPIB Address"=w962) -> ("Error Out"=w963:errorcluster, "GPIB Address Out"=w964:string)  [unwired: 9 in]
              }
              frame #1 {
                n505 = local read "current y"() -> (w972:i32)
                n506 = local read "current x"() -> (w974:i32)
                n507 = local read "y target"() -> (w973:i32)
                n508 = local read "x target"() -> (w975:i32)
                n509 = local write "Status"("Moving Probe" ("Status")) -> ()
                n510 = Subtract(x=w973, y=w972) -> (x-y=w970:i32)
                n511 = Subtract(x=w975, y=w974) -> (x-y=w971:i32)
                n512 = call "EG2001 Move Machine Step X-Y.vi"("Flip X Coordinates?"=FALSE, "Y"=w970, "Steps/Microns"=enum32{"Steps", "Microns"}."Microns", "X"=w971, "error in (no error)"=w968, "GPIB Address"=w969) -> ()  [unwired: 4 in, 2 out]
              }
              frame #2 {
                n513 = local read "y target"() -> (w977:i32)
                n514 = local read "x target"() -> (w978:i32)
                n515 = local write "Status"("Done" ("Status")) -> ()
                n516 = local write "current x"(w978) -> ()
                n517 = local write "current y"(w977) -> ()
              }
            }
          }
          frame "manual test" {
            # "Manual Test execution - first runs sweep VI, then measures the two points for the raw test. It doesn NOT save anywhere automatically, just displays results on the graph"
            n518 = Enqueue Element At Opposite End(queue=w982, element="idle", error in (no error)=w985) -> (queue out=w983:refnum<queue>, error out=w984:errorcluster)  [unwired: 1 in, 1 out]
            n519 = flat-sequence {
              tunnel: [w995] -> w993
              tunnel: [w994] -> w992
              tunnel: [w1002] -> w991
              tunnel: w993 -> [w1002]
              tunnel: [w1001] -> w990
              tunnel: w992 -> [w1001]
              tunnel: [w1026] -> w989
              tunnel: w991 -> [w1026]
              tunnel: [w1025] -> w988
              tunnel: w990 -> [w1025]
              tunnel: ["Measure 2 Point?"] -> w980
              tunnel: [w1057] -> w987
              tunnel: w989 -> [w1057]
              tunnel: [w1056] -> w986
              tunnel: w988 -> [w1056]
              tunnel: w980 -> [w1055]
              tunnel: [w1055] -> w979
              tunnel: w987 -> [w1093]
              tunnel: w986 -> [w1092]
              tunnel: w979 -> [w1086]
              frame #0 {
                n520 = local read "Prober GPIB"() -> (w996:string)
                n521 = call "EG2001 Move Z Up.vi"("GPIB Address"=w996) -> ("Error Out"=w994:errorcluster, "GPIB Address Out"=w995:string)  [unwired: 1 in, 8 out]
              }
              frame #1 {
                n522 = local read "Channel"() -> (w1011:enum32{"Channel A", "Channel B"})
                n523 = local read "I compliance sweep"() -> (w1006:dbl)
                n524 = local read "sweep delay ms"() -> (w1005:dbl)
                n525 = local read "Sweep Settings"() -> (w1012:T11)
                n526 = local write "Status"("Sweeping IV Curve") -> ()
                n527 = local read "V start"() -> (w1010:dbl)
                n528 = local read "points"() -> (w1008:u16)
                n529 = local read "V end"() -> (w1009:dbl)
                n530 = local read "NPLC"() -> (w1007:dbl)
                n531 = Bundle By Name(cluster=w1012, "Channel"=w1011, "Vstart"=w1010, "Vend"=w1009, "# of points"=w1008, "NPLC"=w1007, "I compliance"=w1006, "Delay ms"=w1005) -> (w997:T11)
                n532 = local read "Keysight"() -> (w998:bool)
                n533 = local write "Sweep Settings"(w997) -> ()
                n534 = local read "4-wire"() -> (w999:bool)
                n535 = case shown="False" w998 {
                  tunnel: w997 -> [w1018 w1023]
                  tunnel: [w1015 w1022] -> w1004
                  tunnel: [w1014 w1021] -> w1003
                  tunnel: w999 -> [w1017 w1019]
                  frame False {
                    n536 = local read "Keysight SMU"() -> (w1016:refnum<visa-resource-name>)
                    n537 = call "IVSweep (SubVI).vi"("SweepSettings"=w1018, "4 wire"=w1017, "VISA Refnum in"=w1016, "Sweep Direction (0: Up)"="Sweep Direction (Keysight)") -> ("V"=w1014:dbl[], "I"=w1015:dbl[])  [unwired: 2 out]
                  }
                  frame True {
                    n538 = local read "Keithley SMU"() -> (w1020:refnum<visa-resource-name>)
                    n539 = call "K2602 Vsweep.vi"("4-wire"=w1019, "Settings"=w1023, "SMU"=w1020) -> ("V"=w1021:dbl[], "I"=w1022:dbl[])  [unwired: 6 in, 1 out]
                  }
                }
                "Varray manual" <- w1003
                "Iarray manual" <- w1004
              }
              frame #2 {
                n540 = case shown="True" "Measure 2 Point?" {
                  frame False {
                    n541 = local read "Iarray manual"() -> (w1028:dbl[])
                    n542 = Array Max & Min(array=w1028) -> (min value=w1027:dbl)  [unwired: 3 out]
                    n543 = local write "Imeas manual"(w1027) -> ()
                  }
                  frame True {
                    n544 = local read "Keysight"() -> (w1029:bool)
                    n545 = case shown="False" w1029 {
                      tunnel: [w1031 w1053] -> w1030
                      frame False {
                        n546 = local read "Channel Keysight"() -> (w1034:dbl)
                        n547 = local read "Repeat Id"() -> (w1038:u32)
                        n548 = local read "Imeas Settings"() -> (w1042:T12)
                        n549 = local read "I compliance"() -> (w1039:dbl)
                        n550 = local read "Id delay ms"() -> (w1037:dbl)
                        n551 = local write "Status"("Measuring I @ Vset") -> ()
                        n552 = local read "4-wire"() -> (w1035:bool)
                        n553 = local read "NPLC"() -> (w1040:dbl)
                        n554 = local read "V set"() -> (w1041:dbl)
                        n555 = Bundle By Name(cluster=w1042, "Channel"=w1034, "Vset"=w1041, "NPLC"=w1040, "I compliance"=w1039, "Repeat time"=w1038, "Delay ms"=w1037, "4-wire"=w1035) -> (w1033:T12)
                        n556 = local read "Keysight SMU"() -> (w1032:refnum<visa-resource-name>)
                        n557 = local write "Imeas Settings"(w1033) -> ()
                        n558 = call "Agilent B2900 Measure I at Vset.vi"("Imeas Settings"=w1033, "VISA resource name"=w1032) -> ("Avg I"=w1031:dbl)  [unwired: 9 in]
                      }
                      frame True {
                        n559 = local read "Id delay ms"() -> (w1047:dbl)
                        n560 = local read "Repeat Id"() -> (w1048:u32)
                        n561 = local read "Channel"() -> (w1052:enum32{"Channel A", "Channel B"})
                        n562 = local read "Imeas Settings"() -> (w1054:T12)
                        n563 = local read "I compliance"() -> (w1049:dbl)
                        n564 = local read "4-wire"() -> (w1045:bool)
                        n565 = local write "Status"("Measuring I @ Vset") -> ()
                        n566 = local read "NPLC"() -> (w1050:dbl)
                        n567 = local read "V set"() -> (w1051:dbl)
                        n568 = Bundle By Name(cluster=w1054, "Channel"=w1052, "Vset"=w1051, "NPLC"=w1050, "I compliance"=w1049, "Repeat time"=w1048, "Delay ms"=w1047, "4-wire"=w1045) -> (w1044:T12)
                        n569 = local read "Keithley SMU"() -> (w1043:refnum<visa-resource-name>)
                        n570 = local write "Imeas Settings"(w1044) -> ()
                        n571 = call "K2602 setVmeasI.vi"("Settings"=w1044, "SMU"=w1043) -> ("Iavg"=w1053:dbl)  [unwired: 6 in, 3 out]
                      }
                    }
                    n572 = local write "Imeas manual"(w1030) -> ()
                  }
                }
              }
              frame #3 {
                n573 = case shown="True" w1055 {
                  frame False {
                    n574 = local read "Varray manual"() -> (w1058:dbl[])
                    n575 = Array Max & Min(array=w1058) -> (min value=w1059:dbl)  [unwired: 3 out]
                    n576 = local write "Vmeas manual"(w1059) -> ()
                  }
                  frame True {
                    n577 = local read "Keysight"() -> (w1060:bool)
                    n578 = case shown="False" w1060 {
                      tunnel: [w1062 w1075] -> w1061
                      frame False {
                        n579 = local read "Vf delay ms"() -> (w1067:dbl)
                        n580 = local read "Repeat Vf"() -> (w1068:u32)
                        n581 = local read "Channel"() -> (w1072:enum32{"Channel A", "Channel B"})
                        n582 = local read "Vmeas Settings"() -> (w1073:T12)
                        n583 = local read "V compliance"() -> (w1069:dbl)
                        n584 = local read "4-wire"() -> (w1065:bool)
                        n585 = local write "Status"("Measuring V @ Iset") -> ()
                        n586 = local read "NPLC"() -> (w1070:dbl)
                        n587 = local read "I set"() -> (w1071:dbl)
                        n588 = Bundle By Name(cluster=w1073, "Channel"=w1072, "Vset"=w1071, "NPLC"=w1070, "I compliance"=w1069, "Repeat time"=w1068, "Delay ms"=w1067, "4-wire"=w1065) -> (w1064:T12)
                        n589 = local read "Keysight SMU"() -> (w1063:refnum<visa-resource-name>)
                        n590 = local write "Vmeas Settings"(w1064) -> ()
                        n591 = call "Agilent B2900 Measure V at Iset.vi"("Imeas Settings"=w1064, "VISA resource name"=w1063) -> ("Avg V"=w1062:dbl)  [unwired: 9 in]
                      }
                      frame True {
                        n592 = local read "Vf delay ms"() -> (w1079:dbl)
                        n593 = local read "Repeat Vf"() -> (w1080:u32)
                        n594 = local read "Channel"() -> (w1084:enum32{"Channel A", "Channel B"})
                        n595 = local read "Vmeas Settings"() -> (w1085:T12)
                        n596 = local read "V compliance"() -> (w1081:dbl)
                        n597 = local read "4-wire"() -> (w1077:bool)
                        n598 = local write "Status"("Measuring V @ Iset") -> ()
                        n599 = local read "NPLC"() -> (w1082:dbl)
                        n600 = local read "I set"() -> (w1083:dbl)
                        n601 = Bundle By Name(cluster=w1085, "Channel"=w1084, "Vset"=w1083, "NPLC"=w1082, "I compliance"=w1081, "Repeat time"=w1080, "Delay ms"=w1079, "4-wire"=w1077) -> (w1076:T12)
                        n602 = local read "Keithley SMU"() -> (w1074:refnum<visa-resource-name>)
                        n603 = call "K2602 setImeasV.vi"("Settings"=w1076, "SMU"=w1074) -> ("Vavg"=w1075:dbl)  [unwired: 6 in, 3 out]
                        n604 = local write "Vmeas Settings"(w1076) -> ()
                      }
                    }
                    n605 = local write "Vmeas manual"(w1061) -> ()
                  }
                }
              }
              frame #4 {
                n606 = call "EG2001 Move Z Down.vi"("error in (no error)"=w1092, "GPIB Address"=w1093) -> ()  [unwired: 8 in, 2 out]
                n607 = local write "Status"("Done") -> ()
                n608 = case shown="True" w1086 {
                  tunnel: [w1098 w1113] -> w1091
                  tunnel: [w1096 w1112] -> w1088
                  tunnel: [w1097 w1111] -> w1087
                  frame False {
                    n609 = local read "Manual IV Plot settting"() -> (w1098:enum32{"Linear plot", "Log plot"})
                    n610 = local read "Vmeas manual"() -> (w1101:dbl)
                    n611 = local read "Varray manual"() -> (w1102:dbl[])
                    n612 = local read "Imeas manual"() -> (w1100:dbl)
                    n613 = local read "Iarray manual"() -> (w1095:dbl[])
                    n614 = local read "points"() -> (w1103:u16)
                    n615 = local read "V set"() -> (w1099:dbl)
                    n616 = Array Max & Min(array=w1095) -> (min value=w1094:dbl)  [unwired: 3 out]
                    n617 = call "get Plot.vi"("I set"=w1094, "Imeas"=w1100, "V set"=w1099, "Vmeas"=w1101, "Iarray"=w1095, "Varray"=w1102, "points"=w1103) -> ("logplot"=w1096:cluster{"Varray manual":dbl[], dbl[]}[], "Linearplot"=w1097:T19)  [unwired: 3 in]
                  }
                  frame True {
                    n618 = local read "Manual IV Plot settting"() -> (w1113:enum32{"Linear plot", "Log plot"})
                    n619 = local read "Vmeas manual"() -> (w1107:dbl)
                    n620 = local read "Varray manual"() -> (w1109:dbl[])
                    n621 = local read "Imeas manual"() -> (w1106:dbl)
                    n622 = local read "Iarray manual"() -> (w1108:dbl[])
                    n623 = local read "points"() -> (w1110:u16)
                    n624 = local read "V set"() -> (w1105:dbl)
                    n625 = local read "I set"() -> (w1104:dbl)
                    n626 = call "get Plot.vi"("I set"=w1104, "Imeas"=w1106, "V set"=w1105, "Vmeas"=w1107, "Iarray"=w1108, "Varray"=w1109, "points"=w1110) -> ("logplot"=w1112:cluster{"Varray manual":dbl[], dbl[]}[], "Linearplot"=w1111:T19)  [unwired: 3 in]
                  }
                }
                "Manual Plot 0" <- w1087
                "Manaul Plot 1" <- w1088
                n627 = case shown="\"Linear plot\", Default" w1091 {
                  tunnel: w1087 -> [w1116 _]
                  tunnel: [w1116 w1119] -> w1090
                  tunnel: w1088 -> [_ w1119]
                  frame "Linear plot", Default {
                    n628 = property on="Manual IV" class="XYGraph (strict)"("YScale.Mapping Mode"=u8 0 ("Y Scale.Mapping Mode")) -> ()  [unwired: 2 in, 2 out]
                    n629 = property on="Manual IV" class="XYGraph (strict)"("YScale.NameLbl.Text"="Current (A)" ("X Scale.Name Label.Text")) -> ()  [unwired: 2 in, 2 out]
                  }
                  frame "Log plot" {
                    n630 = property on="Manual IV" class="XYGraph (strict)"("YScale.NameLbl.Text"="Abs(I)" ("Y Scale.Name Label.Text")) -> ()  [unwired: 2 in, 2 out]
                    n631 = property on="Manual IV" class="XYGraph (strict)"("YScale.Mapping Mode"=u8 1 ("Y Scale.Mapping Mode")) -> ()  [unwired: 2 in, 2 out]
                  }
                }
                "Manual IV" <- w1090
              }
              frame #5 {
                n632 = Two Button Dialog(message="Save Data?", 1:"Nay" ("F button name (\"Cancel\")"), 2:"Yea" ("T button name (\"OK\")")) -> (T button?=w1123:bool)
                n633 = case shown="True" w1123 {
                  frame False {
                  }
                  frame True {
                    n634 = flat-sequence {
                      tunnel: [w1129] -> w1125
                      tunnel: w1125 -> [w1152]
                      tunnel: [w1152] -> w1124
                      tunnel: w1124 -> [w1170]
                      frame #0 {
                        n635 = local read "Wafer Info 3"() -> (w1128:T3)
                        n636 = Bundle By Name(cluster=w1128, "Comment"="Manual Test Comments") -> (w1127:T3)
                        n637 = local write "Wafer Info 3"(w1127) -> ()
                      }
                      frame #1 {
                        n638 = local read "FineTest save path"() -> (w1136:path)
                        n639 = local read "Lot"() -> (w1137:string)
                        n640 = Build Path(base path=w1136, name or relative path=w1137) -> (appended path=w1138:path)
                        n641 = local read "Wafer Name"() -> (w1139:string)
                        n642 = call "CreateDirectory.vi"("Path to be created"=w1138) -> ()  [unwired: 10 in, 1 out]
                        n643 = Build Path(base path=w1138, name or relative path=w1139) -> (appended path=w1140:path)
                        n644 = local read "Output Power (mW)"() -> (w1131:dbl)
                        n645 = call "CreateDirectory.vi"("Path to be created"=w1140) -> ()  [unwired: 10 in, 1 out]
                        n646 = local read "Device Name"() -> (w1130:string)
                        n647 = Build Path(base path=w1140, name or relative path="IV") -> (appended path=w1142:path)
                        n648 = call "CreateDirectory.vi"("Path to be created"=w1142) -> ()  [unwired: 10 in, 1 out]
                        n649 = Number To Decimal String(number=w1131) -> (decimal integer string=w1133:string)  [unwired: 1 in]
                        n650 = Build Path(base path=w1142, name or relative path=w1130) -> (appended path=w1132:path)
                        n651 = call "CreateDirectory.vi"("Path to be created"=w1132) -> ()  [unwired: 10 in, 1 out]
                        n652 = Concatenate Strings(w1133, " mW" ("string")) -> (w1135:string)
                        n653 = Build Path(base path=w1132, name or relative path=w1135) -> (appended path=w1129:path)
                        n654 = call "CreateDirectory.vi"("Path to be created"=w1129) -> ()  [unwired: 10 in, 1 out]
                      }
                      frame #2 {
                        n655 = local read "I compliance sweep"() -> (w1147:dbl)
                        n656 = local read "sweep delay ms"() -> (w1146:dbl)
                        n657 = local read "Sweep Direction (Keysight)"() -> (w1151:i32)
                        n658 = local read "points"() -> (w1148:u16)
                        n659 = local read "V end"() -> (w1149:dbl)
                        n660 = local read "V start"() -> (w1150:dbl)
                        n661 = call "pho_DBCheck_LIV_meas_recipe.vi"("V start"=w1150, "Sweep Direction (Keysight)"=w1151, "V end"=w1149, "points"=w1148, "I compliance sweep"=w1147, "sweep delay ms"=w1146) -> ("RecipeID"=w1145:string)  [unwired: 8 in, 1 out]
                        n662 = local write "RecipeID"(w1145) -> ()
                        n663 = Equal?(x=w1145, y="") -> (x = y?=w1143:bool)
                        n664 = case shown="True" w1143 {
                          frame False {
                          }
                          frame True {
                            n665 = local read "I compliance sweep"() -> (w1155:dbl)
                            n666 = local read "sweep delay ms"() -> (w1154:dbl)
                            n667 = local read "Sweep Direction (Keysight)"() -> (w1159:i32)
                            n668 = local read "points"() -> (w1156:u16)
                            n669 = local read "V end"() -> (w1157:dbl)
                            n670 = local read "V start"() -> (w1158:dbl)
                            n671 = call "pho_DB_Insert_LIV_meas_recipe.vi"("V start"=w1158, "Sweep Direction (Keysight)"=w1159, "V end"=w1157, "points"=w1156, "I compliance sweep"=w1155, "sweep delay ms"=w1154) -> ("RecipeID"=w1153:string)  [unwired: 9 in]
                            n672 = local write "RecipeID"(w1153) -> ()
                          }
                        }
                      }
                      frame #3 {
                        n673 = local read "current y"() -> (w1176:i32)
                        n674 = local read "current x"() -> (w1175:i32)
                        n675 = local read "Current Session"() -> (w1160:timestamp)
                        n676 = local read "Temp Data"() -> (w1164:T2)
                        n677 = local read "Device Name"() -> (w1172:string)
                        n678 = local read "Wafer Name"() -> (w1171:string)
                        n679 = local read "Varray manual"() -> (w1178:dbl[])
                        n680 = local read "Iarray manual"() -> (w1177:dbl[])
                        n681 = local read "Operator"() -> (w1161:string)
                        n682 = To Double Precision Float(number=w1175) -> (double precision float=w1173:dbl)
                        n683 = To Double Precision Float(number=w1176) -> (double precision float=w1174:dbl)
                        n684 = Get Date/Time In Seconds() -> (seconds since 1Jan1904=w1183:timestamp)
                        n685 = local read "Parameters Flash"() -> (w1166:T5)
                        n686 = local read "RecipeID"() -> (w1165:string)
                        n687 = local read "Wafer Info 3"() -> (w1163:T3)
                        n688 = call "get Flash FileName .vi"("Time"=w1183, "Device Name"=w1172, "Operator"=w1161, "Wafer Name"=w1171, "FineTest save path"=w1170) -> ("appended path"=w1167:path)  [unwired: 6 in]
                        n689 = Build Array(w1178, w1177) -> (w1169:dbl[][])
                        n690 = Bundle(w1173, w1174) -> (w1162:cluster{dbl, dbl})  [unwired: 1 in]
                        n691 = Get Date/Time String(seconds (now)=w1183, want seconds? (F)=TRUE) -> (date string=w1179:string, time string=w1181:string)  [unwired: 1 in]
                        n692 = local read "Mask"() -> (w1168:string)
                        n693 = call <vilib>:"Space Constant.vi"() -> ("String"=w1182:string)
                        n694 = Concatenate Strings(w1179, w1182, w1181) -> ()  [unwired: 1 out]
                        n695 = call "WriteFlashFile NEW.vi"("Input File Path"=w1167, "IV array"=w1169, "Current Session"=w1160, "Parameters"=w1166, "RecipeID"=w1165, "User"=w1161, "Coords"=w1162, "Wafer Info"=w1163, "Mask Name"=w1168, "Temp Data"=w1164) -> ()  [unwired: 17 in, 1 out]
                      }
                    }
                  }
                }
              }
            }
          }
          frame "select preset sweep recipe" {
            n696 = call "getDB Detector Common Recipes.vi"() -> ("Desired ID"=w1199:string)  [unwired: 11 in]
            n697 = call "getDB Recipe from ID.vi"("ID"=w1199) -> ("OutputDetector Measurement Recipe"=w1198:T20)  [unwired: 10 in]
            n698 = Unbundle By Name(w1198) -> ("Start Voltage"=w1196:dbl, "End Voltage"=w1195:dbl, "# Data Points"=w1194:dbl, "I compliance"=w1193:dbl, "Sweep Delay"=w1192:dbl, "Direction"=w1189:string, "Recipe ID"=w1185:dbl)
            n699 = Number To Decimal String(number=w1185) -> (decimal integer string=w1184:string)  [unwired: 1 in]
            n700 = Multiply(x=w1192, y=1000.0) -> (x*y=w1190:dbl)
            n701 = Equal?(x=w1189, y="UP") -> (x = y?=w1187:bool)
            n702 = local read "Sweep Settings"() -> (w1197:T11)
            n703 = Bundle By Name(cluster=w1197, "Vstart"=w1196, "Vend"=w1195, "# of points"=w1194, "I compliance"=w1193, "Delay ms"=w1190) -> (w1186:T11)
            n704 = local write "RecipeID"(w1184) -> ()
            n705 = case shown="False" w1187 {
              frame False {
                w1202 = 1 items=["Up", "Down"] ("Sweep Direction (Keysight)")
                n706 = local write "Sweep Direction (Keysight)"(w1202) -> ()
              }
              frame True {
                w1203 = 0 items=["Up", "Down"] ("Sweep Direction (Keysight)")
                n707 = local write "Sweep Direction (Keysight)"(w1203) -> ()
              }
            }
            n708 = local write "Sweep Settings"(w1186) -> ()
          }
          frame "make common recipe" {
            n709 = call "New Common Recipe"() -> ("Comments"=w1204:string, "OK"=w1205:bool)  [unwired: 17 in, 1 out]
            n710 = case shown="True" w1205 {
              tunnel: w1204 -> [_ w1209]
              frame False {
              }
              frame True {
                n711 = flat-sequence {
                  tunnel: w1209 -> [w1210]
                  tunnel: [w1228] -> w1208
                  tunnel: w1208 -> [w1240]
                  frame #0 {
                    n712 = local read "Sweep Direction (Keysight)"() -> (w1216:i32)
                    n713 = local read "Sweep Settings"() -> (w1224:T11)
                    n714 = Equal?(x=w1216, y=0) -> (x = y?=w1213:bool)
                    n715 = Unbundle By Name(w1224) -> ("Vstart"=w1223:dbl, "Vend"=w1222:dbl, "# of points"=w1221:u16, "Delay ms"=w1220:dbl, "I compliance"=w1217:dbl)
                    n716 = case shown="False" w1213 {
                      tunnel: ["DOWN" "UP"] -> w1214
                      frame False {
                      }
                      frame True {
                      }
                    }
                    n717 = Divide(x=w1220, y=1000.0) -> (x/y=w1218:dbl)
                    n718 = local read "Detector Measurement Recipe"() -> (w1225:T1)
                    n719 = Bundle By Name(cluster=w1225, "Start Voltage"=w1223, "End Voltage"=w1222, "Number of Points"=w1221, "I compliance ma"=w1217, "Sweep Delay s"=w1218, "Direction"=w1214, "Comments"=w1210, "Common Recipe"=1.0) -> (w1211:T1)
                    n720 = local write "Detector Measurement Recipe"(w1211) -> ()
                  }
                  frame #1 {
                    n721 = local read "Detector Measurement Recipe"() -> (w1239:T1)
                    n722 = Unbundle By Name(w1239) -> ("Start Voltage"=w1238:dbl, "End Voltage"=w1237:dbl, "Number of Points"=w1236:dbl, "I compliance ma"=w1235:dbl, "Sweep Delay s"=w1234:dbl, "Direction"=w1233:string)
                    n723 = Bundle("Start Voltage"=w1238, "End Voltage"=w1237, "Number of Points"=w1236, "I compliance ma"=w1235, "Sweep Delay s"=w1234, "Direction"=w1233) -> (w1232:T21)  [unwired: 1 in]
                    n724 = call "Check Detector Recipe from phoDB.vi"("Input Detector Measurement Recipe"=w1232) -> ("OutputDetector Measurement Recipe"=w1231:T20)  [unwired: 10 in]
                    n725 = Unbundle By Name(w1231) -> ("Common Recipe"=w1230:dbl)
                    n726 = Equal?(x=w1230, y=1.0) -> (x = y?=w1228:bool)
                  }
                  frame #2 {
                    n727 = case shown="True" w1240 {
                      frame False {
                        n728 = local read "Detector Measurement Recipe"() -> (w1252:T1)
                        n729 = Unbundle By Name(w1252) -> ("Start Voltage"=w1251:dbl, "End Voltage"=w1250:dbl, "Number of Points"=w1249:dbl, "I compliance ma"=w1248:dbl, "Sweep Delay s"=w1247:dbl, "Direction"=w1246:string, "Comments"=w1245:string, "Common Recipe"=w1244:dbl, "Test Setup"=w1243:dbl)
                        n730 = Bundle("Start Voltage"=w1251, "End Voltage"=w1250, "Number of Points"=w1249, "I compliance ma"=w1248, "Sweep Delay s"=w1247, "Direction"=w1246, "Comments"=w1245, "Common Recipe"=w1244, "Test Setup"=w1243) -> (w1242:T22)  [unwired: 1 in]
                        n731 = call "Insert New Detector LIV Recipe into db.vi"("Recipe Input"=w1242) -> ("New Measurement ID"=w1241:string)  [unwired: 10 in]
                        n732 = local write "RecipeID"(w1241) -> ()
                      }
                      frame True {
                        n733 = One Button Dialog(message="This is already a common recipe", button name ("OK")="whoops...") -> ()  [unwired: 1 out]
                      }
                    }
                  }
                }
              }
            }
          }
          frame "generate prelim report" {
            n734 = call <vilib>:"System Exec.vi"("wait until completion? (T)"=FALSE, "working directory"=path "C:/Users/Flash/Documents/GitHub/solarjunction", "command line"="C:\\Windows\\system32\\cmd.exe /k python3 generate_prelim_report.py") -> ()  [unwired: 5 in, 4 out]
          }
          frame "update wafer" {
            # "Takes wafer name and pulls info from the database, and updates relevant variables"
            n735 = local read "Wafer Name"() -> (w1262:string)
            n736 = Enqueue Element At Opposite End(queue=w1270, element="idle", error in (no error)=w1264) -> (queue out=w1269:refnum<queue>, error out=w1268:errorcluster)  [unwired: 1 in, 1 out]
            n737 = call "getDB Wafer Info.vi"("Wafer Name"=w1262) -> ("WaferInfo"=w1263:T23)  [unwired: 9 in, 1 out]
            n738 = Unbundle By Name(w1263) -> ("WaferName"=w1260:string, "Scribe"=w1267:string, "Lot"=w1266:string, "Mask"=w1265:string)  [unwired: 1 out]
            n739 = local write "Scribe"(w1267) -> ()
            n740 = local write "Lot"(w1266) -> ()
            n741 = local write "Mask"(w1265) -> ()
            n742 = Equal?(x=w1262, y=w1260) -> (x = y?=w1261:bool)
            n743 = case shown="True" w1261 {
              tunnel: w1260 -> [w1272 _]
              frame False {
                n744 = local write "Wafer Name"(w1272) -> ()
              }
              frame True {
              }
            }
          }
          frame "desired wafer to current wafer" {
            # "This only runs in the lot test. It updates the wafer name from the wafer list. The Wafer counter keeps track of the iteration of the auto test the lot test is currently on. Once the wafer name is updated, the Wafer counter in incremented by one. If the Wafer list has reached its end, the wafer counter is returned to 0"
            n745 = flat-sequence {
              frame #0 {
                n746 = local read "WaferCounter"() -> (w1277:i32)
                n747 = property on="Wafer List" class="LstBox (strict)"() -> ("Item Names"=w1276:string[])  [unwired: 2 in, 2 out]
                n748 = Index Array(array=w1276, index=w1277) -> (element=w1275:string)
                n749 = local write "Wafer Name"(w1275) -> ()
              }
              frame #1 {
                n750 = local read "WaferCounter"() -> (w1279:i32)
                n751 = Increment(x=w1279) -> (x+1=w1278:i32)
                n752 = local write "WaferCounter"(w1278) -> ()
              }
              frame #2 {
                n753 = property on="Wafer List" class="LstBox (strict)"() -> ("Item Names"=w1283:string[])  [unwired: 2 in, 2 out]
                n754 = local read "WaferCounter"() -> (w1281:i32)
                n755 = Array Size(array=w1283) -> (size(s)=w1282:i32)
                n756 = Equal?(x=w1282, y=w1281) -> (x = y?=w1280:bool)
                n757 = case shown="True" w1280 {
                  frame False {
                  }
                  frame True {
                    n758 = local write "WaferCounter"(0 ("WaferCounter")) -> ()
                  }
                }
              }
            }
          }
          frame "idle" {
            n759 = local write "Status"("idle" ("Status")) -> ()
          }
          frame "change plot" {
            # "Switch from linear to logarithmic plot and back on the maual test tab"
            n760 = local read "Manual IV Plot settting"() -> (w1294:enum32{"Linear plot", "Log plot"})
            n761 = Enqueue Element At Opposite End(queue=w1289, element="idle", error in (no error)=w1291) -> (queue out=w1288:refnum<queue>, error out=w1290:errorcluster)  [unwired: 1 in, 1 out]
            n762 = case shown="\"Log plot\"" w1294 {
              tunnel: [w1297 w1300] -> w1293
              frame "Linear plot", Default {
                n763 = property on="Manual IV" class="XYGraph (strict)"("YScale.Mapping Mode"=u8 0 ("Y Scale.Mapping Mode")) -> ()  [unwired: 2 in, 2 out]
                n764 = local read "Manual Plot 0"() -> (w1297:cluster{"V manual":dbl[], "I manual":dbl[]}[])
                n765 = property on="Manual IV" class="XYGraph (strict)"("YScale.NameLbl.Text"="Current (A)" ("Y Scale.Name Label.Text")) -> ()  [unwired: 2 in, 2 out]
              }
              frame "Log plot" {
                n766 = property on="Manual IV" class="XYGraph (strict)"("YScale.Mapping Mode"=u8 1 ("Y Scale.Mapping Mode")) -> ()  [unwired: 2 in, 2 out]
                n767 = property on="Manual IV" class="XYGraph (strict)"("YScale.NameLbl.Text"="Abs(I)" ("Y Scale.Name Label.Text")) -> ()  [unwired: 2 in, 2 out]
                n768 = local read "Manaul Plot 1"() -> (w1300:cluster{"V manual":dbl[], dbl[]}[])
              }
            }
            n769 = local write "Manual IV"(w1293) -> ()
          }
          frame "select" {
            # "Selects Best ten devices (in seperate VI). If less than ten devices are within the voltage and current bounds, it selects all the devices that are within the parameters. If no devices are in the parameters, it still saves the mask file but it will be empty"
            n770 = Enqueue Element At Opposite End(queue=w1304, element="idle", error in (no error)=w1303) -> (queue out=w1306:refnum<queue>, error out=w1305:errorcluster)  [unwired: 1 in, 1 out]
            n771 = local read "Raw Test Skipped"() -> (w1302:bool)
            n772 = Not(x=w1302) -> (.not. x?=w1301:bool)
            n773 = case shown="True" w1301 {
              frame False {
              }
              frame True {
                n774 = local read "I meas"() -> (w1310:dbl[])
                n775 = Array Size(array=w1310) -> (size(s)=w1308:i32)
                n776 = Greater Than 0?(x=w1308) -> (x > 0?=w1309:bool)
                n777 = case shown="True" w1309 {
                  tunnel: w1308 -> [_ w1328]
                  frame False {
                  }
                  frame True {
                    n778 = local read "Laser Current (mA)"() -> (w1313:dbl)
                    n779 = local read "Number Select"() -> (w1334:u16)
                    n780 = local read "new raw data save path"() -> (w1330:path)
                    n781 = local read "V meas"() -> (w1320:dbl[])
                    n782 = local read "I meas"() -> (w1319:dbl[])
                    n783 = local read "Vmax"() -> (w1333:dbl)
                    n784 = local read "Vmin"() -> (w1332:dbl)
                    n785 = Greater Than 0?(x=w1313) -> (x > 0?=w1312:bool)
                    n786 = local read "Mask File Raw"() -> (w1335:path)
                    n787 = local read "RawData file"() -> (w1316:path)
                    n788 = local read "Wafer Name"() -> (w1336:string)
                    n789 = Initialize Array(nan ("element"), w1328) -> (w1324:dbl[])
                    n790 = call "select RawTestData.vi"("Light > 0?"=w1312, "Number Select"=w1334, "Vmax"=w1333, "Vmin"=w1332, "V meas"=w1320, "I meas"=w1319) -> ("Selected V"=w1327:dbl[], "Selected I"=w1325:dbl[], "Selected Index"=w1314:dbl[])  [unwired: 2 in, 1 out]
                    n791 = call "updatedFile RawTestSelect.vi"("Column Number"=u32 21, "Selected Index"=w1314, "Path"=w1316) -> ()  [unwired: 9 in]
                    n792 = Replace Array Subset(array=w1324, new element=w1327, index=0) -> (w1322:dbl[])
                    n793 = Replace Array Subset(array=w1324, new element=w1325, index=0) -> (w1321:dbl[])
                    n794 = call "save FineMask.vi"("Selected Index"=w1314, "RawData Save Path"=w1330, "Text Add"=w1336, "Mask File Raw"=w1335) -> ("Output path"=w1331:path)  [unwired: 7 in]
                    n795 = Bundle("V meas"=w1320, "I meas"=w1319) -> (w1318:cluster{"V meas":dbl[], "I meas":dbl[]})  [unwired: 1 in]
                    n796 = Bundle(w1322, w1321) -> (w1311:cluster{dbl[], dbl[]})  [unwired: 1 in]
                    n797 = local write "Mask File Fine"(w1331) -> ()
                    n798 = Build Array(w1318, w1311) -> (w1317:cluster{"V meas":dbl[], "I meas":dbl[]}[])
                    n799 = local write "Spec Plot"(w1317) -> ()
                  }
                }
              }
            }
          }
          frame "update measurement log" {
            # "Collects measurement parameters (such a test type) and saves them to the measurement log CSV file."
            n800 = flat-sequence {
              tunnel: [w1348] -> w1338
              tunnel: w1338 -> [w1364]
              tunnel: [w1355] -> w1337
              tunnel: w1337 -> [w1376]
              frame #0 {
                n801 = Get Date/Time In Seconds() -> (seconds since 1Jan1904=w1350:timestamp)
                n802 = Get Date/Time String(seconds (now)=w1350) -> (date string=w1344:string, time string=w1349:string)  [unwired: 2 in]
                n803 = local read "Wafer Name"() -> (w1352:string)
                n804 = local read "Test Type"() -> (w1341:string)
                n805 = local read "Operator"() -> (w1351:string)
                n806 = Search and Replace String(replace all?=TRUE ("replace all? (F)"), input string=w1344, search string="/", replace string="_" ("replace string (\"\")")) -> (result string=w1343:string)  [unwired: 4 in, 3 out]
                n807 = Bundle("result string"=w1343, "time string"=w1349, "Wafer Name"=w1352, "Operator"=w1351, "Test description"="Test description", "Test Type"=w1341) -> (w1348:T16)  [unwired: 1 in]
                "Last Measurement" <- w1348
              }
              frame #1 {
                w1353 = ","
                n808 = Unbundle(w1364) -> ("result string"=w1360:string, "time string"=w1359:string, "Wafer Name"=w1358:string, "Operator"=w1357:string, "Test description"=w1356:string, "Test Type"=w1354:string)
                n809 = Concatenate Strings(w1360, w1353, w1359, w1353, w1358, w1353, w1357, w1353, w1356, w1353, w1354) -> (w1361:string)
                n810 = call <vilib>:"Check if File or Folder Exists.vi"("path"=path "C:/Users/Flash/Desktop/Data/Detector test data/MeasurementLog.csv") -> ("file or folder exists?"=w1362:bool, "dup path"=w1355:path)  [unwired: 1 in, 8 out]
                n811 = case shown="True" w1362 {
                  tunnel: w1355 -> [w1369 w1374]
                  tunnel: w1361 -> [w1366 w1371]
                  frame False {
                    n812 = Build Array(w1366) -> (w1365:string[])
                    n813 = call-poly <vilib>:"Write To Spreadsheet File.vi"("delimiter (\\t)"="," ("delimiter (\\t)"), "append to file? (new file:F)"=FALSE, "1D data"=w1365, "file path (dialog if empty)"=w1369) -> ()  [unwired: 4 in, 1 out]
                  }
                  frame True {
                    n814 = Build Array(w1371) -> (w1370:string[])
                    n815 = call-poly <vilib>:"Write To Spreadsheet File.vi"("delimiter (\\t)"="," ("delimiter (\\t)"), "append to file? (new file:F)"=TRUE, "1D data"=w1370, "file path (dialog if empty)"=w1374) -> ()  [unwired: 4 in, 1 out]
                  }
                }
              }
              frame #2 {
                n816 = call-poly <vilib>:"Read From Spreadsheet File.vi"("file path (dialog if empty)"=w1376) -> ("all rows"=w1375:string[][])  [unwired: 6 in, 4 out]
                n817 = property on="Logview" class="MCListbox (strict)"("ItemNames"=w1375) -> ()  [unwired: 2 in, 2 out]
              }
            }
          }
          frame "load raw data" {
            # "Prompts the user to pick a raw data file, and then displays that data on the graphical display  on the raw test tab"
            n818 = local read "RawData Save Path"() -> (w1377:path)
            n819 = Enqueue Element At Opposite End(queue=w1383, element="idle", error in (no error)=w1382) -> (queue out=w1385:refnum<queue>, error out=w1384:errorcluster)  [unwired: 1 in, 1 out]
            n820 = call "File Dialog"("start path"=w1377, "prompt"="Please pick a raw test data file", "pattern (all files)"="*.csv" ("pattern label")) -> ("selected path"=w1378:path, "cancelled"=w1381:bool)  [unwired: 9 in, 2 out]
            n821 = case shown="False" w1381 {
              tunnel: w1378 -> [_ w1388]
              frame True {
              }
              frame False {
                n822 = Strip Path(path=w1388) -> (name=w1389:string)  [unwired: 1 out]
                n823 = Strip Path(path=w1388) -> (stripped path=w1387:path)  [unwired: 1 out]
                n824 = local write "RawData file"(w1388) -> ()
                n825 = call "read Raw.vi"("Path"=w1388) -> ("Session Info"=w1407:T24, "Die Info"=w1416:T25, "Wafer Info"=w1415:T10, "V"=w1393:dbl[], "I"=w1392:dbl[])  [unwired: 6 in]
                n826 = local write "Test FileName"(w1389) -> ()
                n827 = local write "new raw data save path"(w1387) -> ()
                n828 = local write "I meas"(w1392) -> ()
                n829 = Unbundle By Name(w1407) -> ("V set"=w1406:dbl, "I compliance"=w1405:dbl, "J set"=w1404:dbl, "I set"=w1403:dbl, "V compliance"=w1402:dbl, "Laser Power (mW)"=w1400:dbl, "Operator"=w1401:string)
                n830 = local write "V meas"(w1393) -> ()
                n831 = Unbundle By Name(w1416) -> ("Device Name"=w1410:string, "ActiveArea_um2"=w1409:dbl, "MesaArea_um2"=w1408:dbl)
                n832 = Unbundle By Name(w1415) -> ("Wafer Name"=w1414:string, "Scribe"=w1413:string, "Mask"=w1412:string, "Lot"=w1411:string)
                n833 = Array Size(array=w1392) -> (size(s)=w1398:i32)
                n834 = call <vilib>:"Histogram.vi"("X"=w1393) -> ("Histogram Graph"=w1390:T15)  [unwired: 7 in, 3 out]
                n835 = call <vilib>:"Histogram.vi"("X"=w1392) -> ("Histogram Graph"=w1391:T15)  [unwired: 7 in, 3 out]
                n836 = local write "Scribe"(w1413) -> ()
                n837 = local write "Mask"(w1412) -> ()
                n838 = local write "Lot"(w1411) -> ()
                n839 = local write "Device Name"(w1410) -> ()
                n840 = local write "ActiveArea_um2"(w1409) -> ()
                n841 = local write "MesaArea_um2"(w1408) -> ()
                n842 = local write "V set"(w1406) -> ()
                n843 = local write "I set"(w1403) -> ()
                n844 = local write "Vforward hist"(w1390) -> ()
                n845 = local write "Idark hist"(w1391) -> ()
                n846 = Initialize Array(nan ("element"), w1398) -> (w1397:dbl[])
                n847 = local write "Wafer Name"(w1414) -> ()
                n848 = local write "I compliance"(w1405) -> ()
                n849 = local write "J set A/cm2"(w1404) -> ()
                n850 = local write "V compliance"(w1402) -> ()
                n851 = local write "Laser Current (mA)"(w1400) -> ()
                n852 = local write "Operator"(w1401) -> ()
                n853 = Bundle("V"=w1393, "I"=w1392) -> (w1396:cluster{"V":dbl[], "I":dbl[]})  [unwired: 1 in]
                n854 = Bundle(w1397, w1397) -> (w1395:cluster{dbl[], dbl[]})  [unwired: 1 in]
                n855 = local write "Selected Data"(w1395) -> ()
                n856 = Build Array(w1396, w1395) -> (w1394:cluster{"V":dbl[], "I":dbl[]}[])
                n857 = local write "Spec Plot"(w1394) -> ()
              }
            }
          }
          frame "start fine" {
            # "Executes Fine test. If \"no file\" is true, it means that raw test was skipped, but then no previous raw data was found to run the fine test. The fine test will be skipped in this case.\n1) Loads  the fine mask files and updates relevant parameters\n2) Passes the parameters to the data clusters. There are three data clusters due to different versions of the save flash file. It saves the wafer information, time and date, current power, temperature, and other assorted parameters. Many parameters are leftover from the solar cell testing program, and are consequently always left as 0.\n3)The sweep is run using the Keithley sweep sub VI\n4) The directory is found/created to save the IV file (see guide for saving structure)\n5) data is saved and prober is returned to 0  0"
            n858 = Enqueue Element At Opposite End(queue=w1418, element="idle", error in (no error)=w1419) -> (queue out=w1420:refnum<queue>, error out=w1421:errorcluster)  [unwired: 1 in, 1 out]
            n859 = flat-sequence {
              tunnel: w1422 -> [w1425]
              frame #0 {
                n860 = local read "no file"() -> (w1424:bool)
                n861 = Not(x=w1424) -> (.not. x?=w1423:bool)
                n862 = case shown="True" w1423 {
                  tunnel: w1425 -> [_ w1426]
                  frame False {
                  }
                  frame True {
                    n863 = flat-sequence {
                      tunnel: [w1432] -> w1427
                      tunnel: w1426 -> [w1430]
                      tunnel: w1427 -> [w1444]
                      frame #0 {
                        w1433 = u8 0 ("Progress 2")
                        n864 = local write "Progress 2"(w1433) -> ()
                        n865 = local read "points"() -> (w1435:u16)
                        n866 = case shown="True" w1430 {
                          tunnel: "Mask File Fine" -> [w1442 w1443]
                          tunnel: [w1442 w1443] -> w1428
                          frame False {
                          }
                          frame True {
                          }
                        }
                        n867 = Initialize Array(nan ("element"), w1435) -> (w1437:dbl[])
                        n868 = local write "Tab Control"(T17."Fine Test" ("Tab Control")) -> ()
                        n869 = local write "Mask File Fine"(w1428) -> ()
                        n870 = local write "Status"("prepare fine test" ("Status")) -> ()
                        n871 = Bundle(w1437, w1437) -> (w1436:cluster{dbl[], dbl[]})  [unwired: 1 in]
                        n872 = call "Device Files v1.vi"("Rows"=1200, "Mask file path"=w1428) -> ("size(s)"=w1432:i32, "Array of Cell Clusters"=→"Fine Cell Clusters":T6)  [unwired: 6 in, 2 out]
                        "Total Device" <- w1432
                        n873 = Initialize Array(w1436, w1432) -> (→"IV fine linear" →"IV fine log":cluster{dbl[], dbl[]}[])
                        "Current Device" <- w1433
                      }
                      frame #1 {
                        n874 = for {
                          N: w1444 -> [w1474]
                          i -> [w1475]
                          n875 = flat-sequence {
                            tunnel: w1475 -> [w1490]
                            tunnel: [w1498] -> w1469
                            tunnel: [w1497] -> w1468
                            tunnel: [w1494] -> w1467
                            tunnel: [w1493] -> w1466
                            tunnel: [w1492] -> w1465
                            tunnel: [w1491] -> w1464
                            tunnel: [w1490] -> w1456
                            tunnel: w1469 -> [w1513]
                            tunnel: w1468 -> [w1512]
                            tunnel: w1467 -> [w1510]
                            tunnel: w1466 -> [w1509]
                            tunnel: w1465 -> [w1508]
                            tunnel: w1464 -> [w1507]
                            tunnel: [w1506] -> w1463
                            tunnel: [w1505] -> w1462
                            tunnel: [w1504] -> w1457
                            tunnel: w1456 -> [w1504]
                            tunnel: w1463 -> [w1516]
                            tunnel: w1462 -> [w1515]
                            tunnel: [w1514] -> w1458
                            tunnel: w1457 -> [w1514]
                            tunnel: [w1528] -> w1452
                            tunnel: w1458 -> [w1528]
                            tunnel: w1452 -> [w1553]
                            tunnel: [w1553] -> w1451
                            tunnel: w1451 -> [w1568]
                            tunnel: [w1568] -> w1454
                            tunnel: [w1561] -> w1453
                            tunnel: w1454 -> [w1589]
                            tunnel: [w1580] -> w1450
                            tunnel: [w1574] -> w1449
                            tunnel: [w1573] -> w1448
                            tunnel: w1453 -> [w1572]
                            tunnel: [w1602] -> w1447
                            tunnel: [w1603] -> w1446
                            tunnel: [w1604] -> w1445
                            tunnel: w1448 -> [w1604]
                            tunnel: w1449 -> [w1603]
                            tunnel: w1450 -> [w1602]
                            tunnel: w1447 -> [w1629]
                            tunnel: w1446 -> [w1616]
                            tunnel: w1445 -> [w1623]
                            frame #0 {
                              n876 = local read "Fine Cell Clusters"() -> (w1503:T6)
                              n877 = local read "Output Power (mW)"() -> (w1480:dbl)
                              n878 = local read "ActiveArea_um2"() -> (w1482:dbl)
                              n879 = Index Array(array=w1503, index=w1490) -> (element=w1487:T26)
                              n880 = local read "Laser Current (mA)"() -> (w1486:dbl)
                              n881 = Divide(x=w1482, y=100000000.0) -> (x/y=w1477:dbl)
                              n882 = Unbundle By Name(w1487) -> ("Cell Name"=w1502:string, "X-coord"=w1492:dbl, "Y-coord"=w1491:dbl, "Area"=w1501:dbl, "Mesa Area"=w1500:dbl)
                              n883 = Multiply(x=w1480, y=0.001) -> (x*y=w1478:dbl)
                              n884 = local write "Device Name"(w1502) -> ()
                              n885 = local write "ActiveArea_um2"(w1501) -> ()
                              n886 = local write "MesaArea_um2"(w1500) -> ()
                              n887 = call "get Area.vi"("Laser"=w1486, "Cell Data Cluster"=w1487) -> ("Area"=w1488:dbl)  [unwired: 9 in]
                              n888 = Divide(x=w1478, y=w1477) -> (x/y=w1476:dbl)
                              n889 = local read "current y"() -> (w1495:i32)
                              n890 = local read "current x"() -> (w1496:i32)
                              n891 = local read "Output Power (mW)"() -> (w1483:dbl)
                              n892 = local read "Laser Current (mA)"() -> (w1484:dbl)
                              n893 = local read "Parameters Flash 2"() -> (w1489:T5)
                              n894 = Subtract(x=w1491, y=w1495) -> (x-y=w1493:dbl)
                              n895 = Subtract(x=w1492, y=w1496) -> (x-y=w1494:dbl)
                              n896 = Bundle By Name(cluster=w1489, "Cell Area (cm²)"=w1488, "Input Current (mA)"=w1484, "Power Density (W/cm^2)"=w1476, "Incident Power"=w1483) -> (w1485:T5)
                              n897 = local read "Prober GPIB"() -> (w1499:string)
                              n898 = local write "Parameters Flash"(w1485) -> ()
                              n899 = call "EG2001 Move Z Down.vi"("GPIB Address"=w1499) -> ("Error Out"=w1497:errorcluster, "GPIB Address Out"=w1498:string)  [unwired: 9 in]
                            }
                            frame #1 {
                              n900 = local write "current x"(w1508) -> ()
                              n901 = local write "current y"(w1507) -> ()
                              n902 = call "EG2001 Move Machine Step X-Y.vi"("Y"=w1509, "Steps/Microns"=enum32{"Steps", "Microns"}."Microns", "X"=w1510, "error in (no error)"=w1512, "GPIB Address"=w1513) -> ("Error Out"=w1505:errorcluster, "GPIB Address Out"=w1506:string)  [unwired: 5 in]
                            }
                            frame #2 {
                              n903 = call "EG2001 Move Z Up.vi"("error in (no error)"=w1515, "GPIB Address"=w1516) -> ()  [unwired: 10 out]
                            }
                            frame #3 {
                              n904 = local read "I compliance sweep"() -> (w1532:dbl)
                              n905 = local read "Wafer Info Flash 2"() -> (w1527:T4)
                              n906 = local read "sweep delay ms"() -> (w1531:dbl)
                              n907 = local read "Sweep Settings"() -> (w1538:T11)
                              n908 = local read "Temp Setpoint"() -> (w1523:string)
                              n909 = local read "Device Name"() -> (w1526:string)
                              n910 = local read "Channel"() -> (w1537:enum32{"Channel A", "Channel B"})
                              n911 = local read "V start"() -> (w1535:dbl)
                              n912 = local read "points"() -> (w1534:u16)
                              n913 = local read "V end"() -> (w1536:dbl)
                              n914 = local read "NPLC"() -> (w1533:dbl)
                              n915 = Bundle By Name(cluster=w1538, "Channel"=w1537, "Vstart"=w1535, "Vend"=w1536, "# of points"=w1534, "NPLC"=w1533, "I compliance"=w1532, "Delay ms"=w1531) -> (w1517:T11)
                              n916 = Bundle By Name(cluster=w1527, "Cell Name"=w1526) -> (w1525:T4)
                              n917 = Decimal String To Number(string=w1523) -> (number=w1520:i32)  [unwired: 2 in, 1 out]
                              n918 = local write "Wafer Info Flash"(w1525) -> ()
                              n919 = local write "Sweep Settings"(w1517) -> ()
                              n920 = call "DAQ Assistant"() -> ("data"=w1521:dynamicdata)  [unwired: 17 in, 2 out]
                              n921 = local read "Temp Data"() -> (w1524:T2)
                              n922 = local read "Keysight"() -> (w1519:bool)
                              n923 = local read "4-wire"() -> (w1518:bool)
                              n924 = Bundle By Name(cluster=w1524, "Ambient Temperature"=w1521, "Chuck Set Temperature"=w1520) -> (w1522:T2)
                              n925 = case shown="False" w1519 {
                                tunnel: w1517 -> [w1544 w1549]
                                tunnel: [w1541 w1548] -> w1530
                                tunnel: [w1542 w1547] -> w1529
                                tunnel: w1518 -> [w1543 w1546]
                                frame False {
                                n926 = local read "Sweep Direction (Keysight)"() -> (w1539:i32)
                                n927 = call "IVSweep (SubVI).vi"("SweepSettings"=w1544, "4 wire"=w1543, "VISA Refnum in"="Keysight SMU", "Sweep Direction (0: Up)"=w1539) -> ("V"=w1542:dbl[], "I"=w1541:dbl[])  [unwired: 2 out]
                                }
                                frame True {
                                n928 = local read "Keithley SMU"() -> (w1545:refnum<visa-resource-name>)
                                n929 = call "K2602 Vsweep.vi"("4-wire"=w1546, "Settings"=w1549, "SMU"=w1545) -> ("V"=w1547:dbl[], "I"=w1548:dbl[])  [unwired: 6 in, 1 out]
                                }
                              }
                              n930 = local write "Temp Data"(w1522) -> ()
                              n931 = local write "I fine"(w1530) -> ()
                              n932 = local write "V fine"(w1529) -> ()
                            }
                            frame #4 {
                              n933 = local read "Device Name"() -> (w1551:string)
                              n934 = local read "Wafer Info 3"() -> (w1552:T3)
                              n935 = Bundle By Name(cluster=w1552, "Cell Name (Automatic)"=w1551) -> (w1550:T3)
                              n936 = local write "Wafer Info 3"(w1550) -> ()
                            }
                            frame #5 {
                              n937 = local read "FineTest save path"() -> (w1560:path)
                              n938 = local read "Lot"() -> (w1559:string)
                              n939 = Build Path(base path=w1560, name or relative path=w1559) -> (appended path=w1558:path)
                              n940 = call "CreateDirectory.vi"("Path to be created"=w1558) -> ()  [unwired: 10 in, 1 out]
                              n941 = local read "Wafer Name"() -> (w1557:string)
                              n942 = Build Path(base path=w1558, name or relative path=w1557) -> (appended path=w1556:path)
                              n943 = call "CreateDirectory.vi"("Path to be created"=w1556) -> ()  [unwired: 10 in, 1 out]
                              n944 = Build Path(base path=w1556, name or relative path="IV") -> (appended path=w1554:path)
                              n945 = call "CreateDirectory.vi"("Path to be created"=w1554) -> ()  [unwired: 10 in, 1 out]
                              n946 = local read "Output Power (mW)"() -> (w1566:dbl)
                              n947 = local read "Device Name"() -> (w1567:string)
                              n948 = Build Path(base path=w1554, name or relative path=w1567) -> (appended path=w1565:path)
                              n949 = Number To Decimal String(number=w1566) -> (decimal integer string=w1564:string)  [unwired: 1 in]
                              n950 = call "CreateDirectory.vi"("Path to be created"=w1565) -> ()  [unwired: 10 in, 1 out]
                              n951 = Concatenate Strings(w1564, " mW" ("string")) -> (w1562:string)
                              n952 = Build Path(base path=w1565, name or relative path=w1562) -> (appended path=w1561:path)
                              n953 = call "CreateDirectory.vi"("Path to be created"=w1561) -> ()  [unwired: 10 in, 1 out]
                            }
                            frame #6 {
                              n954 = local read "Wafer Info 3"() -> (w1571:T3)
                              n955 = local read "Comments"() -> (w1570:string)
                              n956 = local read "V fine"() -> (w1579:dbl[])
                              n957 = local read "I fine"() -> (w1585:dbl[])
                              n958 = Bundle By Name(cluster=w1571, "Comment"=w1570) -> (w1569:T3)
                              n959 = Bundle("V fine"=w1579, "I fine"=w1585) -> (w1590:cluster{"V fine":dbl[], "I fine":dbl[]})  [unwired: 1 in]
                              n960 = Absolute Value(x=w1585) -> (abs(x)=w1586:dbl[])
                              n961 = local write "Wafer Info 3"(w1569) -> ()
                              n962 = local read "IV fine linear"() -> (w1592:cluster{dbl[], dbl[]}[])
                              n963 = Bundle("V fine"=w1579, w1586) -> (w1584:cluster{"V fine":dbl[], dbl[]})  [unwired: 1 in]
                              n964 = local read "IV fine log"() -> (w1587:cluster{dbl[], dbl[]}[])
                              n965 = local read "current x"() -> (w1576:i32)
                              n966 = local read "current y"() -> (w1575:i32)
                              n967 = Replace Array Subset(array=w1592, new element=w1590, index=w1589) -> (w1591:cluster{dbl[], dbl[]}[])
                              n968 = local read "Device Name"() -> (w1581:string)
                              n969 = local write "IV fine linear"(w1591) -> ()
                              n970 = local read "Wafer Name"() -> (w1583:string)
                              n971 = Replace Array Subset(array=w1587, new element=w1584, index=w1589) -> (w1588:cluster{dbl[], dbl[]}[])
                              n972 = local read "Operator"() -> (w1582:string)
                              n973 = To Double Precision Float(number=w1576) -> (double precision float=w1578:dbl)
                              n974 = To Double Precision Float(number=w1575) -> (double precision float=w1577:dbl)
                              n975 = Get Date/Time In Seconds() -> (seconds since 1Jan1904=w1573:timestamp)
                              n976 = local write "IV fine log"(w1588) -> ()
                              n977 = call "get Flash FileName .vi"("Time"=w1573, "Device Name"=w1581, "Operator"=w1582, "Wafer Name"=w1583, "FineTest save path"=w1572) -> ("appended path"=w1580:path)  [unwired: 6 in]
                              n978 = Bundle(w1578, w1577) -> (w1574:cluster{dbl, dbl})  [unwired: 1 in]
                            }
                            frame #7 {
                              n979 = local read "Sweep Direction (Keysight)"() -> (w1593:i32)
                              n980 = local read "I compliance sweep"() -> (w1597:dbl)
                              n981 = local read "sweep delay ms"() -> (w1598:dbl)
                              n982 = local read "V start"() -> (w1594:dbl)
                              n983 = local read "points"() -> (w1596:u16)
                              n984 = local read "V end"() -> (w1595:dbl)
                              n985 = call "pho_DBCheck_LIV_meas_recipe.vi"("V start"=w1594, "Sweep Direction (Keysight)"=w1593, "V end"=w1595, "points"=w1596, "I compliance sweep"=w1597, "sweep delay ms"=w1598) -> ("RecipeID"=w1599:string)  [unwired: 8 in, 1 out]
                              n986 = local write "RecipeID"(w1599) -> ()
                              n987 = Equal?(x=w1599, y="") -> (x = y?=w1601:bool)
                              n988 = case shown="True" w1601 {
                                frame False {
                                }
                                frame True {
                                n989 = local read "Sweep Direction (Keysight)"() -> (w1611:i32)
                                n990 = local read "I compliance sweep"() -> (w1607:dbl)
                                n991 = local read "sweep delay ms"() -> (w1606:dbl)
                                n992 = local read "V start"() -> (w1610:dbl)
                                n993 = local read "points"() -> (w1608:u16)
                                n994 = local read "V end"() -> (w1609:dbl)
                                n995 = call "pho_DB_Insert_LIV_meas_recipe.vi"("V start"=w1610, "Sweep Direction (Keysight)"=w1611, "V end"=w1609, "points"=w1608, "I compliance sweep"=w1607, "sweep delay ms"=w1606) -> ("RecipeID"=w1605:string)  [unwired: 9 in]
                                n996 = local write "RecipeID"(w1605) -> ()
                                }
                              }
                            }
                            frame #8 {
                              n997 = local read "V fine"() -> (w1626:dbl[])
                              n998 = local read "I fine"() -> (w1627:dbl[])
                              n999 = local read "Current Session"() -> (w1612:timestamp)
                              n1000 = Build Array(w1626, w1627) -> (w1625:dbl[][])
                              n1001 = Get Date/Time String(seconds (now)=w1623, want seconds? (F)=TRUE) -> (date string=w1622:string, time string=w1620:string)  [unwired: 1 in]
                              n1002 = local read "Parameters Flash"() -> (w1624:T5)
                              n1003 = local read "Temp Data"() -> (w1617:T2)
                              n1004 = local read "Operator"() -> (w1613:string)
                              n1005 = local read "RecipeID"() -> (w1614:string)
                              n1006 = local read "Mask"() -> (w1628:string)
                              n1007 = call <vilib>:"Space Constant.vi"() -> ("String"=w1619:string)
                              n1008 = Concatenate Strings(w1622, w1619, w1620) -> (w1618:string)
                              n1009 = call "WriteFlashFile NEW.vi"("Input File Path"=w1629, "IV array"=w1625, "Current Session"=w1612, "Parameters"=w1624, "RecipeID"=w1614, "User"=w1613, "Coords"=w1616, "Wafer Info"="Wafer Info 3", "Mask Name"=w1628, "Temp Data"=w1617, "Die Number"=w1618) -> ()  [unwired: 16 in, 1 out]
                            }
                          }
                          n1010 = Increment(x=w1475) -> (x+1=w1455:i32)
                          n1011 = Divide(x=w1455, y=w1474) -> (x/y=w1473:dbl)
                          n1012 = local write "Current Device"(w1455) -> ()
                          n1013 = Multiply(x=100.0, y=w1473) -> (x*y=w1471:dbl)
                          n1014 = Number To Decimal String(number=w1455) -> (decimal integer string=w1460:string)  [unwired: 1 in]
                          n1015 = To Unsigned Byte Integer(number=w1471) -> (unsigned 8bit integer=w1470:u8)
                          n1016 = Concatenate Strings("IV test for die number: " ("string"), w1460) -> (w1459:string)
                          n1017 = local write "Progress 2"(w1470) -> ()
                          n1018 = local write "Status"(w1459) -> ()
                        }
                      }
                      frame #2 {
                        w1634 = -1 ("x")
                        n1019 = local read "Prober GPIB"() -> (w1638:string)
                        n1020 = local read "current y"() -> (w1635:i32)
                        n1021 = local read "current x"() -> (w1636:i32)
                        n1022 = Multiply(x=w1635, y=w1634) -> (x*y=w1632:i32)
                        n1023 = Multiply(x=w1634, y=w1636) -> (x*y=w1633:i32)
                        n1024 = call "EG2001 Move Z Down.vi"("GPIB Address"=w1638) -> ("Error Out"=w1637:errorcluster, "GPIB Address Out"=w1639:string)  [unwired: 9 in]
                        n1025 = call "EG2001 Move Machine Step X-Y.vi"("Flip X Coordinates?"=FALSE, "Y"=w1632, "Steps/Microns"=enum32{"Steps", "Microns"}."Microns", "X"=w1633, "error in (no error)"=w1637, "GPIB Address"=w1639) -> ()  [unwired: 4 in, 2 out]
                      }
                      frame #3 {
                        w1640 = 0 ("current x")
                        n1026 = local write "current y"(w1640) -> ()
                        n1027 = local write "current x"(w1640) -> ()
                      }
                    }
                  }
                }
              }
              frame #1 {
                n1028 = local write "no file"(FALSE ("no file")) -> ()
              }
            }
          }
          frame "update temperature" {
            # "Temptronics is communicatied via VISA sreial commands. RS sets the temperature, and ST tells the TEC to set the current temperature on the output pins to be read"
            n1029 = local read "Temp Setpoint"() -> (w1649:string)
            n1030 = local read "Temptronics VISA"() -> (w1647:refnum<visa-resource-name>)
            n1031 = Concatenate Strings("rs" ("string"), w1649) -> (w1648:string)
            n1032 = VISA Write(VISA resource name=w1647, write buffer=w1648) -> (VISA resource name out=w1646:refnum<visa-resource-name>)  [unwired: 1 in, 2 out]
            n1033 = VISA Write(VISA resource name=w1646, write buffer="st") -> (VISA resource name out=w1644:refnum<visa-resource-name>, return count=w1643:u32)  [unwired: 1 in, 1 out]
            n1034 = VISA Read(VISA resource name=w1644, byte count=w1643) -> (read buffer=w1642:string)  [unwired: 1 in, 3 out]
            n1035 = local write "Current Temp"(w1642) -> ()
          }
          frame "Update Laser" {
            # "Sets the laser current to the values set in the Laser Current (mA) box. Then uses the calibration file to find the appropriate power and updates that. Finally updates the compliance for the sweeps so illuminated IV curves don't just hit compliance due to photogenerated current"
            n1036 = flat-sequence {
              frame #0 {
                n1037 = local read "TL4000 In"() -> (w1658:refnum<visa-resource-name>)
                n1038 = local read "Laser Current (mA)"() -> (w1655:dbl)
                n1039 = Divide(x=w1655, y=1000.0) -> (x/y=w1670:dbl)
                n1040 = call <instrlib>:"TL4000 Set Laser Diode Current Setpoint.vi"("Laser Diode Current Setpoint (0.0)"=w1670, "instrument handle"=w1658) -> ()  [unwired: 8 in, 2 out]
                n1041 = call-poly <vilib>:"Read From Spreadsheet File.vi"("delimiter (\\t)"="," ("delimiter (\\t)"), "file path (dialog if empty)"="Load Calibration File") -> ("all rows"=w1665:dbl[][])  [unwired: 5 in, 4 out]
                n1042 = Index Array(array=w1665, index (row)=0) -> (element=w1667:dbl[])  [unwired: 1 in]
                n1043 = Index Array(array=w1665, index (row)=1) -> (element=w1657:dbl[])  [unwired: 1 in]
                n1044 = Array Size(array=w1657) -> (size(s)=w1656:i32)
                n1045 = call "Convert to Dynamic Data2"("Array"=w1657) -> ("Dynamic Data Type"=w1669:dynamicdata)  [unwired: 3 in]
                n1046 = call "Convert to Dynamic Data"("Array"=w1667) -> ("Dynamic Data Type"=w1668:dynamicdata)  [unwired: 3 in]
                n1047 = for {
                  N: w1656 -> [_]
                  tunnel: w1667 -> [w1675] mode=indexing
                  tunnel: w1655 -> [w1676]
                  tunnel: w1657 -> [w1674]
                  tunnel: [w1672] -> w1662
                  i -> [w1673]
                  stop <- w1671 stop-if-true
                  n1048 = Equal?(x=w1675, y=w1676) -> (x = y?=w1671:bool)
                  n1049 = case shown="False" w1671 {
                    tunnel: w1674 -> [_ w1679]
                    tunnel: w1673 -> [_ w1678]
                    tunnel: [_ w1677] -> w1672
                    frame False {
                    }
                    frame True {
                      n1050 = Index Array(array=w1679, index=w1678) -> (element=w1677:dbl)
                    }
                  }
                }
                "Output Power (mW)" <- w1662
                n1051 = call "Build XY Graph"("Y Input"=w1669, "X Input"=w1668) -> ("XY Graph"=→"Calibration":cluster{"Y":dbl[], "Y":dbl[]}[])  [unwired: 3 in, 6 out]
              }
              frame #1 {
                n1052 = case shown="True" "Auto Adjust Compliance?" {
                  frame False {
                  }
                  frame True {
                    n1053 = local read "Output Power (mW)"() -> (w1683:dbl)
                    n1054 = Greater Or Equal?(x=w1683, y=0.1) -> (x >= y?=w1681:bool)
                    n1055 = case shown="False" w1681 {
                      frame False {
                        n1056 = local write "I compliance sweep"(0.001 ("I compliance sweep")) -> ()
                      }
                      frame True {
                        n1057 = local read "Output Power (mW)"() -> (w1687:dbl)
                        n1058 = Multiply(x=w1687, y=0.001) -> (x*y=w1685:dbl)
                        n1059 = local write "I compliance sweep"(w1685) -> ()
                      }
                    }
                  }
                }
              }
            }
          }
          frame "Zero Laser" {
            # "Does not actually update laser - just changer the laser current variable to zero."
            n1060 = local write "Laser Current (mA)"(0.0) -> ()
          }
          frame "raw mask updated" {
            # "Asks if the manual mask should be updated to match the new raw mask file"
            n1061 = Enqueue Element At Opposite End(queue=w1697, element="idle", error in (no error)=w1696) -> (queue out=w1699:refnum<queue>, error out=w1698:errorcluster)  [unwired: 1 in, 1 out]
            n1062 = Two Button Dialog(message="Wold you like to update the Manual mask?", 1:"No" ("F button name (\"Cancel\")"), 2:"Yes" ("T button name (\"OK\")")) -> (T button?=w1691:bool)
            n1063 = case shown="True" w1691 {
              frame False {
              }
              frame True {
                n1064 = local read "Mask File Raw"() -> (w1700:path)
                n1065 = local write "Mask File Manual"(w1700) -> ()
              }
            }
          }
          frame "mask manual update" {
            # "asks if the raw test mask should be changed to math manual mask"
            n1066 = Enqueue Element At Opposite End(queue=w1707, element="idle", error in (no error)=w1706) -> (queue out=w1709:refnum<queue>, error out=w1708:errorcluster)  [unwired: 1 in, 1 out]
            n1067 = Two Button Dialog(message="Would you like update mask file for raw test?", 1:"No" ("F button name (\"Cancel\")"), 2:"Yes" ("T button name (\"OK\")")) -> (T button?=w1701:bool)
            n1068 = case shown="True" w1701 {
              frame False {
              }
              frame True {
                n1069 = local read "Mask File Manual"() -> (w1710:path)
                n1070 = local write "Mask File Raw"(w1710) -> ()
              }
            }
          }
          frame "save comment" {
            # "Uses activex to open the measurement log, save the comment to the approprate cell, and attempt to close the file again. As it stands, the file always stays open after this is run."
            n1071 = flat-sequence {
              frame #0 {
                # "6"
                # "5"
                # "4"
                # "3"
                # "2"
                # "1"
                # "This example demonstrates how to close a Worksheet from an Excel Workbook. \n\nThe steps are as follows:\n1) Open Excel\n2) Open the specific workbook\n3) Open a Specific Sheet\n4) Find a range in that sheet to clear \n5) For adding individual data points, you can use the same range refnum to send in coordinates and the new values. \n6) Close all open references"
                n1072 = Path To String(path="Measurement Log Path") -> (string=w1713:string)
                n1073 = Automation Open(Automation Refnum=refnum<k7> refnum ("Excel._Application")) -> (Automation Refnum=w1760:refnum<k7>, error out=w1759:errorcluster)  [unwired: 3 in]
                n1074 = property on="Property Node" class="_Application"(reference=w1760, error in=w1759, "Visible"=TRUE) -> (reference out=w1756:refnum<k7>, error out=w1755:errorcluster, "Workbooks"=w1757:refnum<k7>)
                n1075 = invoke on="Invoke Node" class="Workbooks" method="Open"(reference=w1757, error in=w1755, "Filename"=w1713, "ReadOnly"=FALSE, "Editable"=TRUE) -> (error out=w1754:errorcluster, "Open"=w1725:refnum<k7>)  [unwired: 13 in, 16 out]
                n1076 = property on="Property Node" class="_Workbook"(reference=w1725, error in=w1754) -> (reference out=w1722:refnum<k7>, error out=w1753:errorcluster, "Worksheets"=w1748:refnum<k7>)
                n1077 = invoke on="Invoke Node" class="Sheets" method="Item"(reference=w1748, error in=w1753, "Index"="MeasurementLog") -> (reference out=w1742:refnum<k7>, error out=w1747:errorcluster, "Item"=w1750:variant)  [unwired: 1 in, 1 out]
                n1078 = local read "Logview"() -> (w1761:i32)
                n1079 = Variant To Data(error in=w1747, type=refnum<k7> refnum ("reference"), Variant=w1750) -> (data=w1720:refnum<k7>, error out=w1735:errorcluster)
                n1080 = Build Array(w1761) -> (w1731:i32[])
                n1081 = To Variant(anything="A1") -> (Variant=w1743:variant)
                n1082 = To Variant(anything="A1") -> (Variant=w1744:variant)
                n1083 = local read "Add Comments"() -> (w1732:string)
                n1084 = invoke on="Invoke Node" class="_Worksheet" method="Range"(reference=w1720, error in=w1735, "Cell1"=w1743, "Cell2"=w1744) -> (error out=w1734:errorcluster, "Range"=w1737:refnum<k7>)  [unwired: 1 in, 3 out]
                n1085 = Index Array(array=w1731, index=0) -> (element=w1728:i32)
                n1086 = Add(x=w1728, y=1) -> (x+y=w1726:i32)
                n1087 = invoke on="Invoke Node" class="Range" method="ListNames"(reference=w1737, error in=w1734) -> (reference out=w1736:refnum<k7>, error out=w1733:errorcluster)  [unwired: 1 in, 1 out]
                n1088 = To Variant(anything=w1732) -> (Variant=w1740:variant)
                n1089 = invoke on="Invoke Node" class="Range" method="Item"(reference=w1736, error in=w1733, "RowIndex"=w1726, "ColumnIndex"=7, "newValue"=w1740) -> (reference out=w1738:refnum<k7>, error out=w1721:errorcluster)  [unwired: 1 in, 4 out]
                n1090 = invoke class="_Worksheet" method="SaveAs"(reference=w1720, error in=w1721, "Filename"=w1713) -> (reference out=w1716:refnum<k7>, error out=w1715:errorcluster)  [unwired: 10 in, 11 out]
                n1091 = Close Reference(reference=w1738, error in (no error)=w1715) -> (error out=w1749:errorcluster)
                n1092 = Close Reference(reference=w1742, error in (no error)=w1749) -> (error out=w1723:errorcluster)
                n1093 = Close Reference(reference=w1722, error in (no error)=w1723) -> (error out=w1724:errorcluster)
                n1094 = Close Reference(reference=w1756, error in (no error)=w1724) -> (error out=w1718:errorcluster)
                n1095 = Close Reference(reference=w1716, error in (no error)=w1718) -> (error out=w1717:errorcluster)
                n1096 = call <vilib>:"Simple Error Handler.vi"("error in (no error)"=w1717) -> ()  [unwired: 4 in, 5 out]
              }
            }
          }
          frame "update viewer" {
            # "Makes the logview table match the measurements log csv"
            n1097 = call-poly <vilib>:"Read From Spreadsheet File.vi"("file path (dialog if empty)"=path "C:/Users/Flash/Desktop/Data/Detector test data/MeasurementLog.csv") -> ("all rows"=w1764:string[][])  [unwired: 6 in, 4 out]
            n1098 = property on="Logview" class="MCListbox (strict)"("ItemNames"=w1764) -> ()  [unwired: 2 in, 2 out]
          }
          frame "refresh device names" {
            # "Ideally populates device nam elist for auto test with devices from the appropriate mask file. Isnt woking at this time, the user needs to manually type in device names"
            n1099 = Enqueue Element At Opposite End(queue=w1775, element="idle", error in (no error)=w1774) -> (queue out=w1776:refnum<queue>, error out=w1771:errorcluster)  [unwired: 1 in, 1 out]
            n1100 = call "getDB unique Device.vi"("error in (no error)"=w1771, "Mask"="Mask Name") -> ("NameList"=w1767:string[])  [unwired: 8 in, 1 out]
            "NameList" <- w1767
            n1101 = Equal?(x=w1767, y=string[] []) -> (x = y?=w1769:bool[])
            n1102 = And Array Elements(Boolean array=w1769) -> (logical AND=w1768:bool)
            n1103 = case shown="True" w1768 {
              tunnel: w1767 -> [w1777 w1779]
              tunnel: [w1777 w1778] -> w1766
              frame False {
              }
              frame True {
                n1104 = call "Prompt User for Input"() -> ("YES"=w1780:bool)  [unwired: 18 in, 1 out]
                n1105 = case shown="True" w1780 {
                  tunnel: w1779 -> [w1781 _]
                  tunnel: [w1781 w1782] -> w1778
                  frame False {
                  }
                  frame True {
                    # "GET DEVICES FROM FILE"
                    n1106 = local read "Mask File all"() -> (w1783:path)
                    n1107 = call "Select unique devices from File.vi"("MaskFile"=w1783) -> ("Device Array"=w1782:string[])  [unwired: 10 in]
                  }
                }
              }
            }
            n1108 = property on="Available Device Name" class="CmbBox"("Strings[]"=w1766) -> ()  [unwired: 2 in, 2 out]
          }
          frame "add to list" {
            # "Adds available device name to test list. If Skip Raw Test Is selected, it appends (skip) on the device name, which the auto test uses to know when to skip the raw test."
            n1109 = Enqueue Element At Opposite End(queue=w1787, element="idle", error in (no error)=w1785) -> (queue out=w1789:refnum<queue>, error out=w1788:errorcluster)  [unwired: 1 in, 1 out]
            n1110 = case shown="False" "Skip Raw Test?" {
              frame False {
                n1111 = local read "Available Device Name"() -> (w1791:string)
                n1112 = property on="Test List" class="LstBox (strict)"() -> ("Item Names"=w1790:string[])  [unwired: 2 in, 2 out]
                n1113 = Build Array (concatenate)(w1790, w1791) -> (w1792:string[])
                n1114 = property on="Test List" class="LstBox (strict)"("Item Names"=w1792) -> ()  [unwired: 2 in, 2 out]
              }
              frame True {
                n1115 = local read "Available Device Name"() -> (w1795:string)
                n1116 = property on="Test List" class="LstBox (strict)"() -> ("Item Names"=w1796:string[])  [unwired: 2 in, 2 out]
                n1117 = Concatenate Strings(w1795, "(skip)" ("string")) -> (w1793:string)
                n1118 = Build Array (concatenate)(w1796, w1793) -> (w1797:string[])
                n1119 = property on="Test List" class="LstBox (strict)"("Item Names"=w1797) -> ()  [unwired: 2 in, 2 out]
              }
            }
          }
          frame "skip raw?" {
            # "First checks to see of (skip) is appended on the current device name. If it isnt, it sets \"raw test skipped\" to false. It (skip) is appended on the end, then it removes it and sets \"raw test skipped\" to true."
            n1120 = property on="Test List" class="LstBox (strict)"() -> ("Item Names"=w1806:string[])  [unwired: 2 in, 2 out]
            n1121 = local read "Counter"() -> (w1805:i32)
            n1122 = Index Array(array=w1806, index=w1805) -> (element=w1804:string)
            "device name w skip" <- w1804
            n1123 = Search/Split String(string=w1804, search string/char (-)="(skip)") -> (match + rest of string=w1802:string)  [unwired: 1 in, 2 out]
            n1124 = Equal?(x=w1802, y="") -> (x = y?=w1800:bool)
            n1125 = local write "no file"(FALSE ("no file")) -> ()
            n1126 = Not(x=w1800) -> (.not. x?=w1799:bool)
            n1127 = case shown="False" w1799 {
              frame False {
                n1128 = local write "Raw Test Skipped"(FALSE ("Skipped")) -> ()
              }
              frame True {
                n1129 = flat-sequence {
                  tunnel: [w1815] -> w1812
                  tunnel: [w1814] -> w1811
                  tunnel: [w1813] -> w1810
                  tunnel: w1812 -> [w1823]
                  tunnel: w1811 -> [w1822]
                  tunnel: w1810 -> [w1821]
                  frame #0 {
                    n1130 = property on="Test List" class="LstBox (strict)"() -> ("Item Names"=w1815:string[])  [unwired: 2 in, 2 out]
                    n1131 = local read "Counter"() -> (w1814:i32)
                    n1132 = Index Array(array=w1815, index=w1814) -> (element=w1817:string)
                    n1133 = Search/Split String(string=w1817, search string/char (-)="(skip)") -> (substring before match=w1813:string)  [unwired: 1 in, 2 out]
                  }
                  frame #1 {
                    n1134 = Delete From Array(array=w1823, index=w1822) -> (array with subset deleted=w1820:string[])  [unwired: 1 in, 1 out]
                    n1135 = Insert Into Array(array=w1820, index=w1822, new element=w1821) -> (w1819:string[])
                    n1136 = property on="Test List" class="LstBox (strict)"("Item Names"=w1819) -> ()  [unwired: 2 in, 2 out]
                    "Raw Test Skipped" <- TRUE ("Skipped")
                  }
                }
              }
            }
          }
          frame "add to laser list" {
            # "Adds \"desired current\" value to current list"
            n1137 = property on="Laser List" class="LstBox (strict)"() -> ("Item Names"=w1828:string[])  [unwired: 2 in, 2 out]
            n1138 = local read "Desired Current (mA)"() -> (w1825:dbl)
            n1139 = Format Into String(format string="%08.4f", w1825) -> (resulting string=w1824:string)  [unwired: 2 in, 1 out]
            n1140 = Build Array (concatenate)(w1828, w1824) -> (w1827:string[])
            n1141 = property on="Laser List" class="LstBox (strict)"("Item Names"=w1827) -> ()  [unwired: 2 in, 2 out]
          }
          frame "remove from laser list" {
            # "removes highlighted value from laser list"
            n1142 = local read "Laser List"() -> (w1835:i32)
            n1143 = property on="Laser List" class="LstBox (strict)"() -> ("Item Names"=w1834:string[])  [unwired: 2 in, 2 out]
            n1144 = Delete From Array(array=w1834, index=w1835) -> (array with subset deleted=w1833:string[])  [unwired: 1 in, 1 out]
            n1145 = property on="Laser List" class="LstBox (strict)"("Item Names"=w1833) -> ()  [unwired: 2 in, 2 out]
          }
          frame "clear laser list" {
            # "removes all values from laser list"
            n1146 = property on="Laser List" class="LstBox (strict)"("Item Names"=string[] []) -> ()  [unwired: 2 in, 2 out]
          }
          frame "remove from list" {
            # "removes highlighted value from test list"
            n1147 = property on="Test List" class="LstBox (strict)"() -> ("Item Names"=w1841:string[])  [unwired: 2 in, 2 out]
            n1148 = local read "Test List"() -> (w1839:i32)
            n1149 = Enqueue Element At Opposite End(queue=w1843, element="idle", error in (no error)=w1842) -> (queue out=w1845:refnum<queue>, error out=w1844:errorcluster)  [unwired: 1 in, 1 out]
            n1150 = Delete From Array(array=w1841, index=w1839) -> (array with subset deleted=w1840:string[])  [unwired: 1 in, 1 out]
            n1151 = property on="Test List" class="LstBox (strict)"("Item Names"=w1840) -> ()  [unwired: 2 in, 2 out]
          }
          frame "clear list" {
            # "removes all values from test list"
            n1152 = property on="Test List" class="LstBox (strict)"("Item Names"=string[] []) -> ()  [unwired: 2 in, 2 out]
            n1153 = Enqueue Element(queue=w1850, element="idle", error in (no error)=w1848) -> (queue out=w1852:refnum<queue>, error out=w1851:errorcluster)  [unwired: 1 in, 1 out]
          }
          frame "add to temp list" {
            # "Adds \"desired temperature\" valiue to temp list"
            n1154 = local read "Desired Temperature"() -> (w1856:dbl)
            n1155 = property on="Single Device Temperature List" class="LstBox (strict)"() -> ("Item Names"=w1855:string[])  [unwired: 2 in, 2 out]
            n1156 = Format Into String(format string="%08.4f", w1856) -> (resulting string=w1854:string)  [unwired: 2 in, 1 out]
            n1157 = Build Array (concatenate)(w1855, w1854) -> (w1853:string[])
            n1158 = property on="Single Device Temperature List" class="LstBox (strict)"("Item Names"=w1853) -> ()  [unwired: 2 in, 2 out]
          }
          frame "remove from temp list" {
            # "Removes highlighted value from temperatre list"
            n1159 = property on="Single Device Temperature List" class="LstBox (strict)"() -> ("Item Names"=w1862:string[])  [unwired: 2 in, 2 out]
            n1160 = local read "Single Device Temperature List"() -> (w1861:i32)
            n1161 = Delete From Array(array=w1862, index=w1861) -> (array with subset deleted=w1860:string[])  [unwired: 1 in, 1 out]
            n1162 = property on="Single Device Temperature List" class="LstBox (strict)"("Item Names"=w1860) -> ()  [unwired: 2 in, 2 out]
          }
          frame "clear temp list" {
            # "Removes all values from temp list"
            n1163 = property on="Single Device Temperature List" class="LstBox (strict)"("Item Names"=string[] []) -> ()  [unwired: 2 in, 2 out]
          }
          frame "pick device" {
            # "Takes the device for the current iteration of the auto test and updates the test name. The Counter keeps track of which iteration of the auto test the program is running. After the device name is updated, the counter is incremented by one. If th elast device is reached, the counter is reset to zero for the next test."
            n1164 = Enqueue Element(queue=w1872, element="idle", error in (no error)=w1870) -> (queue out=w1871:refnum<queue>, error out=w1869:errorcluster)  [unwired: 1 in, 1 out]
            n1165 = flat-sequence {
              frame #0 {
                n1166 = local read "Mask File all"() -> (w1875:path)
                n1167 = property on="Test List" class="LstBox (strict)"() -> ("Item Names"=w1877:string[])  [unwired: 2 in, 2 out]
                n1168 = local read "Counter"() -> (w1876:i32)
                n1169 = Index Array(array=w1877, index=w1876) -> (element=w1873:string)
                n1170 = local write "Device Name"(w1873) -> ()
                n1171 = call "Mask file select device.vi"("Device"=w1873, "MaskFile"=w1875) -> ("RawMask"=w1874:path)  [unwired: 9 in]
                n1172 = local write "Mask File Raw"(w1874) -> ()
              }
              frame #1 {
                n1173 = local read "Counter"() -> (w1879:i32)
                n1174 = Increment(x=w1879) -> (x+1=w1878:i32)
                n1175 = local write "Counter"(w1878) -> ()
              }
              frame #2 {
                n1176 = property on="Test List" class="LstBox (strict)"() -> ("Item Names"=w1882:string[])  [unwired: 2 in, 2 out]
                n1177 = local read "Counter"() -> (w1883:i32)
                n1178 = Array Size(array=w1882) -> (size(s)=w1881:i32)
                n1179 = Equal?(x=w1883, y=w1881) -> (x = y?=w1880:bool)
                n1180 = case shown="False" w1880 {
                  frame False {
                  }
                  frame True {
                    n1181 = local write "Counter"(0 ("Counter")) -> ()
                  }
                }
              }
            }
          }
          frame "pick laser" {
            # "See pick device. Mechanics are exactly the same, except for laser instead of device name"
            n1182 = flat-sequence {
              frame #0 {
                n1183 = property on="Laser List" class="LstBox (strict)"() -> ("Item Names"=w1889:string[])  [unwired: 2 in, 2 out]
                n1184 = local read "Laser Counter"() -> (w1890:i32)
                n1185 = Index Array(array=w1889, index=w1890) -> (element=w1888:string)
                n1186 = Fract/Exp String To Number(string=w1888) -> (number=w1887:dbl)  [unwired: 3 in, 1 out]
                n1187 = local write "Laser Current (mA)"(w1887) -> ()
              }
              frame #1 {
                n1188 = local read "Laser Counter"() -> (w1892:i32)
                n1189 = Increment(x=w1892) -> (x+1=w1891:i32)
                n1190 = local write "Laser Counter"(w1891) -> ()
              }
              frame #2 {
                n1191 = property on="Laser List" class="LstBox (strict)"() -> ("Item Names"=w1893:string[])  [unwired: 2 in, 2 out]
                n1192 = local read "Laser Counter"() -> (w1896:i32)
                n1193 = Array Size(array=w1893) -> (size(s)=w1895:i32)
                n1194 = Equal?(x=w1896, y=w1895) -> (x = y?=w1894:bool)
                n1195 = case shown="True" w1894 {
                  frame False {
                  }
                  frame True {
                    n1196 = local write "Laser Counter"(0 ("Counter")) -> ()
                  }
                }
              }
            }
          }
          frame "reset skip" {
            # "If the raw test was skipped, during the auto test the (skip) tag was removed from the device mane during testing. This replaces the (skip)tag so the user can run another test"
            n1197 = local read "Counter"() -> (w1900:i32)
            n1198 = property on="Test List" class="LstBox (strict)"() -> ("Item Names"=w1902:string[])  [unwired: 2 in, 2 out]
            n1199 = Not Equal?(x=w1900, y=0) -> (x != y?=w1898:bool)
            n1200 = case shown="False" w1898 {
              tunnel: w1902 -> [w1907 w1916]
              tunnel: [w1908 w1912] -> w1901
              frame False {
                n1201 = Array Size(array=w1907) -> (size(s)=w1906:i32)
                n1202 = local read "device name w skip"() -> (w1910:string)
                n1203 = Decrement(x=w1906) -> (x-1=w1905:i32)
                n1204 = Delete From Array(array=w1907, index=w1905) -> (array with subset deleted=w1909:string[])  [unwired: 1 in, 1 out]
                n1205 = Insert Into Array(array=w1909, index=w1905, new element=w1910) -> (w1908:string[])
              }
              frame True {
                n1206 = local read "Counter"() -> (w1913:i32)
                n1207 = local read "device name w skip"() -> (w1915:string)
                n1208 = Subtract(x=w1913, y=1) -> (x-y=w1911:i32)
                n1209 = Delete From Array(array=w1916, index=w1911) -> (array with subset deleted=w1914:string[])  [unwired: 1 in, 1 out]
                n1210 = Insert Into Array(array=w1914, index=w1911, new element=w1915) -> (w1912:string[])
              }
            }
            n1211 = property on="Test List" class="LstBox (strict)"("Item Names"=w1901) -> ()  [unwired: 2 in, 2 out]
          }
          frame "load wafer" {
            # "tells probe station to load wafer"
            n1212 = flat-sequence {
              frame #0 {
                n1213 = local read "Prober GPIB"() -> (w1924:string)
                n1214 = local write "Status"("loading..." ("Status")) -> ()
                n1215 = call "EG2001 Load Wafer.vi"("Enable Error Message"=FALSE, "error in (no error)"=errorcluster {"status"=FALSE, "code"=0, "source"=""}, "Characters to Write"="LO", "GPIB Address"=w1924) -> ()  [unwired: 5 in, 3 out]
              }
              frame #1 {
                n1216 = local write "Status"("load complete" ("Status")) -> ()
              }
            }
          }
          frame "profile z" {
            # "tells pobe station to run \"profile z\" program"
            n1217 = local read "Prober GPIB"() -> (w1927:string)
            n1218 = call "EG2001 Profile Wafer Only.vi"("GPIB Address"=w1927) -> ("Error Out"=→"Error Out":errorcluster)  [unwired: 9 in, 1 out]
          }
          frame "auto align" {
            # "tells prober to run \"auto align\" feature. Only works if ref is already stored, if find target needs to be run, that needs to be done manually, (see prober guide for details)."
            n1219 = flat-sequence {
              frame #0 {
                n1220 = local read "Prober GPIB"() -> (w1933:string)
                n1221 = local write "Status"("aligning" ("Status")) -> ()
                n1222 = call "EG2001 Auto Align Wafer.vi"("GPIB Address"=w1933) -> ()  [unwired: 8 in, 3 out]
              }
              frame #1 {
                n1223 = local write "Status"("idle" ("Status")) -> ()
              }
            }
          }
          frame "wait" {
            # "delays for a certain number of seconds, determined by the \"wait after load\" parameter"
            n1224 = Multiply(x="Wait after load", y=u32 1000) -> (x*y=w1935:u32)
            n1225 = Wait (ms)(milliseconds to wait=w1935) -> ()  [unwired: 1 out]
          }
          frame "add to wafer list" {
            # "adds \"desired wafer name\" to wafer list"
            n1226 = property on="Wafer List" class="LstBox (strict)"() -> ("Item Names"=w1941:string[])  [unwired: 2 in, 2 out]
            n1227 = local read "Desired Wafer Name"() -> (w1942:string)
            n1228 = Build Array (concatenate)(w1941, w1942) -> (w1940:string[])
            n1229 = property on="Wafer List" class="LstBox (strict)"("Item Names"=w1940) -> ()  [unwired: 2 in, 2 out]
          }
          frame "remove from wafer list" {
            # "Removes highlighted value from wafer list"
            n1230 = property on="Wafer List" class="LstBox (strict)"() -> ("Item Names"=w1946:string[])  [unwired: 2 in, 2 out]
            n1231 = local read "Wafer List"() -> (w1947:i32)
            n1232 = Delete From Array(array=w1946, index=w1947) -> (array with subset deleted=w1945:string[])  [unwired: 1 in, 1 out]
            n1233 = property on="Wafer List" class="LstBox (strict)"("Item Names"=w1945) -> ()  [unwired: 2 in, 2 out]
          }
          frame "clear wafer list" {
            # "Deletes all values in wafer list"
            n1234 = property on="Wafer List" class="LstBox (strict)"("Item Names"=string[] []) -> ()  [unwired: 2 in, 2 out]
          }
          frame "desired device change" {
            # "works the same as \"die number changed\" but in the temperature tab"
            n1235 = flat-sequence {
              frame #0 {
                n1236 = local read "Desired Device"() -> (w1962:u16)
                n1237 = local read "Array of Cell Data Clusters"() -> (w1963:T13)
                n1238 = Index Array(array=w1963, index=w1962) -> (element=w1961:T18)
                n1239 = Unbundle By Name(w1961) -> ("Cell Name"=w1960:string, "X-coord"=w1957:dbl, "Y-coord"=w1956:dbl, "Area"=w1959:dbl, "Meas Area"=w1958:dbl)
                "X" <- w1957
                "Y" <- w1956
                n1240 = local write "Device Name"(w1960) -> ()
                n1241 = local write "x target"(w1957) -> ()
                n1242 = local write "y target"(w1956) -> ()
                n1243 = local write "ActiveArea_um2"(w1959) -> ()
                n1244 = local write "MesaArea_um2"(w1958) -> ()
              }
              frame #1 {
                n1245 = local read "J set A/cm2"() -> (w1969:dbl)
                n1246 = local read "Laser Current (mA)"() -> (w1966:dbl)
                n1247 = Equal To 0?(x=w1966) -> (x = 0?=w1965:bool)
                n1248 = case shown="True" w1965 {
                  tunnel: [w1971 w1972] -> w1964
                  frame False {
                    n1249 = local read "ActiveArea_um2"() -> (w1971:dbl)
                  }
                  frame True {
                    n1250 = local read "MesaArea_um2"() -> (w1972:dbl)
                  }
                }
                n1251 = Divide(x=w1964, y=100000000.0) -> (x/y=w1968:dbl)
                n1252 = Multiply(x=w1968, y=w1969) -> (x*y=w1970:dbl)
                n1253 = local write "I set"(w1970) -> ()
              }
            }
            n1254 = local write "Status"("Changing Die" ("Status")) -> ()
          }
          frame "select temperature" {
            # "Updates the current temperature from the temperature list, and updates the counter, which operates the same as laser, wafer, and auto test counters"
            n1255 = flat-sequence {
              frame #0 {
                n1256 = local read "Auto Temp Counter"() -> (w1978:i32)
                n1257 = property on="Auto Temperature List" class="LstBox (strict)"() -> ("Item Names"=w1975:string[])  [unwired: 2 in, 2 out]
                n1258 = local write "Status"("selecting temperature" ("Status")) -> ()
                n1259 = Index Array(array=w1975, index=w1978) -> (element=w1976:string)
                n1260 = local write "Temp Setpoint"(w1976) -> ()
              }
              frame #1 {
                n1261 = local read "Auto Temp Counter"() -> (w1980:i32)
                n1262 = Increment(x=w1980) -> (x+1=w1979:i32)
                n1263 = local write "Auto Temp Counter"(w1979) -> ()
              }
              frame #2 {
                n1264 = property on="Auto Temperature List" class="LstBox (strict)"() -> ("Item Names"=w1981:string[])  [unwired: 2 in, 2 out]
                n1265 = local read "Auto Temp Counter"() -> (w1984:i32)
                n1266 = Array Size(array=w1981) -> (size(s)=w1983:i32)
                n1267 = Equal?(x=w1984, y=w1983) -> (x = y?=w1982:bool)
                n1268 = case shown="True" w1982 {
                  frame False {
                  }
                  frame True {
                    n1269 = local write "Auto Temp Counter"(0 ("Counter")) -> ()
                  }
                }
              }
            }
          }
          frame "wait for temperature" {
            # "This while loop checks every five seconds whether the temperature has reached the setpoint, and if it has it exits the while loop and allows the program to continue"
            n1270 = local read "Temp Controller Found"() -> (w1986:bool)
            n1271 = case shown="True" w1986 {
              frame False {
              }
              frame True {
                n1272 = while {
                  i -> [w1992]
                  stop <- w1989 stop-if-true
                  n1273 = flat-sequence {
                    tunnel: [w1998] -> w1991
                    tunnel: w1992 -> [w2006]
                    tunnel: [w2005] -> w1990
                    frame #0 {
                      n1274 = local read "Temptronics VISA"() -> (w2002:refnum<visa-resource-name>)
                      n1275 = Wait (ms)(milliseconds to wait=u32 500) -> ()  [unwired: 1 out]
                      n1276 = VISA Write(VISA resource name=w2002, write buffer="st") -> (VISA resource name out=w2001:refnum<visa-resource-name>, return count=w2000:u32)  [unwired: 1 in, 1 out]
                      n1277 = local read "Temp Setpoint"() -> (w1994:string)
                      n1278 = local write "Status"("waiting for temperature..." ("Status")) -> ()
                      n1279 = VISA Read(VISA resource name=w2001, byte count=w2000) -> (read buffer=w1996:string)  [unwired: 1 in, 3 out]
                      n1280 = Decimal String To Number(string=w1996) -> (number=w1995:i32)  [unwired: 2 in, 1 out]
                      n1281 = Decimal String To Number(string=w1994) -> (number=w1993:i32)  [unwired: 2 in, 1 out]
                      n1282 = Equal?(x=w1995, y=w1993) -> (x = y?=w1998:bool)
                    }
                    frame #1 {
                      n1283 = Equal?(x=w2006, y=500) -> ()  [unwired: 1 out]
                      n1284 = case shown="False" FALSE {
                        tunnel: [_ w2008] -> w2005
                        frame False {
                        }
                        frame True {
                          n1285 = One Button Dialog(message="Temperature Timeout") -> (true=w2008:bool)  [unwired: 1 in]
                        }
                      }
                    }
                  }
                  n1286 = Or(x=w1990, y=w1991) -> (x .or. y?=w1989:bool)
                }
              }
            }
          }
          frame "temp to 25" {
            n1287 = local write "Temp Setpoint"("25" ("Temp Setpoint")) -> ()
          }
          frame "load file for temp" {
            # "same as load manual mask file, but in the temperature tab"
            n1288 = flat-sequence {
              tunnel: [w2023] -> w2018
              tunnel: w2018 -> [w2026]
              frame #0 {
                n1289 = local read "Mask File Temperature"() -> (w2019:path)
                n1290 = local write "Status"("Loading mask file" ("Status")) -> ()
                n1291 = call "Device Files v1.vi"("Rows"=1200, "Mask file path"=w2019) -> ("Mask Name"=w2024:string, "size(s)"=w2023:i32, "Array of Cell Clusters"=w2020:T6)  [unwired: 6 in, 1 out]
                n1292 = local write "Mask"(w2024) -> ()
                n1293 = local write "Array of Cell Data Clusters"(w2020) -> ()
              }
              frame #1 {
                n1294 = for {
                  N: w2026 -> [_]
                  tunnel: [w2027] -> w2025 mode=indexing
                  i -> [w2028]
                  n1295 = Number To Decimal String(number=w2028) -> (decimal integer string=w2027:string)  [unwired: 1 in]
                }
                n1296 = property on="Desired Device" class="Ring (strict)"("Strings []"=w2025) -> ()  [unwired: 2 in, 2 out]
              }
              frame #2 {
                n1297 = local read "Array of Cell Data Clusters"() -> (w2036:T13)
                n1298 = local read "Desired Device"() -> (w2035:u16)
                n1299 = Index Array(array=w2036, index=w2035) -> (element=w2034:T18)
                n1300 = Unbundle By Name(w2034) -> ("Cell Name"=w2029:string, "X-coord"=w2032:dbl, "Y-coord"=w2033:dbl, "Area"=w2031:dbl, "Meas Area"=w2030:dbl)
                n1301 = local write "Device Name"(w2029) -> ()
                n1302 = local write "x target"(w2032) -> ()
                n1303 = local write "y target"(w2033) -> ()
                n1304 = local write "ActiveArea_um2"(w2031) -> ()
                n1305 = local write "MesaArea_um2"(w2030) -> ()
              }
              frame #3 {
                n1306 = local read "Laser Current (mA)"() -> (w2039:dbl)
                n1307 = Equal To 0?(x=w2039) -> (x = 0?=w2038:bool)
                n1308 = case shown="False" w2038 {
                  tunnel: [w2044 w2045] -> w2037
                  frame False {
                    n1309 = local read "ActiveArea_um2"() -> (w2044:dbl)
                  }
                  frame True {
                    n1310 = local read "MesaArea_um2"() -> (w2045:dbl)
                  }
                }
                n1311 = local read "J set A/cm2"() -> (w2042:dbl)
                n1312 = Divide(x=w2037, y=100000000.0) -> (x/y=w2041:dbl)
                n1313 = Multiply(x=w2041, y=w2042) -> (x*y=w2043:dbl)
                n1314 = local write "I set"(w2043) -> ()
              }
            }
            n1315 = Enqueue Element(queue=w2017, element="idle", error in (no error)=w2015) -> (queue out=w2016:refnum<queue>, error out=w2014:errorcluster)  [unwired: 1 in, 1 out]
          }
          frame "begin temperature series" {
            # "In Progress"
            n1316 = flat-sequence {
              frame #0 {
                n1317 = local read "Mask File Temperature"() -> (w2051:path)
                n1318 = local write "Status"("prepare temperature test" ("Status")) -> ()
                n1319 = local write "Mask File Temperature"(w2051) -> ()
                n1320 = local write "Tab Control"(T17."Temperature Series Single Device" ("Tab Control")) -> ()
                n1321 = local read "points"() -> (w2053:u16)
                n1322 = Initialize Array(nan ("element"), w2053) -> (w2055:dbl[])
                n1323 = call "Device Files v1.vi"("Rows"=1200, "Mask file path"=w2051) -> ("size(s)"=w2050:i32, "Array of Cell Clusters"=w2049:T6)  [unwired: 6 in, 2 out]
                n1324 = local write "Fine Cell Clusters"(w2049) -> ()
                n1325 = local write "Total Device"(w2050) -> ()
                n1326 = Bundle(w2055, w2055) -> (w2054:cluster{dbl[], dbl[]})  [unwired: 1 in]
                n1327 = Initialize Array(w2054, w2050) -> (w2048:cluster{dbl[], dbl[]}[])
                n1328 = local write "IV temp linear"(w2048) -> ()
                n1329 = local write "IV temp log"(w2048) -> ()
              }
              frame #1 {
                n1330 = property on="Single Device Temperature List" class="LstBox (strict)"() -> ("Item Names"=w2059:string[])  [unwired: 2 in, 2 out]
                n1331 = for {
                  tunnel: w2059 -> [_] mode=indexing
                  i -> [w2060]
                  n1332 = flat-sequence {
                    frame #0 {
                      n1333 = stacked-sequence {
                        frame #0 {
                          n1334 = property on="Single Device Temperature List" class="LstBox (strict)"() -> ("Item Names"=w2063:string[])  [unwired: 2 in, 2 out]
                          n1335 = local read "TempCounter"() -> (w2064:i32)
                          n1336 = local write "Status"("selecting temperature" ("Status")) -> ()
                          n1337 = Index Array(array=w2063, index=w2064) -> (element=w2061:string)
                          n1338 = local write "Temp Setpoint"(w2061) -> ()
                        }
                        frame #1 {
                          n1339 = local read "Temp Setpoint"() -> (w2072:string)
                          n1340 = local read "Temptronics VISA"() -> (w2070:refnum<visa-resource-name>)
                          n1341 = Concatenate Strings("rs" ("string"), w2072) -> (w2071:string)
                          n1342 = VISA Write(VISA resource name=w2070, write buffer=w2071) -> (VISA resource name out=w2069:refnum<visa-resource-name>)  [unwired: 1 in, 2 out]
                          n1343 = VISA Write(VISA resource name=w2069, write buffer="st") -> (VISA resource name out=w2067:refnum<visa-resource-name>, return count=w2066:u32)  [unwired: 1 in, 1 out]
                          n1344 = VISA Read(VISA resource name=w2067, byte count=w2066) -> (read buffer=w2065:string)  [unwired: 1 in, 3 out]
                          n1345 = local write "Current Temp"(w2065) -> ()
                        }
                        frame #2 {
                          n1346 = local read "TempCounter"() -> (w2075:i32)
                          n1347 = Increment(x=w2075) -> (x+1=w2074:i32)
                          n1348 = local write "TempCounter"(w2074) -> ()
                        }
                        frame #3 {
                          n1349 = property on="Single Device Temperature List" class="LstBox (strict)"() -> ("Item Names"=w2076:string[])  [unwired: 2 in, 2 out]
                          n1350 = local read "TempCounter"() -> (w2079:i32)
                          n1351 = Array Size(array=w2076) -> (size(s)=w2078:i32)
                          n1352 = Equal?(x=w2079, y=w2078) -> (x = y?=w2077:bool)
                          n1353 = case shown="False" w2077 {
                            frame False {
                            }
                            frame True {
                              n1354 = local write "TempCounter"(0 ("Counter")) -> ()
                            }
                          }
                        }
                      }
                    }
                    frame #1 {
                      n1355 = while {
                        i -> [w2084]
                        stop <- w2081 stop-if-true
                        n1356 = flat-sequence {
                          tunnel: [w2090] -> w2083
                          tunnel: w2084 -> [w2097]
                          tunnel: [w2096] -> w2082
                          frame #0 {
                            n1357 = local read "Temptronics VISA"() -> (w2094:refnum<visa-resource-name>)
                            n1358 = Wait (ms)(milliseconds to wait=u32 500) -> ()  [unwired: 1 out]
                            n1359 = VISA Write(VISA resource name=w2094, write buffer="st") -> (VISA resource name out=w2093:refnum<visa-resource-name>, return count=w2092:u32)  [unwired: 1 in, 1 out]
                            n1360 = local read "Temp Setpoint"() -> (w2086:string)
                            n1361 = local write "Status"("waiting for temperature..." ("Status")) -> ()
                            n1362 = VISA Read(VISA resource name=w2093, byte count=w2092) -> (read buffer=w2088:string)  [unwired: 1 in, 3 out]
                            n1363 = Decimal String To Number(string=w2088) -> (number=w2087:i32)  [unwired: 2 in, 1 out]
                            n1364 = Decimal String To Number(string=w2086) -> (number=w2085:i32)  [unwired: 2 in, 1 out]
                            n1365 = Equal?(x=w2087, y=w2085) -> (x = y?=w2090:bool)
                          }
                          frame #1 {
                            n1366 = Equal?(x=w2097, y=1000) -> (x = y?=w2099:bool)
                            n1367 = case shown="False" w2099 {
                              tunnel: [_ w2100] -> w2096
                              frame False {
                              }
                              frame True {
                                n1368 = One Button Dialog(message="Temperature Timeout") -> (true=w2100:bool)  [unwired: 1 in]
                              }
                            }
                          }
                        }
                        n1369 = Or(x=w2082, y=w2083) -> (x .or. y?=w2081:bool)
                      }
                    }
                    frame #2 {
                      n1370 = local read "Desired Device"() -> (w2114:u16)
                      n1371 = local write "Status"("IV test running..." ("string")) -> ()
                      n1372 = flat-sequence {
                        tunnel: [w2150] -> w2127
                        tunnel: [w2149] -> w2126
                        tunnel: [w2146] -> w2125
                        tunnel: [w2145] -> w2124
                        tunnel: [w2144] -> w2123
                        tunnel: [w2143] -> w2122
                        tunnel: [w2128] -> w2121
                        tunnel: w2114 -> [w2128]
                        tunnel: w2127 -> [w2166]
                        tunnel: w2126 -> [w2165]
                        tunnel: w2125 -> [w2163]
                        tunnel: w2124 -> [w2162]
                        tunnel: w2123 -> [w2161]
                        tunnel: w2122 -> [w2160]
                        tunnel: [w2159] -> w2120
                        tunnel: [w2158] -> w2119
                        tunnel: [w2157] -> w2118
                        tunnel: w2121 -> [w2157]
                        tunnel: w2120 -> [w2176]
                        tunnel: w2119 -> [w2175]
                        tunnel: [w2174] -> w2117
                        tunnel: w2118 -> [w2174]
                        tunnel: [w2188] -> w2116
                        tunnel: w2117 -> [w2188]
                        tunnel: [w2226] -> w2105
                        tunnel: [w2219] -> w2103
                        tunnel: w2116 -> [w2226]
                        tunnel: w2105 -> [w2237]
                        tunnel: [w2237] -> w2104
                        tunnel: w2103 -> [w2236]
                        tunnel: [w2236] -> w2102
                        tunnel: w2104 -> [_]
                        tunnel: [w2262] -> w2113
                        tunnel: [w2256] -> w2111
                        tunnel: [w2255] -> w2109
                        tunnel: w2102 -> [w2254]
                        tunnel: [w2250] -> w2107
                        tunnel: [w2248] -> w2106
                        tunnel: w2113 -> [w2279]
                        tunnel: [w2279] -> w2112
                        tunnel: w2111 -> [w2278]
                        tunnel: [w2278] -> w2110
                        tunnel: w2109 -> [w2277]
                        tunnel: [w2277] -> w2108
                        tunnel: w2107 -> [w2275]
                        tunnel: w2106 -> [w2276]
                        tunnel: w2112 -> [w2297]
                        tunnel: w2110 -> [w2291]
                        tunnel: w2108 -> [w2290]
                        frame #0 {
                          n1373 = local read "Output Power (mW)"() -> (w2133:dbl)
                          n1374 = local read "Fine Cell Clusters"() -> (w2155:T6)
                          n1375 = local read "ActiveArea_um2"() -> (w2135:dbl)
                          n1376 = local read "Laser Current (mA)"() -> (w2139:dbl)
                          n1377 = Multiply(x=w2133, y=0.001) -> (x*y=w2131:dbl)
                          n1378 = Divide(x=w2135, y=100000000.0) -> (x/y=w2130:dbl)
                          n1379 = local read "Output Power (mW)"() -> (w2136:dbl)
                          n1380 = Index Array(array=w2155, index=w2128) -> (element=w2140:T26)
                          n1381 = local read "Laser Current (mA)"() -> (w2137:dbl)
                          n1382 = local read "Parameters Flash 2"() -> (w2142:T5)
                          n1383 = Unbundle By Name(w2140) -> ("Cell Name"=w2154:string, "X-coord"=w2144:dbl, "Y-coord"=w2143:dbl, "Area"=w2153:dbl, "Mesa Area"=w2152:dbl)
                          n1384 = local read "current y"() -> (w2147:i32)
                          n1385 = local read "current x"() -> (w2148:i32)
                          n1386 = call "get Area.vi"("Laser"=w2139, "Cell Data Cluster"=w2140) -> ("Area"=w2141:dbl)  [unwired: 9 in]
                          n1387 = Divide(x=w2131, y=w2130) -> (x/y=w2129:dbl)
                          n1388 = local write "Device Name"(w2154) -> ()
                          n1389 = local write "ActiveArea_um2"(w2153) -> ()
                          n1390 = local write "MesaArea_um2"(w2152) -> ()
                          n1391 = Bundle By Name(cluster=w2142, "Cell Area (cm²)"=w2141, "Input Current (mA)"=w2137, "Power Density (W/cm^2)"=w2129, "Incident Power"=w2136) -> (w2138:T5)
                          n1392 = Subtract(x=w2143, y=w2147) -> (x-y=w2145:dbl)
                          n1393 = Subtract(x=w2144, y=w2148) -> (x-y=w2146:dbl)
                          n1394 = local write "Parameters Flash"(w2138) -> ()
                          n1395 = local read "Prober GPIB"() -> (w2151:string)
                          n1396 = call "EG2001 Move Z Down.vi"("GPIB Address"=w2151) -> ("Error Out"=w2149:errorcluster, "GPIB Address Out"=w2150:string)  [unwired: 9 in]
                        }
                        frame #1 {
                          n1397 = local write "current x"(w2161) -> ()
                          n1398 = local write "current y"(w2160) -> ()
                          n1399 = case shown="False" FALSE {
                            tunnel: w2166 -> [_ w2173]
                            tunnel: w2165 -> [_ w2172]
                            tunnel: enum32{"Steps", "Microns"}."Microns" ("Steps/Microns") -> [_ w2171]
                            tunnel: w2163 -> [_ w2170]
                            tunnel: w2162 -> [_ w2169]
                            tunnel: [_ w2168] -> w2159
                            tunnel: [_ w2167] -> w2158
                            frame False {
                            }
                            frame True {
                              n1400 = call "EG2001 Move Machine Step X-Y.vi"("Y"=w2169, "Steps/Microns"=w2171, "X"=w2170, "error in (no error)"=w2172, "GPIB Address"=w2173) -> ("Error Out"=w2167:errorcluster, "GPIB Address Out"=w2168:string)  [unwired: 5 in]
                            }
                          }
                        }
                        frame #2 {
                          n1401 = call "EG2001 Move Z Up.vi"("error in (no error)"=w2175, "GPIB Address"=w2176) -> ()  [unwired: 10 out]
                        }
                        frame #3 {
                          n1402 = local read "I compliance sweep"() -> (w2192:dbl)
                          n1403 = local read "Wafer Info Flash 2"() -> (w2187:T4)
                          n1404 = local read "sweep delay ms"() -> (w2191:dbl)
                          n1405 = local read "Sweep Settings"() -> (w2198:T11)
                          n1406 = local read "Temp Setpoint"() -> (w2182:string)
                          n1407 = local read "Device Name"() -> (w2186:string)
                          n1408 = local read "Channel"() -> (w2197:enum32{"Channel A", "Channel B"})
                          n1409 = call "DAQ Assistant2"() -> ("data"=w2180:dynamicdata)  [unwired: 17 in, 2 out]
                          n1410 = local read "Temp Data"() -> (w2183:T2)
                          n1411 = Bundle By Name(cluster=w2187, "Cell Name"=w2186) -> (w2185:T4)
                          n1412 = Decimal String To Number(string=w2182) -> (number=w2179:i32)  [unwired: 2 in, 1 out]
                          n1413 = local read "V start"() -> (w2195:dbl)
                          n1414 = local read "points"() -> (w2194:u16)
                          n1415 = local read "V end"() -> (w2196:dbl)
                          n1416 = local read "NPLC"() -> (w2193:dbl)
                          n1417 = Bundle By Name(cluster=w2183, "Ambient Temperature"=w2180, "Chuck Set Temperature"=w2179) -> (w2181:T2)
                          n1418 = local write "Wafer Info Flash"(w2185) -> ()
                          n1419 = Bundle By Name(cluster=w2198, "Channel"=w2197, "Vstart"=w2195, "Vend"=w2196, "# of points"=w2194, "NPLC"=w2193, "I compliance"=w2192, "Delay ms"=w2191) -> (w2177:T11)
                          n1420 = local read "Keysight"() -> (w2178:bool)
                          n1421 = local write "Temp Data"(w2181) -> ()
                          n1422 = local read "4-wire"() -> (w2184:bool)
                          n1423 = local write "Sweep Settings"(w2177) -> ()
                          n1424 = case shown="False" w2178 {
                            tunnel: w2177 -> [w2203 w2208]
                            tunnel: [w2201 w2206] -> w2190
                            tunnel: [w2200 w2205] -> w2189
                            tunnel: w2184 -> [w2199 w2207]
                            frame False {
                              n1425 = local read "Keithley SMU"() -> (w2202:refnum<visa-resource-name>)
                              n1426 = call "K2602 Vsweep.vi"("4-wire"=w2199, "Settings"=w2203, "SMU"=w2202) -> ("V"=w2200:dbl[], "I"=w2201:dbl[])  [unwired: 6 in, 1 out]
                            }
                            frame True {
                              n1427 = local read "Keysight SMU"() -> (w2204:refnum<visa-resource-name>)
                              n1428 = call "IVSweep (SubVI).vi"("SweepSettings"=w2208, "4 wire"=w2207, "VISA Refnum in"=w2204) -> ("V"=w2205:dbl[], "I"=w2206:dbl[])  [unwired: 1 in, 2 out]
                            }
                          }
                          n1429 = local write "I fine"(w2190) -> ()
                          n1430 = local write "V fine"(w2189) -> ()
                        }
                        frame #4 {
                          n1431 = local read "Temperature Series save path"() -> (w2218:path)
                          n1432 = local read "Device Name"() -> (w2210:string)
                          n1433 = local read "Wafer Info 3"() -> (w2209:T3)
                          n1434 = local read "Lot"() -> (w2217:string)
                          n1435 = Build Path(base path=w2218, name or relative path=w2217) -> (appended path=w2216:path)
                          n1436 = local read "Wafer Name"() -> (w2215:string)
                          n1437 = Bundle By Name(cluster=w2209, "Cell Name (Automatic)"=w2210) -> (w2211:T3)
                          n1438 = call "CreateDirectory.vi"("Path to be created"=w2216) -> ()  [unwired: 10 in, 1 out]
                          n1439 = local read "Output Power (mW)"() -> (w2224:dbl)
                          n1440 = Build Path(base path=w2216, name or relative path=w2215) -> (appended path=w2214:path)
                          n1441 = call "CreateDirectory.vi"("Path to be created"=w2214) -> ()  [unwired: 10 in, 1 out]
                          n1442 = local read "Device Name"() -> (w2225:string)
                          n1443 = local write "Wafer Info 3"(w2211) -> ()
                          n1444 = Build Path(base path=w2214, name or relative path="Temperature Series") -> (appended path=w2212:path)
                          n1445 = Number To Decimal String(number=w2224) -> (decimal integer string=w2222:string)  [unwired: 1 in]
                          n1446 = call "CreateDirectory.vi"("Path to be created"=w2212) -> ()  [unwired: 10 in, 1 out]
                          n1447 = Build Path(base path=w2212, name or relative path=w2225) -> (appended path=w2223:path)
                          n1448 = Concatenate Strings(w2222, " mW" ("string")) -> (w2220:string)
                          n1449 = call "CreateDirectory.vi"("Path to be created"=w2223) -> ()  [unwired: 10 in, 1 out]
                          n1450 = Build Path(base path=w2223, name or relative path=w2220) -> (appended path=w2219:path)
                          n1451 = call "CreateDirectory.vi"("Path to be created"=w2219) -> ()  [unwired: 10 in, 1 out]
                        }
                        frame #5 {
                          n1452 = local read "Sweep Direction (Keysight)"() -> (w2235:i32)
                          n1453 = local read "I compliance sweep"() -> (w2231:dbl)
                          n1454 = local read "sweep delay ms"() -> (w2230:dbl)
                          n1455 = local read "V start"() -> (w2234:dbl)
                          n1456 = local read "points"() -> (w2232:u16)
                          n1457 = local read "V end"() -> (w2233:dbl)
                          n1458 = call "pho_DBCheck_LIV_meas_recipe.vi"("V start"=w2234, "Sweep Direction (Keysight)"=w2235, "V end"=w2233, "points"=w2232, "I compliance sweep"=w2231, "sweep delay ms"=w2230) -> ("RecipeID"=w2229:string)  [unwired: 8 in, 1 out]
                          n1459 = local write "RecipeID"(w2229) -> ()
                          n1460 = Equal?(x=w2229, y="") -> (x = y?=w2227:bool)
                          n1461 = case shown="True" w2227 {
                            frame False {
                            }
                            frame True {
                              n1462 = local read "Sweep Direction (Keysight)"() -> (w2244:i32)
                              n1463 = local read "I compliance sweep"() -> (w2240:dbl)
                              n1464 = local read "sweep delay ms"() -> (w2239:dbl)
                              n1465 = local read "V start"() -> (w2243:dbl)
                              n1466 = local read "points"() -> (w2241:u16)
                              n1467 = local read "V end"() -> (w2242:dbl)
                              n1468 = call "pho_DB_Insert_LIV_meas_recipe.vi"("V start"=w2243, "Sweep Direction (Keysight)"=w2244, "V end"=w2242, "points"=w2241, "I compliance sweep"=w2240, "sweep delay ms"=w2239) -> ("RecipeID"=w2238:string)  [unwired: 9 in]
                              n1469 = local write "RecipeID"(w2238) -> ()
                            }
                          }
                        }
                        frame #6 {
                          n1470 = local read "I fine"() -> (w2267:dbl[])
                          n1471 = local read "Wafer Info 3"() -> (w2253:T3)
                          n1472 = local read "Comments"() -> (w2252:string)
                          n1473 = local read "V fine"() -> (w2261:dbl[])
                          n1474 = Absolute Value(x=w2267) -> (abs(x)=w2268:dbl[])
                          n1475 = local read "Temp Setpoint"() -> (w2247:string)
                          n1476 = local read "IV temp linear"() -> (w2273:cluster{dbl[], dbl[]}[])
                          n1477 = local read "IV temp log"() -> (w2269:cluster{dbl[], dbl[]}[])
                          n1478 = Bundle By Name(cluster=w2253, "Comment"=w2252) -> (w2251:T3)
                          n1479 = local read "iteration"() -> (w2250:i32)
                          n1480 = Bundle("V fine"=w2261, w2268) -> (w2266:cluster{"V fine":dbl[], dbl[]})  [unwired: 1 in]
                          n1481 = Bundle("V fine"=w2261, "I fine"=w2267) -> (w2271:cluster{"V fine":dbl[], "I fine":dbl[]})  [unwired: 1 in]
                          n1482 = local write "Wafer Info 3"(w2251) -> ()
                          n1483 = Replace Array Subset(array=w2269, new element=w2266, index=w2250) -> (w2270:cluster{dbl[], dbl[]}[])
                          n1484 = Replace Array Subset(array=w2273, new element=w2271, index=w2250) -> (w2272:cluster{dbl[], dbl[]}[])
                          n1485 = Decimal String To Number(string=w2247) -> (number=w2246:i32)  [unwired: 2 in, 1 out]
                          n1486 = local read "current y"() -> (w2257:i32)
                          n1487 = local read "current x"() -> (w2258:i32)
                          n1488 = local write "IV temp log"(w2270) -> ()
                          n1489 = local write "IV temp linear"(w2272) -> ()
                          n1490 = Number To Decimal String(number=w2246) -> (decimal integer string=w2245:string)  [unwired: 1 in]
                          n1491 = local read "Device Name"() -> (w2263:string)
                          n1492 = local read "Wafer Name"() -> (w2265:string)
                          n1493 = local read "Operator"() -> (w2264:string)
                          n1494 = To Double Precision Float(number=w2258) -> (double precision float=w2260:dbl)
                          n1495 = To Double Precision Float(number=w2257) -> (double precision float=w2259:dbl)
                          n1496 = Get Date/Time In Seconds() -> (seconds since 1Jan1904=w2255:timestamp)
                          n1497 = Concatenate Strings(w2245, " C" ("string")) -> (w2248:string)
                          n1498 = call "get Flash FileName .vi"("Time"=w2255, "Device Name"=w2263, "Operator"=w2264, "Wafer Name"=w2265, "FineTest save path"=w2254) -> ("appended path"=w2262:path)  [unwired: 6 in]
                          n1499 = Bundle(w2260, w2259) -> (w2256:cluster{dbl, dbl})  [unwired: 1 in]
                        }
                        frame #7 {
                          n1500 = Increment(x=w2275) -> (x+1=w2274:i32)
                          n1501 = property on="IV temp linear" class="XYGraph (strict)"("Active Plot"=w2275, "Plot.Plot Name"=w2276, "LegNumRows"=w2274) -> ()  [unwired: 2 in, 2 out]
                          n1502 = property on="IV temp log" class="XYGraph (strict)"("Active Plot"=w2275, "Plot.Plot Name"=w2276, "LegNumRows"=w2274) -> ()  [unwired: 2 in, 2 out]
                        }
                        frame #8 {
                          n1503 = local read "V fine"() -> (w2294:dbl[])
                          n1504 = local read "I fine"() -> (w2295:dbl[])
                          n1505 = local read "Parameters Flash"() -> (w2292:T5)
                          n1506 = local read "Wafer Info 3"() -> (w2283:T3)
                          n1507 = local read "Temp Data"() -> (w2284:T2)
                          n1508 = local read "Current Session"() -> (w2280:timestamp)
                          n1509 = local read "Operator"() -> (w2281:string)
                          n1510 = local read "RecipeID"() -> (w2282:string)
                          n1511 = Build Array(w2294, w2295) -> (w2293:dbl[][])
                          n1512 = Get Date/Time String(seconds (now)=w2290, want seconds? (F)=TRUE) -> (date string=w2289:string, time string=w2287:string)  [unwired: 1 in]
                          n1513 = local read "Mask"() -> (w2296:string)
                          n1514 = call <vilib>:"Space Constant.vi"() -> ("String"=w2286:string)
                          n1515 = Concatenate Strings(w2289, w2286, w2287) -> (w2285:string)
                          n1516 = call "WriteFlashFile NEW.vi"("Input File Path"=w2297, "IV array"=w2293, "Current Session"=w2280, "Parameters"=w2292, "RecipeID"=w2282, "User"=w2281, "Coords"=w2291, "Wafer Info"=w2283, "Mask Name"=w2296, "Temp Data"=w2284, "Die Number"=w2285) -> ()  [unwired: 16 in, 1 out]
                        }
                      }
                    }
                  }
                  "iteration" <- w2060
                }
              }
              frame #2 {
                w2310 = -1 ("x")
                n1517 = local read "Temptronics VISA"() -> (w2299:refnum<visa-resource-name>)
                n1518 = local read "Prober GPIB"() -> (w2306:string)
                n1519 = local read "current y"() -> (w2309:i32)
                n1520 = local read "current x"() -> (w2308:i32)
                n1521 = Multiply(x=w2309, y=w2310) -> (x*y=w2312:i32)
                n1522 = Multiply(x=w2310, y=w2308) -> (x*y=w2311:i32)
                n1523 = call "EG2001 Move Z Down.vi"("GPIB Address"=w2306) -> ("Error Out"=w2307:errorcluster, "GPIB Address Out"=w2305:string)  [unwired: 9 in]
                n1524 = VISA Write(VISA resource name=w2299, write buffer="rs25" ("string")) -> (VISA resource name out=w2300:refnum<visa-resource-name>)  [unwired: 1 in, 2 out]
                n1525 = VISA Write(VISA resource name=w2300, write buffer="st") -> (VISA resource name out=w2302:refnum<visa-resource-name>, return count=w2303:u32)  [unwired: 1 in, 1 out]
                n1526 = call "EG2001 Move Machine Step X-Y.vi"("Flip X Coordinates?"=FALSE, "Y"=w2312, "Steps/Microns"=enum32{"Steps", "Microns"}."Microns", "X"=w2311, "error in (no error)"=w2307, "GPIB Address"=w2305) -> ()  [unwired: 4 in, 2 out]
                n1527 = VISA Read(VISA resource name=w2302, byte count=w2303) -> (read buffer=w2304:string)  [unwired: 1 in, 3 out]
                n1528 = local write "Current Temp"(w2304) -> ()
              }
              frame #3 {
                w2316 = 0 ("current x")
                n1529 = local write "current y"(w2316) -> ()
                n1530 = local write "current x"(w2316) -> ()
                n1531 = local write "Status"("idle" ("Status")) -> ()
              }
            }
          }
          frame "add temp auto" {
            n1532 = local read "Auto Temp Set"() -> (w2321:dbl)
            n1533 = property on="Auto Temperature List" class="LstBox (strict)"() -> ("Item Names"=w2319:string[])  [unwired: 2 in, 2 out]
            n1534 = Format Into String(format string="%08.4f", w2321) -> (resulting string=w2318:string)  [unwired: 2 in, 1 out]
            n1535 = Build Array (concatenate)(w2319, w2318) -> (w2317:string[])
            n1536 = property on="Auto Temperature List" class="LstBox (strict)"("Item Names"=w2317) -> ()  [unwired: 2 in, 2 out]
          }
          frame "remove temp auto" {
            n1537 = local read "Auto Temperature List"() -> (w2324:i32)
            n1538 = property on="Auto Temperature List" class="LstBox (strict)"() -> ("Item Names"=w2326:string[])  [unwired: 2 in, 2 out]
            n1539 = Delete From Array(array=w2326, index=w2324) -> (array with subset deleted=w2325:string[])  [unwired: 1 in, 1 out]
            n1540 = property on="Auto Temperature List" class="LstBox (strict)"("Item Names"=w2325) -> ()  [unwired: 2 in, 2 out]
          }
          frame "clear temp auto" {
            n1541 = property on="Auto Temperature List" class="LstBox (strict)"("Item Names"=string[] []) -> ()  [unwired: 2 in, 2 out]
          }
          frame "explore data" {
          }
          frame "new session" {
            n1542 = Get Date/Time In Seconds() -> (seconds since 1Jan1904=w2335:timestamp)
            n1543 = local write "Current Session"(w2335) -> ()
            n1544 = local read "Session Info"() -> (w2336:T8)
            n1545 = Bundle By Name(cluster=w2336, "Session Time"=w2335) -> (w2334:T8)
            n1546 = local write "Session Info"(w2334) -> ()
          }
        }
      }
      n1547 = Release Queue(queue=w36, force destroy? (F)=TRUE, error in (no error)=w27) -> (error out=→"error out":errorcluster)  [unwired: 2 out]
    }
  }
